vi "TI cDAQ.vi"() -> ()   [LabVIEW 2023]
uses:
  Type Defs and Controls/Graphs Numerics.ctl
  Type Defs and Controls/Graph Channels.ctl
  Type Defs and Controls/Sensor List Cluster.ctl
  Type Defs and Controls/Channel Config Screen.ctl
  Type Defs and Controls/Graphs Numerics (Big).ctl
  Type Defs and Controls/Graph Channels (Big).ctl
  Type Defs and Controls/Sensor Config.ctl
  Type Defs and Controls/DAQ Settings.ctl
  Type Defs and Controls/Trigger Stop Method.ctl
  Type Defs and Controls/Log File Type.ctl
  Type Defs and Controls/Channel Config.ctl
  Type Defs and Controls/Header.ctl
  Type Defs and Controls/Graph Settings Type Def.ctl
  Type Defs and Controls/Test Limits.ctl
  Type Defs and Controls/All Part Info.ctl
  Type Defs and Controls/Part Info.ctl
  Type Defs and Controls/Sensor.ctl
  Type Defs and Controls/System Type.ctl
  Type Defs and Controls/System Config.ctl
  Type Defs and Controls/App Config.ctl
  <vilib>/event_ctls.llb/eventvkey.ctl
  <vilib>/Analysis/baseanly.llb/Mean (DBL).vi
  <vilib>/DAQmx/read.llb/DAQmx Read (Analog 2D DBL NChan NSamp).vi
  <vilib>/Utility/file.llb/Read Delimited Spreadsheet (string).vi
  <vilib>/DAQmx/miscellaneous.llb/DAQmx Fill In Error Info.vi
  <userlib>/_OpenG.lib/array/array.llb/Sort 1D Array (String)__ogtk.vi
  <userlib>/_OpenG.lib/array/array.llb/Sort 1D Array (I32)__ogtk.vi
  <vilib>/Analysis/NI_AALBase.lvlib
  Type Defs and Controls/RT FIFO Mode.ctl
  <resource>/objmgr/daqmx.rc
  <vilib>/Utility/config.llb/NI_LVConfig.lvlib
  <userlib>/_OpenG.lib/array/array.llb/openg_array.lvlib
  <userlib>/_OpenG.lib/variantconfig/variantconfig.llb/openg_variant_configuration_file.lvlib
panel:
  in  "Connecting Tab":enum32{"Page 1"}(tab)
  in  "Save":bool
  in  "Revert":bool
  in  "Open File":bool
  in  "Save Data As":bool
  in  "O-Scope Mode":bool
  in  "Limit:":dbl caption="Mb"
  in  "Auto Save":bool=TRUE
  out "Changes Latch":bool=TRUE
  in  "Title Bar":string
  out "In O-scope Mode":bool
  in  "Load Indicator Tab":enum32{"Page 1"}(tab)
  in  "Decoration Tab":enum32{"Page 1", "Page 2"}(tab)
  in  "Main Tab":enum32{" Main", "Configure"}(tab)
  in  "Show Big Data":bool
  in  "Big Data Tab":enum32{"Page 1", "Page 2"}(tab)
  out "Graph Channels (Big)":T1
  out "Graph Numerics (Big)":T2 {"Y1 RT 9" format="%_4f"; "Y1 RT 8" format="%_4f"; "Y1 RT 7" format="%_4f"; "Y1 RT 6" format="%_4f"; "Y1 RT 5" format="%_4f"; "Y1 RT 4" format="%_4f"; "Y1 RT 3" format="%_4f"; "Y1 RT 2" format="%_4f"}
  out "Graph Colors (Big)":T3={"Numeric Text.Colors:BG Color"=16711680, "Numeric Text.Colors:BG Color 2"=16711680, "Numeric Text.Colors:BG Color 3"=16711680, "Numeric Text.Colors:BG Color 4"=16711680, "Numeric Text.Colors:BG Color 5"=16711680, "Numeric Text.Colors:BG Color 6"=16711680, "Numeric Text.Colors:BG Color 7"=16711680, "Numeric Text.Colors:BG Color 8"=16711680}
  in  "Axis Toggle All":bool
  in  "Axis Toggles":T4
  out "Graph 2":sgl[][](graph)
  in  "Play":bool=TRUE
  in  "Pause":bool
  in  "Main Toggle":bool
  in  "Graph Toggles":T4
  out "Graph Numerics":T5 {"Y6 RT 3" format="%_4f"; "Y5 RT 3" format="%_4f"; "Y4 RT 3" format="%_4f"; "Y3 RT 3" format="%_4f"; "Y6 RT 2" format="%_4f"; "Y5 RT 2" format="%_4f"; "Y4 RT 2" format="%_4f"; "Y3 RT 2" format="%_4f"; "Y2 RT 2" format="%_4f"; "Y1 RT 2" format="%_4f"; "Y6 RT" format="%_4f"; "Y5 RT" format="%_4f"; "Y4 RT" format="%_4f"; "Y3 RT" format="%_4f"; "Y2 RT" format="%_4f"; "Y1 RT" format="%_4f"}
  in  "Graph Channels":T6 {"Y5 3" items=["", "diag raw", "9221_AI-02", "9221_AI-03", "9221_AI-04", "9221_AI-05", "9221_AI-06", "9221_AI-07", "FDM Current (Controller)", "PWM Command", "PWM Diagnostic", "Pump Speed", "9205_AI-04", "9205_AI-05", "9205_AI-06", "9205_AI-07", "9205_AI-22A", "9205_AI-23A", "9208_AI-00", "9208_AI-01", "9208_AI-02", "9208_AI-03", "9208_AI-04", "9208_AI-05", "9208_AI-06", "9208_AI-07", "9211-1_TC-00", "9211-1_TC-01", "9211-1_TC-02", "9211-1_TC-03", "9211-2_TC-00", "9211-2_TC-01", "9211-2_TC-02", "9211-2_TC-03"]; "Y6 3" items=["", "diag raw", "9221_AI-02", "9221_AI-03", "9221_AI-04", "9221_AI-05", "9221_AI-06", "9221_AI-07", "FDM Current (Controller)", "PWM Command", "PWM Diagnostic", "Pump Speed", "9205_AI-04", "9205_AI-05", "9205_AI-06", "9205_AI-07", "9205_AI-22A", "9205_AI-23A", "9208_AI-00", "9208_AI-01", "9208_AI-02", "9208_AI-03", "9208_AI-04", "9208_AI-05", "9208_AI-06", "9208_AI-07", "9211-1_TC-00", "9211-1_TC-01", "9211-1_TC-02", "9211-1_TC-03", "9211-2_TC-00", "9211-2_TC-01", "9211-2_TC-02", "9211-2_TC-03"]; "Y3 3" items=["", "diag raw", "9221_AI-02", "9221_AI-03", "9221_AI-04", "9221_AI-05", "9221_AI-06", "9221_AI-07", "FDM Current (Controller)", "PWM Command", "PWM Diagnostic", "Pump Speed", "9205_AI-04", "9205_AI-05", "9205_AI-06", "9205_AI-07", "9205_AI-22A", "9205_AI-23A", "9208_AI-00", "9208_AI-01", "9208_AI-02", "9208_AI-03", "9208_AI-04", "9208_AI-05", "9208_AI-06", "9208_AI-07", "9211-1_TC-00", "9211-1_TC-01", "9211-1_TC-02", "9211-1_TC-03", "9211-2_TC-00", "9211-2_TC-01", "9211-2_TC-02", "9211-2_TC-03"]; "Y4 3" items=["", "diag raw", "9221_AI-02", "9221_AI-03", "9221_AI-04", "9221_AI-05", "9221_AI-06", "9221_AI-07", "FDM Current (Controller)", "PWM Command", "PWM Diagnostic", "Pump Speed", "9205_AI-04", "9205_AI-05", "9205_AI-06", "9205_AI-07", "9205_AI-22A", "9205_AI-23A", "9208_AI-00", "9208_AI-01", "9208_AI-02", "9208_AI-03", "9208_AI-04", "9208_AI-05", "9208_AI-06", "9208_AI-07", "9211-1_TC-00", "9211-1_TC-01", "9211-1_TC-02", "9211-1_TC-03", "9211-2_TC-00", "9211-2_TC-01", "9211-2_TC-02", "9211-2_TC-03"]; "Y5 2" items=["", "diag raw", "9221_AI-02", "9221_AI-03", "9221_AI-04", "9221_AI-05", "9221_AI-06", "9221_AI-07", "FDM Current (Controller)", "PWM Command", "PWM Diagnostic", "Pump Speed", "9205_AI-04", "9205_AI-05", "9205_AI-06", "9205_AI-07", "9205_AI-22A", "9205_AI-23A", "9208_AI-00", "9208_AI-01", "9208_AI-02", "9208_AI-03", "9208_AI-04", "9208_AI-05", "9208_AI-06", "9208_AI-07", "9211-1_TC-00", "9211-1_TC-01", "9211-1_TC-02", "9211-1_TC-03", "9211-2_TC-00", "9211-2_TC-01", "9211-2_TC-02", "9211-2_TC-03"]; "Y6 2" items=["", "diag raw", "9221_AI-02", "9221_AI-03", "9221_AI-04", "9221_AI-05", "9221_AI-06", "9221_AI-07", "FDM Current (Controller)", "PWM Command", "PWM Diagnostic", "Pump Speed", "9205_AI-04", "9205_AI-05", "9205_AI-06", "9205_AI-07", "9205_AI-22A", "9205_AI-23A", "9208_AI-00", "9208_AI-01", "9208_AI-02", "9208_AI-03", "9208_AI-04", "9208_AI-05", "9208_AI-06", "9208_AI-07", "9211-1_TC-00", "9211-1_TC-01", "9211-1_TC-02", "9211-1_TC-03", "9211-2_TC-00", "9211-2_TC-01", "9211-2_TC-02", "9211-2_TC-03"]; "Y3 2" items=["", "diag raw", "9221_AI-02", "9221_AI-03", "9221_AI-04", "9221_AI-05", "9221_AI-06", "9221_AI-07", "FDM Current (Controller)", "PWM Command", "PWM Diagnostic", "Pump Speed", "9205_AI-04", "9205_AI-05", "9205_AI-06", "9205_AI-07", "9205_AI-22A", "9205_AI-23A", "9208_AI-00", "9208_AI-01", "9208_AI-02", "9208_AI-03", "9208_AI-04", "9208_AI-05", "9208_AI-06", "9208_AI-07", "9211-1_TC-00", "9211-1_TC-01", "9211-1_TC-02", "9211-1_TC-03", "9211-2_TC-00", "9211-2_TC-01", "9211-2_TC-02", "9211-2_TC-03"]; "Y4 2" items=["", "diag raw", "9221_AI-02", "9221_AI-03", "9221_AI-04", "9221_AI-05", "9221_AI-06", "9221_AI-07", "FDM Current (Controller)", "PWM Command", "PWM Diagnostic", "Pump Speed", "9205_AI-04", "9205_AI-05", "9205_AI-06", "9205_AI-07", "9205_AI-22A", "9205_AI-23A", "9208_AI-00", "9208_AI-01", "9208_AI-02", "9208_AI-03", "9208_AI-04", "9208_AI-05", "9208_AI-06", "9208_AI-07", "9211-1_TC-00", "9211-1_TC-01", "9211-1_TC-02", "9211-1_TC-03", "9211-2_TC-00", "9211-2_TC-01", "9211-2_TC-02", "9211-2_TC-03"]; "Y2 2" items=["", "diag raw", "9221_AI-02", "9221_AI-03", "9221_AI-04", "9221_AI-05", "9221_AI-06", "9221_AI-07", "FDM Current (Controller)", "PWM Command", "PWM Diagnostic", "Pump Speed", "9205_AI-04", "9205_AI-05", "9205_AI-06", "9205_AI-07", "9205_AI-22A", "9205_AI-23A", "9208_AI-00", "9208_AI-01", "9208_AI-02", "9208_AI-03", "9208_AI-04", "9208_AI-05", "9208_AI-06", "9208_AI-07", "9211-1_TC-00", "9211-1_TC-01", "9211-1_TC-02", "9211-1_TC-03", "9211-2_TC-00", "9211-2_TC-01", "9211-2_TC-02", "9211-2_TC-03"]; "Y1 2" items=["", "diag raw", "9221_AI-02", "9221_AI-03", "9221_AI-04", "9221_AI-05", "9221_AI-06", "9221_AI-07", "FDM Current (Controller)", "PWM Command", "PWM Diagnostic", "Pump Speed", "9205_AI-04", "9205_AI-05", "9205_AI-06", "9205_AI-07", "9205_AI-22A", "9205_AI-23A", "9208_AI-00", "9208_AI-01", "9208_AI-02", "9208_AI-03", "9208_AI-04", "9208_AI-05", "9208_AI-06", "9208_AI-07", "9211-1_TC-00", "9211-1_TC-01", "9211-1_TC-02", "9211-1_TC-03", "9211-2_TC-00", "9211-2_TC-01", "9211-2_TC-02", "9211-2_TC-03"]}
  in  "Graph Range":T7(ring)=enum."10"
  out "Graph 1":sgl[][](graph)
  in  "Synch Files":bool
  in  "Import from CSV":bool
  in  "Log Min":bool
  in  "Log Sec":bool=TRUE
  in  "Hide Trig Ch":bool
  in  "Hide Trig Val":bool
  in  "Hide Trig Samples":bool
  in  "Hide Trig Stop":bool
  in  "Hide Trig Int":bool
  in  "Hide Pretrig Smpls":bool
  in  "Save Mode":T8(ring)
  in  "Sample Min":bool
  in  "Sample Sec":bool=TRUE
  in  "Delete Sensor":bool
  in  "Add Sensor":bool
  in  "Trigger Stop Method":T9(ring)=enum."Use Threshold to Stop Trigger"
  in  "Hours":bool
  in  "Minutes":bool=TRUE
  in  "Trigger Type":T10(ring)
  in  "Sensors":T11=[{"Channel"="9221_AI-00", "Description"="test", "Acquire"=TRUE, "Sensor"="Pressure Sensor", "Chg Sensor"=FALSE, "Cal Date"="12/31/1903", "Offset"=-0.0, "Span"=10.0, "Cal"=FALSE, "Test Limits"=FALSE, "Type"="0-60 VDC", "Data Index"=0}, {"Channel"="9221_AI-01", "Description"="", "Acquire"=FALSE, "Sensor"="None Selected", "Chg Sensor"=FALSE, "Cal Date"="---------", "Offset"=0.0, "Span"=0.0, "Cal"=FALSE, "Test Limits"=FALSE, "Type"="0-60 VDC", "Data Index"=1}, {"Channel"="9221_AI-02", "Description"="", "Acquire"=FALSE, "Sensor"="None Selected", "Chg Sensor"=FALSE, "Cal Date"="---------", "Offset"=0.0, "Span"=0.0, "Cal"=FALSE, "Test Limits"=FALSE, "Type"="0-60 VDC", "Data Index"=2}, {"Channel"="9221_AI-03", "Description"="", "Acquire"=FALSE, "Sensor"="None Selected", "Chg Sensor"=FALSE, "Cal Date"="---------", "Offset"=0.0, "Span"=0.0, "Cal"=FALSE, "Test Limits"=FALSE, "Type"="0-60 VDC", "Data Index"=3}, {"Channel"="9221_AI-04", "Description"="", "Acquire"=FALSE, "Sensor"="None Selected", "Chg Sensor"=FALSE, "Cal Date"="---------", "Offset"=0.0, "Span"=0.0, "Cal"=FALSE, "Test Limits"=FALSE, "Type"="0-60 VDC", "Data Index"=4}, {"Channel"="9221_AI-05", "Description"="", "Acquire"=FALSE, "Sensor"="None Selected", "Chg Sensor"=FALSE, "Cal Date"="---------", "Offset"=0.0, "Span"=0.0, "Cal"=FALSE, "Test Limits"=FALSE, "Type"="0-60 VDC", "Data Index"=5}, {"Channel"="9221_AI-06", "Description"="", "Acquire"=FALSE, "Sensor"="None Selected", "Chg Sensor"=FALSE, "Cal Date"="---------", "Offset"=0.0, "Span"=0.0, "Cal"=FALSE, "Test Limits"=FALSE, "Type"="0-60 VDC", "Data Index"=6}, {"Channel"="9221_AI-07", "Description"="", "Acquire"=FALSE, "Sensor"="None Selected", "Chg Sensor"=FALSE, "Cal Date"="---------", "Offset"=0.0, "Span"=0.0, "Cal"=FALSE, "Test Limits"=FALSE, "Type"="0-60 VDC", "Data Index"=7}, {"Channel"="9205_AI-00", "Description"="", "Acquire"=FALSE, "Sensor"="None Selected", "Chg Sensor"=FALSE, "Cal Date"="---------", "Offset"=0.0, "Span"=0.0, "Cal"=FALSE, "Test Limits"=FALSE, "Type"="0-10 VDC", "Data Index"=8}, {"Channel"="9205_AI-01", "Description"="", "Acquire"=FALSE, "Sensor"="None Selected", "Chg Sensor"=FALSE, "Cal Date"="---------", "Offset"=0.0, "Span"=0.0, "Cal"=FALSE, "Test Limits"=FALSE, "Type"="0-10 VDC", "Data Index"=9}, {"Channel"="9205_AI-02", "Description"="", "Acquire"=FALSE, "Sensor"="None Selected", "Chg Sensor"=FALSE, "Cal Date"="---------", "Offset"=0.0, "Span"=0.0, "Cal"=FALSE, "Test Limits"=FALSE, "Type"="0-10 VDC", "Data Index"=10}, {"Channel"="9205_AI-03", "Description"="", "Acquire"=FALSE, "Sensor"="None Selected", "Chg Sensor"=FALSE, "Cal Date"="---------", "Offset"=0.0, "Span"=0.0, "Cal"=FALSE, "Test Limits"=FALSE, "Type"="0-10 VDC", "Data Index"=11}, {"Channel"="9205_AI-04", "Description"="", "Acquire"=FALSE, "Sensor"="None Selected", "Chg Sensor"=FALSE, "Cal Date"="---------", "Offset"=0.0, "Span"=0.0, "Cal"=FALSE, "Test Limits"=FALSE, "Type"="0-10 VDC", "Data Index"=12}, {"Channel"="9205_AI-05", "Description"="", "Acquire"=FALSE, "Sensor"="None Selected", "Chg Sensor"=FALSE, "Cal Date"="---------", "Offset"=0.0, "Span"=0.0, "Cal"=FALSE, "Test Limits"=FALSE, "Type"="0-10 VDC", "Data Index"=13}, {"Channel"="9205_AI-06", "Description"="", "Acquire"=FALSE, "Sensor"="None Selected", "Chg Sensor"=FALSE, "Cal Date"="---------", "Offset"=0.0, "Span"=0.0, "Cal"=FALSE, "Test Limits"=FALSE, "Type"="0-10 VDC", "Data Index"=14}, {"Channel"="9205_AI-07", "Description"="", "Acquire"=FALSE, "Sensor"="None Selected", "Chg Sensor"=FALSE, "Cal Date"="---------", "Offset"=0.0, "Span"=0.0, "Cal"=FALSE, "Test Limits"=FALSE, "Type"="0-10 VDC", "Data Index"=15}, {"Channel"="9208_AI-00", "Description"="", "Acquire"=FALSE, "Sensor"="None Selected", "Chg Sensor"=FALSE, "Cal Date"="---------", "Offset"=0.0, "Span"=0.0, "Cal"=FALSE, "Test Limits"=FALSE, "Type"="0-20 mA", "Data Index"=16}, {"Channel"="9208_AI-01", "Description"="", "Acquire"=FALSE, "Sensor"="None Selected", "Chg Sensor"=FALSE, "Cal Date"="---------", "Offset"=0.0, "Span"=0.0, "Cal"=FALSE, "Test Limits"=FALSE, "Type"="0-20 mA", "Data Index"=17}, {"Channel"="9208_AI-02", "Description"="", "Acquire"=FALSE, "Sensor"="None Selected", "Chg Sensor"=FALSE, "Cal Date"="---------", "Offset"=0.0, "Span"=0.0, "Cal"=FALSE, "Test Limits"=FALSE, "Type"="0-20 mA", "Data Index"=18}, {"Channel"="9208_AI-03", "Description"="", "Acquire"=FALSE, "Sensor"="None Selected", "Chg Sensor"=FALSE, "Cal Date"="---------", "Offset"=0.0, "Span"=0.0, "Cal"=FALSE, "Test Limits"=FALSE, "Type"="0-20 mA", "Data Index"=19}, {"Channel"="9208_AI-04", "Description"="", "Acquire"=FALSE, "Sensor"="None Selected", "Chg Sensor"=FALSE, "Cal Date"="---------", "Offset"=0.0, "Span"=0.0, "Cal"=FALSE, "Test Limits"=FALSE, "Type"="0-20 mA", "Data Index"=20}, {"Channel"="9208_AI-05", "Description"="", "Acquire"=FALSE, "Sensor"="None Selected", "Chg Sensor"=FALSE, "Cal Date"="---------", "Offset"=0.0, "Span"=0.0, "Cal"=FALSE, "Test Limits"=FALSE, "Type"="0-20 mA", "Data Index"=21}, {"Channel"="9208_AI-06", "Description"="", "Acquire"=FALSE, "Sensor"="None Selected", "Chg Sensor"=FALSE, "Cal Date"="---------", "Offset"=0.0, "Span"=0.0, "Cal"=FALSE, "Test Limits"=FALSE, "Type"="0-20 mA", "Data Index"=22}, {"Channel"="9208_AI-07", "Description"="", "Acquire"=FALSE, "Sensor"="None Selected", "Chg Sensor"=FALSE, "Cal Date"="---------", "Offset"=0.0, "Span"=0.0, "Cal"=FALSE, "Test Limits"=FALSE, "Type"="0-20 mA", "Data Index"=23}, {"Channel"="9211_TC-00", "Description"="", "Acquire"=FALSE, "Sensor"="None Selected", "Chg Sensor"=FALSE, "Cal Date"="---------", "Offset"=0.0, "Span"=0.0, "Cal"=FALSE, "Test Limits"=FALSE, "Type"="T-Type", "Data Index"=24}, {"Channel"="9211_TC-01", "Description"="", "Acquire"=FALSE, "Sensor"="None Selected", "Chg Sensor"=FALSE, "Cal Date"="---------", "Offset"=0.0, "Span"=0.0, "Cal"=FALSE, "Test Limits"=FALSE, "Type"="T-Type", "Data Index"=25}, {"Channel"="9211_TC-02", "Description"="", "Acquire"=FALSE, "Sensor"="None Selected", "Chg Sensor"=FALSE, "Cal Date"="---------", "Offset"=0.0, "Span"=0.0, "Cal"=FALSE, "Test Limits"=FALSE, "Type"="T-Type", "Data Index"=26}, {"Channel"="9211_TC-03", "Description"="", "Acquire"=FALSE, "Sensor"="None Selected", "Chg Sensor"=FALSE, "Cal Date"="---------", "Offset"=0.0, "Span"=0.0, "Cal"=FALSE, "Test Limits"=FALSE, "Type"="T-Type", "Data Index"=27}]
  in  "DAQ Table":string[][](table)=[[""], ["test"], ["50.000"], ["5"], ["0"], ["1.000"], [""], ["10"], ["1"]]
  out "Config Name:":string="test.cfg"
  in  "Open":bool
  in  "Save As":bool
  in  "Title Tab":enum32{"Page 1", "Page 2"}(tab)
  out "Title":string="TI cDAQ, Debug"
  out "Date":string="4/23/2020"
  out "Time":string="11:18:09 AM"
  in  "Mode Exit":bool
  out "Status":string="IN DATA VIEW MODE..."
  in  "Acquiring Tab":enum32{"Page 1"}(tab)
  in  "Control Tab":enum32{"Page 1", "Page 2"}(tab)
  in  "Disarm DAQ":bool
  in  "Arm DAQ":bool
  out "DAQ Armed":bool
  in  "Start Log":bool
  out "Acquiring Data 2":bool
  in  "Stop DAQ":bool
  in  "Header Table:":string[][](table)=[[""], [""], [""], [""]] caption="Header Table"
  in  "Data Base Path:":path=path "C:/Data"
  out "Elapsed Time:":dbl format="%<%H:%M:%S>t"
  out "Start of Test:":timestamp format="%<%x %X>T"
  out "Samples Recorded:":u32 format="%#.0f"
  in  "Add Data Point":bool
  # "Connecting\nto cDAQ"
  # "samples /"
  # "*This includes the Sensor/Cal file,\nand Config files."
  # "samples /"
  # "Channel"
  # "Type"
  # "Acquire"
  # "Name"
  # "Sensor"
  # "Cal Date"
  # "Zero"
  # "Span"
  # "Logging\nData"
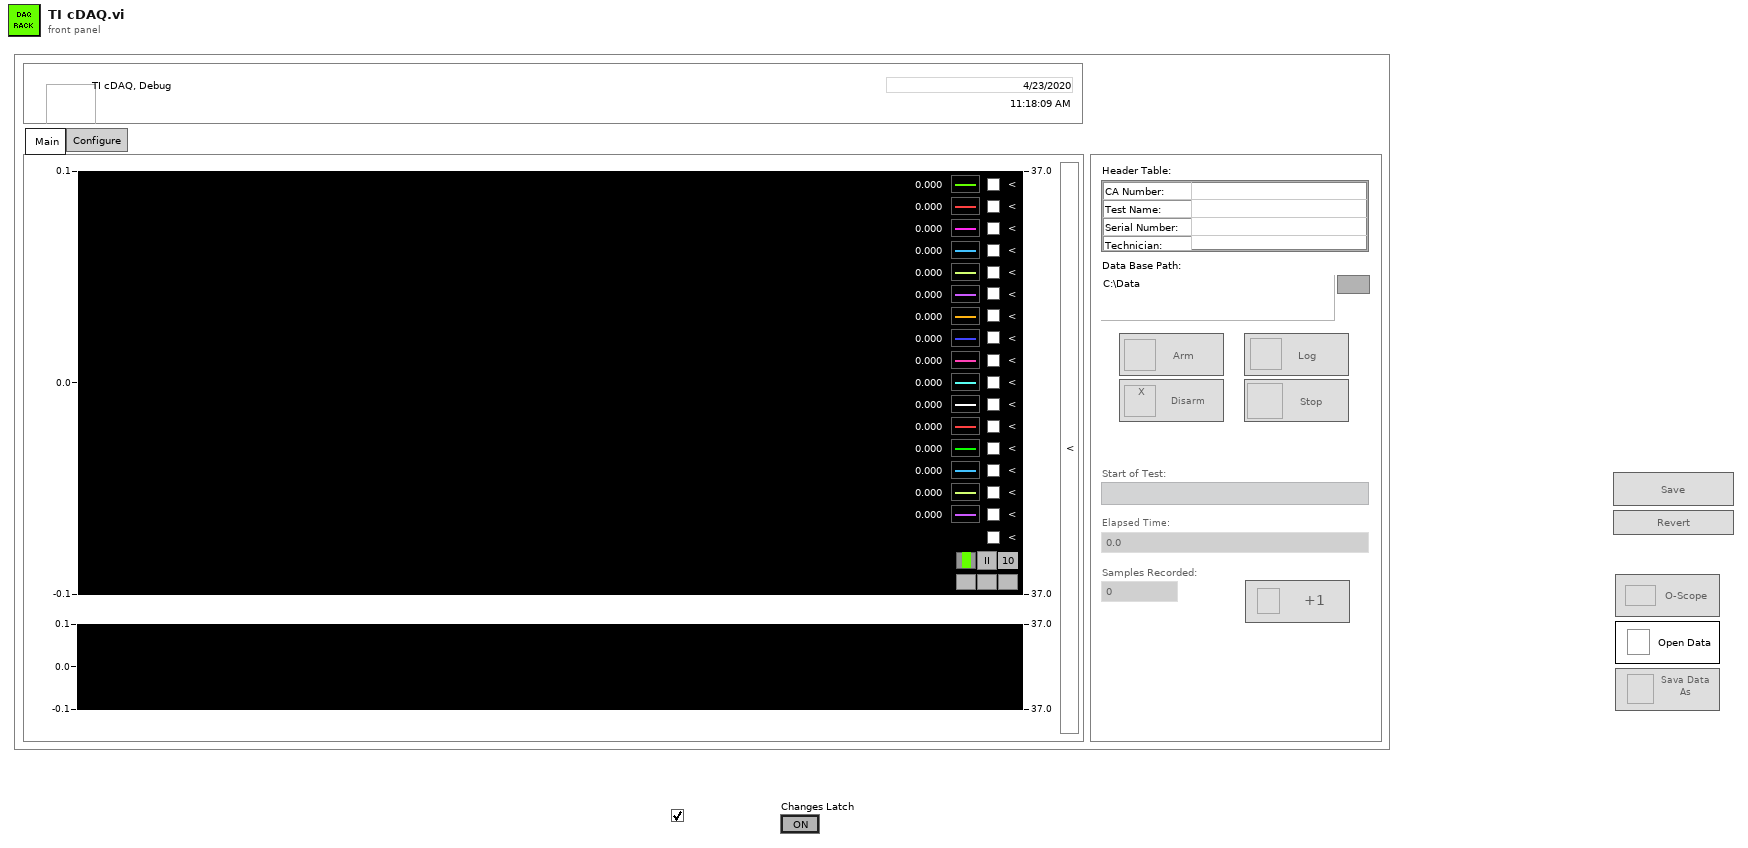
[diagram p1: front panel]
types:
  T1 = typedef "Graph Channels (Big).ctl" = cluster{"String":string, "String 2":string, "String 3":string, "String 4":string, "String 5":string, "String 6":string, "String 7":string, "String 8":string}
  T2 = typedef "Graphs Numerics (Big).ctl" = cluster{"Y1 RT 2":dbl, "Y1 RT 3":dbl, "Y1 RT 4":dbl, "Y1 RT 5":dbl, "Y1 RT 6":dbl, "Y1 RT 7":dbl, "Y1 RT 8":dbl, "Y1 RT 9":dbl}
  T3 = cluster{"Numeric Text.Colors:BG Color":u32, "Numeric Text.Colors:BG Color 2":u32, "Numeric Text.Colors:BG Color 3":u32, "Numeric Text.Colors:BG Color 4":u32, "Numeric Text.Colors:BG Color 5":u32, "Numeric Text.Colors:BG Color 6":u32, "Numeric Text.Colors:BG Color 7":u32, "Numeric Text.Colors:BG Color 8":u32}
  T4 = cluster{"Boolean":bool, "Boolean 2":bool, "Boolean 3":bool, "Boolean 4":bool, "Boolean 5":bool, "Boolean 6":bool, "Boolean 7":bool, "Boolean 8":bool, "Boolean 9":bool, "Boolean 10":bool, "Boolean 11":bool, "Boolean 12":bool, "Boolean 13":bool, "Boolean 14":bool, "Boolean 15":bool, "Boolean 16":bool}
  T5 = typedef "Graphs Numerics.ctl" = cluster{"Y1 RT":dbl, "Y2 RT":dbl, "Y3 RT":dbl, "Y4 RT":dbl, "Y5 RT":dbl, "Y6 RT":dbl, "Y1 RT 2":dbl, "Y2 RT 2":dbl, "Y3 RT 2":dbl, "Y4 RT 2":dbl, "Y5 RT 2":dbl, "Y6 RT 2":dbl, "Y3 RT 3":dbl, "Y4 RT 3":dbl, "Y5 RT 3":dbl, "Y6 RT 3":dbl}
  T6 = typedef "Graph Channels.ctl" = cluster{"Y1":u16, "Y2":u16, "Y3":u16, "Y4":u16, "Y5":u16, "Y6":u16, "Y1 2":u16, "Y2 2":u16, "Y3 2":u16, "Y4 2":u16, "Y5 2":u16, "Y6 2":u16, "Y3 3":u16, "Y4 3":u16, "Y5 3":u16, "Y6 3":u16}
  T7 = enum16{"1", "2", "3", "4", "5", "10", "15", "30", "60"}
  T8 = enum16{"Single File", "Segmented Files", "New File at Midnight"}
  T9 = enum16{"Use Samples Value to Stop Trigger", "Use Threshold to Stop Trigger"}
  T10 = enum16{"Manual", "Timed", "Analog Rising", "Analog Falling"}
  T11 = typedef "Sensor List Cluster.ctl" = T12[]
  T12 = typedef "Channel Config Screen.ctl" = cluster{"Channel":string, "Description":string, "Acquire":bool, "Sensor":string, "Chg Sensor":bool, "Cal Date":string, "Offset":dbl, "Span":dbl, "Cal":bool, "Test Limits":bool, "Type":string, "Data Index":u32}
  T13 = typedef "App Config.ctl" = cluster{"Support Dir (Local)":path, "Support Dir (Remote)":path, "Config Sub Dir":string, "Last Config (Std)":string, "Last Config (Def)":string, "Last Config (8TC)":string}
  T14 = typedef "System Config.ctl" = cluster{"System":string, "Description":string}
  T15 = typedef "System Type.ctl" = enum16{"Standard", "Deformation", "Standard 8TC"}
  T16 = typedef "Sensor Config.ctl" = cluster{"DAQ Settings":T17, "Channels":T20[], "Header":T21, "Graph Settings":T22, "Test Limits":T23[], "All Type Info":T24, "Save Mode":enum16{"Single File", "Segmented Files", "New File at Midnight"}, "Data Base Path":path}
  T17 = typedef "DAQ Settings.ctl" = cluster{"Trigger Type":enum16{"Manual", "Timed", "Analog Rising", "Analog Falling"}, "Trigger Samples":i32, "Pretrigger Samples":i32, "Trigger Interval":dbl, "Time Units":bool, "Auto Save":bool, "Sample Rate":dbl, "Select Analog":bool, "Trigger Value":dbl, "Trigger Stop Method":T18, "Rate Sec/Min":bool, "Save Mode":enum16{"Single File", "Segmented Files", "New File at Midnight"}, "File Size Limit":dbl, "Log File Type":T19, "Trigger Data Index":u32, "Log Rate":dbl, "Rate Sec/Min (Log)":bool, "Sample Rate (S/s)":dbl, "Log Rate (S/s)":dbl}
  T18 = typedef "Trigger Stop Method.ctl" = enum16{"Use Samples Value to Stop Trigger", "Use Threshold to Stop Trigger"}
  T19 = typedef "Log File Type.ctl" = enum16{"Basic", "RTS"}
  T20 = typedef "Channel Config.ctl" = cluster{"Channel":string, "Type":string, "Acquire":bool, "Name":string, "Sensor":string, "Data Index":u32}
  T21 = typedef "Header.ctl" = cluster{"CA Number":string, "Test Name":string, "Serial Number":string, "Technician":string}
  T22 = typedef "Graph Settings Type Def.ctl" = cluster{"Graph Labels":string[], u8[], i16[], u32[], u8[], u8[], u8[], u32[], u8[], u8[], u8[], dbl[], dbl[], "Graph Toggles":bool[], "Axis Toggles":bool[], "Graph Range":enum16{"1", "2", "3", "4", "5", "10", "15", "30", "60"}}
  T23 = typedef "Test Limits.ctl" = cluster{"Channel Acquired?":bool, "RMS?":bool, "Pk-Pk":bool, "Frequency":bool, "EU High Limit 1":dbl, "EU Low Limit 1":dbl, "EU High Limit 2":dbl, "EU Low Limit 2":dbl, "RMS High Limit":dbl, "RMS Low Limit":dbl, "Pk-Pk High Limit ":dbl, "Pk-Pk Low Limit":dbl, "Frequency High Limit":dbl, "Frequency Low Limit":dbl}
  T24 = typedef "All Part Info.ctl" = cluster{"Type Name":string, "Type Signal Names":string[], "# Signals":i32, "# Parts":i32, "Part Info":T25[]}[]
  T25 = typedef "Part Info.ctl" = cluster{"Part Number":string, "Channel Indexes":u16[], "Enabled?":bool}
  T26 = typedef "Sensor.ctl" = cluster{"Sensor Name":string, "Sensor Info":cluster{"Manufacturer":string, "Model":string, "Serial Number":string}, "Last Cal Info":cluster{"Last Calibration Date":dbl, "Calibrator":string, "Cal Duration":i32}, "Voltage Range":cluster{"High Limit":dbl, "Low Limit":dbl}, "EGU Range":cluster{"High Limit":dbl, "Low Limit":dbl}, "Units":string, "Calibration Type":enum16{"Calibrate Analog", "Compare Analog Calibration"}, "EGU List":dbl[], "Voltage List":dbl[], "Coefficients":dbl[], "Order":i32, "Algorithm":enum32{"SVD", "Givens", "Givens2", "Householder", "LU Decomposition", "Cholesky"}, "Max Error % of Full Scale":dbl, "Max Mean Squared Error":dbl, "Use Error %":bool, "Use MSE":bool, "Allow Manual Entry":bool, "Max Stability Error":dbl, "Max Error % of Reading":dbl, "Use Error % of Reading":bool}
  T27 = cluster{"Sensor Name":string, "Sensor Info":cluster{"Manufacturer":string, "Model":string, "Serial Number":string}, "Last Cal Info":cluster{"Last Calibration Date":dbl, "Calibrator":string, "Cal Duration":i32}, "Voltage Range":cluster{"High Limit":dbl, "Low Limit":dbl}, "EGU Range":cluster{"High Limit":dbl, "Low Limit":dbl}, "Units":string, "Calibration Type":enum16{"Calibrate Analog", "Compare Analog Calibration"}, "EGU List":dbl[], "Voltage List":dbl[], "Coefficients":dbl[], "Order":i32, "Algorithm":enum32{"SVD", "Givens", "Givens2", "Householder", "LU Decomposition", "Cholesky"}, "Max Error % of Full Scale":dbl, "Max Mean Squared Error":dbl, "Use Error %":bool, "Use MSE":bool, "Allow Manual Entry":bool, "Max Stability Error":dbl, "Max Error % of Reading":dbl, "Use Error % of Reading":bool}[]
  T28 = cluster{"Virtual Trigger":bool, "Interval":dbl, "Trigger Armed":bool, "Acquiring Data":bool, "Channel Filter":bool[], "Error":errorcluster, "Data":sgl[][], "Trigger Index":i32, "App Path":path, "Config Dir":path, "Config":T16, "Channel Addresses":string[], "Scaling":cluster{"Sensor Name":string, "Sensor Info":cluster{"Manufacturer":string, "Model":string, "Serial Number":string}, "Last Cal Info":cluster{"Last Calibration Date":dbl, "Calibrator":string, "Cal Duration":i32}, "Voltage Range":cluster{"High Limit":dbl, "Low Limit":dbl}, "EGU Range":cluster{"High Limit":dbl, "Low Limit":dbl}, "Units":string, "Calibration Type":enum16{"Calibrate Analog", "Compare Analog Calibration"}, "EGU List":dbl[], "Voltage List":dbl[], "Coefficients":dbl[], "Order":i32, "Algorithm":enum32{"SVD", "Givens", "Givens2", "Householder", "LU Decomposition", "Cholesky"}, "Max Error % of Full Scale":dbl, "Max Mean Squared Error":dbl, "Use Error %":bool, "Use MSE":bool, "Allow Manual Entry":bool, "Max Stability Error":dbl, "Max Error % of Reading":dbl, "Use Error % of Reading":bool}[], "File Created?":bool, "Saving Path":path, "Previous Time":dbl, "New Time":dbl, "Calibration Path":path, "AI Task":refnum<k21>, "Graph Ch Refs":refnum<vi>[], "Pause Graph":bool, "Force Update":bool, "Data File Path":path, "Buffer Size":u32, "UnPause Once":bool, "O-Scope Mode":bool, "Data View Mode":bool, "Midnight Check":timestamp, "Start Timestamp":timestamp, "Time Offset":dbl, "Pretrigger Size":i32, "Midnight Rollover":bool, "Segment File":bool, "Total Channel Count":i16, "DO Task":refnum<k21>, "DI Task":refnum<k21>, "timer":u32, "App Config Path":path, "Title Bar":refnum<vi>, "Connected Timer":u32, "Last SN":string, "Acquire Data":bool, "Channel Select":i32, "Channel Display":T11, "Sensors":T26[], "Config Saved":T16, "Changes?":bool, "Revert":bool, "DAQ Running":bool, "Load Prompt":bool, "Samples Recorded":u32, "System Type":T15, "Samples Acquired":u32, "Data Log Indicies":i32[], "System Ref":tag, "Selected System":T14, "Config Extension":string, "App Config":T13, "Config Name":string, "Sensor File Name":string, "Sys Cfg File Name":string, "Add Data Point":bool, "Manual Data Mode":bool, "Log Path Ref":refnum<file>}
  T29 = typedef "eventvkey.ctl" = enum16{"ASCII", "Enter", "Return", "Shift", "Ctrl", "Alt", "Cmd", "Opt", "Caps", "NumLock", "Clear", "Break", "Up", "Down", "Left", "Right", "Insert", "Delete", "Home", "End", "PageUp", "PageDown", "Escape", "Help", "Pause", "ScrollLock", "F1", "F2", "F3", "F4", "F5", "F6", "F7", "F8", "F9", "F10", "F11", "F12", "F13", "F14", "F15", "F16", "F17", "F18", "F19", "F20", "F21", "F22", "F23", "F24", "Play", "VolumeUp", "VolumeDown", "Mute", "Two Byte Char"}
  T30 = enum8{"Enabled", "Disabled", "Disabled and Grayed Out"}
  T31 = enum32{"Page Enabled", "Page Disabled", "Page Disabled & Grayed"}
  T32 = typedef "RT FIFO Mode.ctl" = enum16{"Create", "Write", "Read", "Delete"}
  T33 = cluster{"[0]":bool, "[1]":bool, "[2]":bool, "[3]":bool, "[4]":bool, "[5]":bool, "[6]":bool, "[7]":bool, "[8]":bool, "[9]":bool, "[10]":bool, "[11]":bool, "[12]":bool, "[13]":bool, "[14]":bool, "[15]":bool}
  T34 = typedef "LVRowAndColumnTypeDef.ctl" = cluster{"Row":i32, "Column":i32}
  T35 = cluster{"Header Table:[0]":string, "Header Table:[1]":string, "Header Table:[2]":string, "Header Table:[3]":string}
  T36 = typedef "LVPoint32TypeDef.ctl" = cluster{"Horizontal":i32, "Vertical":i32}
  T37 = cluster{"[0]":string, "[1]":string, "[2]":string, "[3]":string, "[4]":string, "[5]":string, "[6]":string, "[7]":string}
  T38 = enum32{"invalid app kind", "Development System", "Run Time System", "Student Edition", "Embedded LabVIEW", "Evaluation", "Custom"}
  T39 = typedef "NI_LVConfig.lvlib/Config Data RefNum.ctl" = refnum<k1>
  T40 = cluster{"[0]":dbl, "[1]":dbl, "[2]":dbl, "[3]":dbl, "[4]":dbl, "[5]":dbl, "[6]":dbl, "[7]":dbl, "[8]":dbl, "[9]":dbl, "[10]":dbl, "[11]":dbl, "[12]":dbl, "[13]":dbl, "[14]":dbl, "[15]":dbl}
  T41 = cluster{"[0]":dbl, "[1]":dbl, "[2]":dbl, "[3]":dbl, "[4]":dbl, "[5]":dbl, "[6]":dbl, "[7]":dbl}
  T42 = cluster{"Graph Toggles[0]":bool, "Graph Toggles[1]":bool, "Graph Toggles[2]":bool, "Graph Toggles[3]":bool, "Graph Toggles[4]":bool, "Graph Toggles[5]":bool, "Graph Toggles[6]":bool, "Graph Toggles[7]":bool, "Graph Toggles[8]":bool, "Graph Toggles[9]":bool, "Graph Toggles[10]":bool, "Graph Toggles[11]":bool, "Graph Toggles[12]":bool, "Graph Toggles[13]":bool, "Graph Toggles[14]":bool, "Graph Toggles[15]":bool}
  T43 = cluster{"Axis Toggles[0]":bool, "Axis Toggles[1]":bool, "Axis Toggles[2]":bool, "Axis Toggles[3]":bool, "Axis Toggles[4]":bool, "Axis Toggles[5]":bool, "Axis Toggles[6]":bool, "Axis Toggles[7]":bool, "Axis Toggles[8]":bool, "Axis Toggles[9]":bool, "Axis Toggles[10]":bool, "Axis Toggles[11]":bool, "Axis Toggles[12]":bool, "Axis Toggles[13]":bool, "Axis Toggles[14]":bool, "Axis Toggles[15]":bool}
  T44 = typedef "LVDateTimeRec.ctl" = cluster{"fractional second":dbl, "second":i32, "minute":i32, "hour":i32, "day of month":i32, "month":i32, "year":i32, "day of week":i32, "day of year":i32, "DST":i32}
  T45 = cluster{"Sensor Name":string, "Sensor Info":cluster{"Manufacturer":string, "Model":string, "Serial Number":string}, "Last Cal Info":cluster{"Last Calibration Date":dbl, "Calibrator":string, "Cal Duration":i32}, "Voltage Range":cluster{"High Limit":dbl, "Low Limit":dbl}, "EGU Range":cluster{"High Limit":dbl, "Low Limit":dbl}, "Units":string, "Calibration Type":enum16{"Calibrate Analog", "Compare Analog Calibration"}, "EGU List":dbl[], "Voltage List":dbl[], "Coefficients":dbl[], "Order":i32, "Algorithm":enum32{"SVD", "Givens", "Givens2", "Householder", "LU Decomposition", "Cholesky"}, "Max Error % of Full Scale":dbl, "Max Mean Squared Error":dbl, "Use Error %":bool, "Use MSE":bool, "Allow Manual Entry":bool, "Max Stability Error":dbl, "Max Error % of Reading":dbl, "Use Error % of Reading":bool}
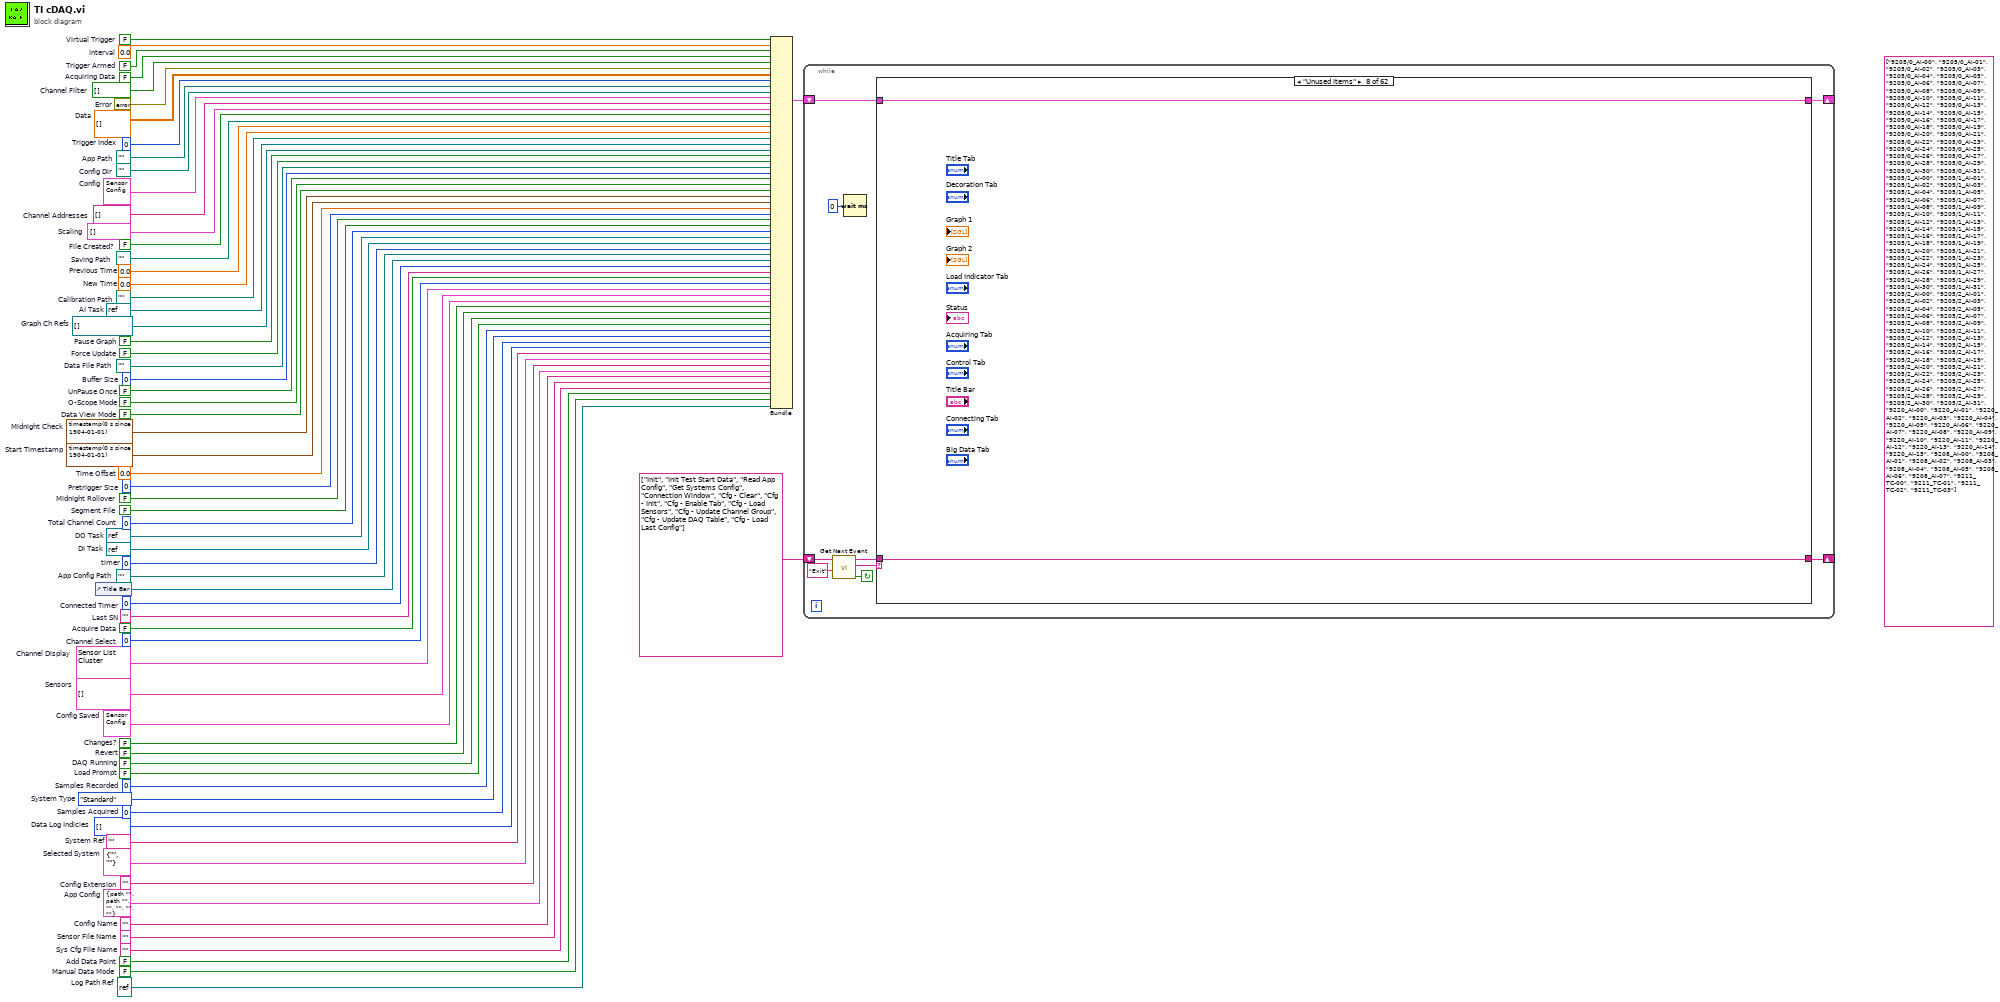
[diagram p0: block diagram]
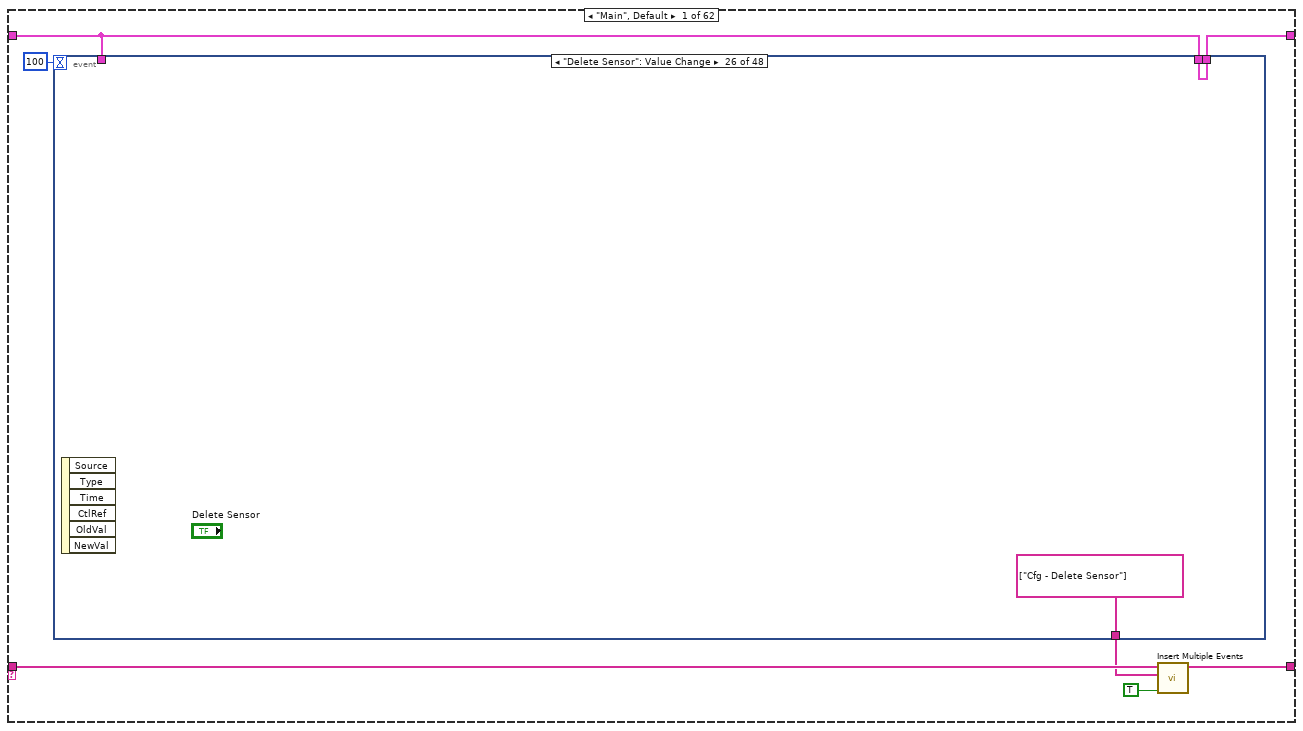
[diagram p2: hidden frame]
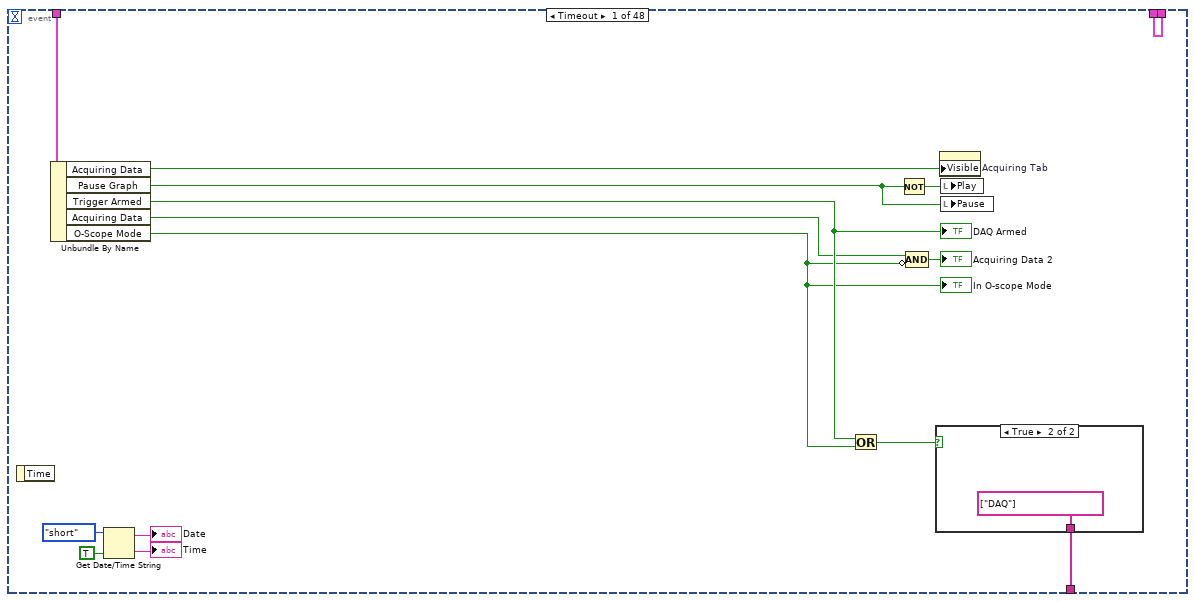
[diagram p3: hidden frame]
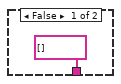
[diagram p4: hidden frame]
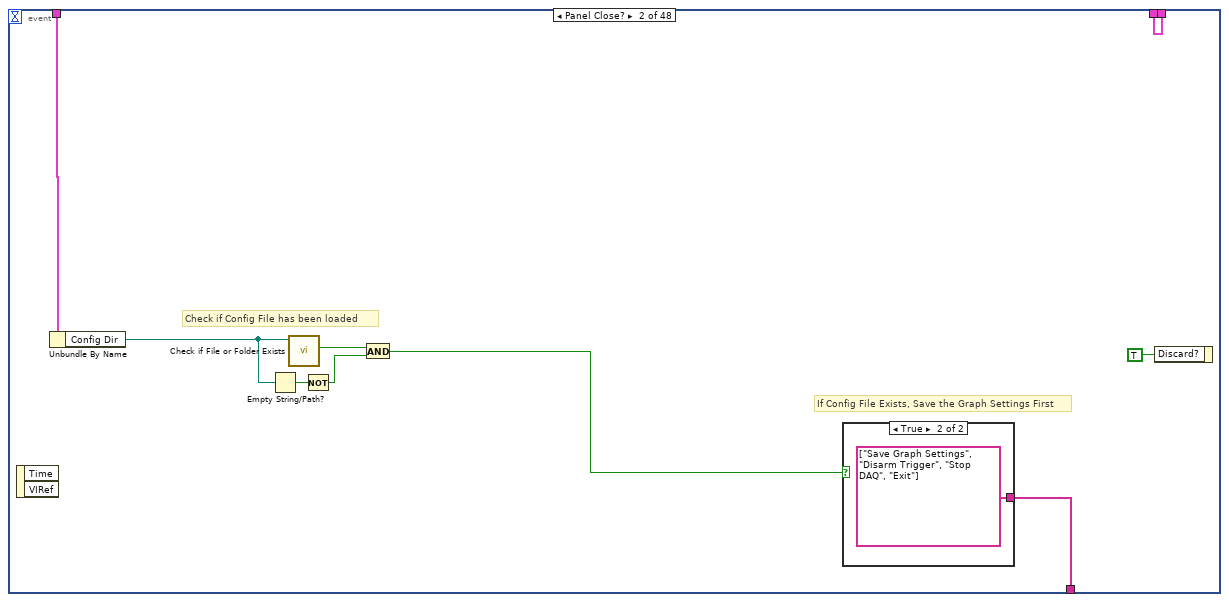
[diagram p5: hidden frame]
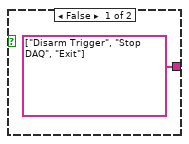
[diagram p6: hidden frame]
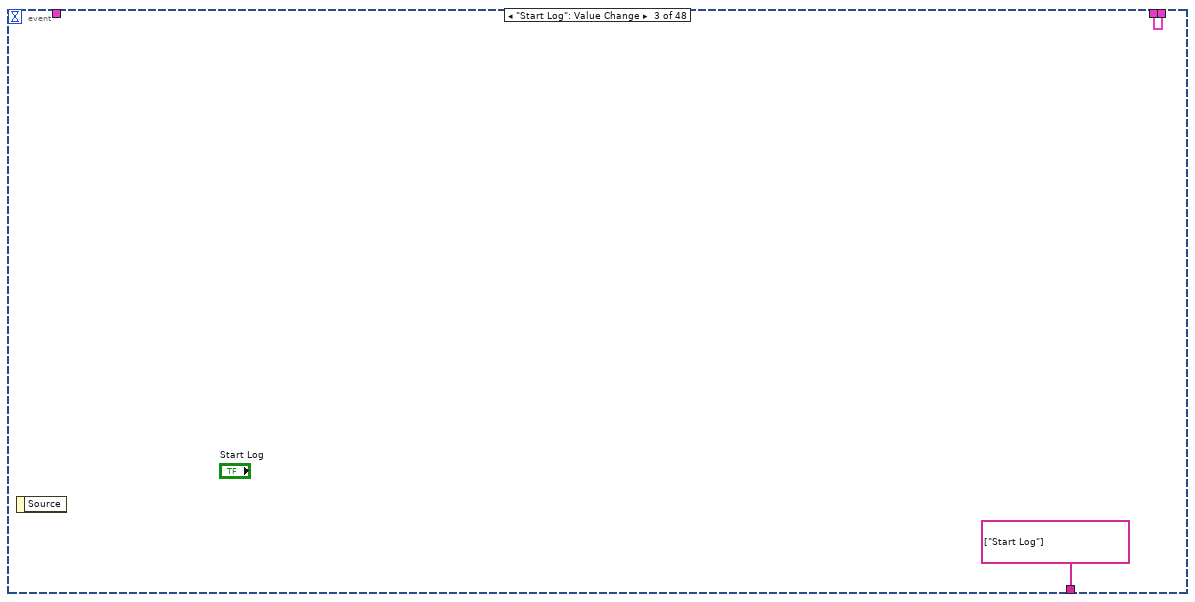
[diagram p7: hidden frame]
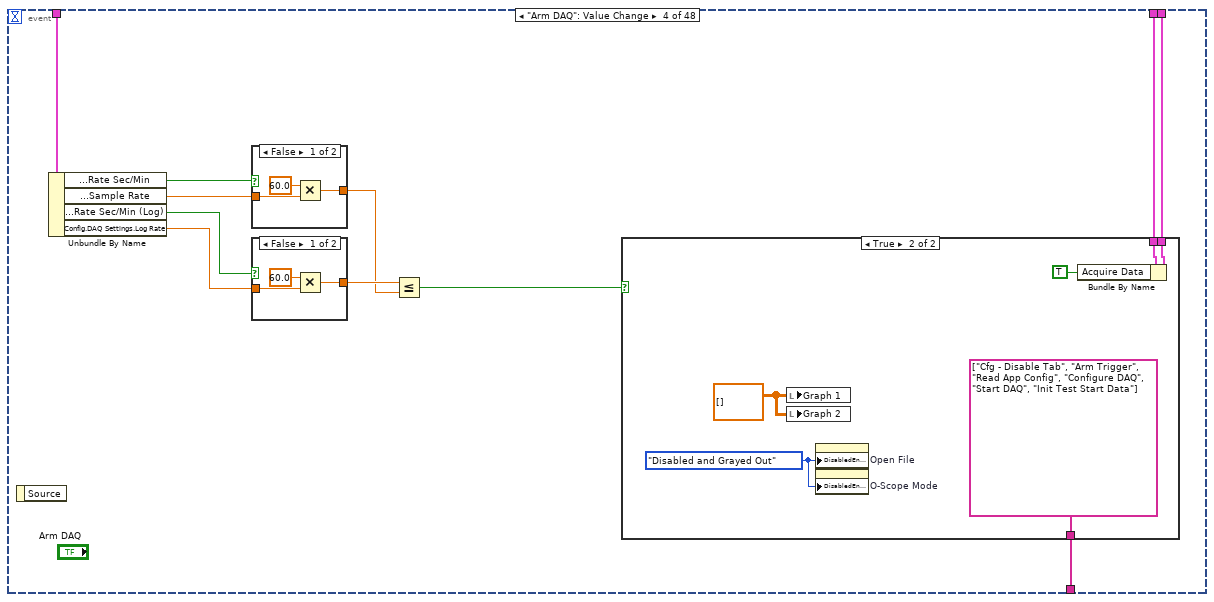
[diagram p8: hidden frame]
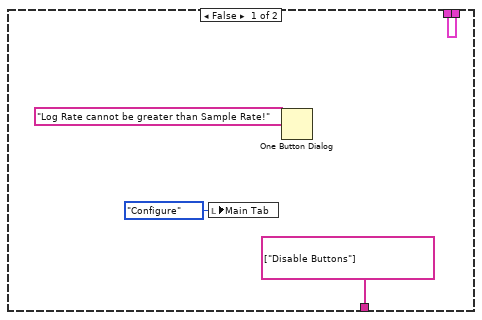
[diagram p11: hidden frame]
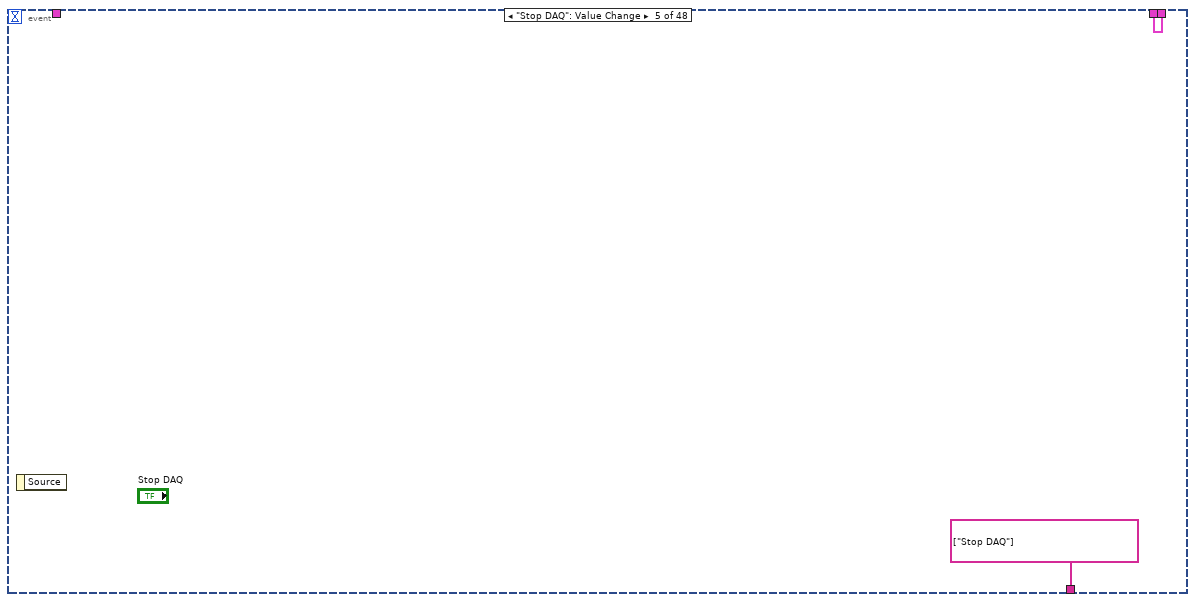
[diagram p12: hidden frame]
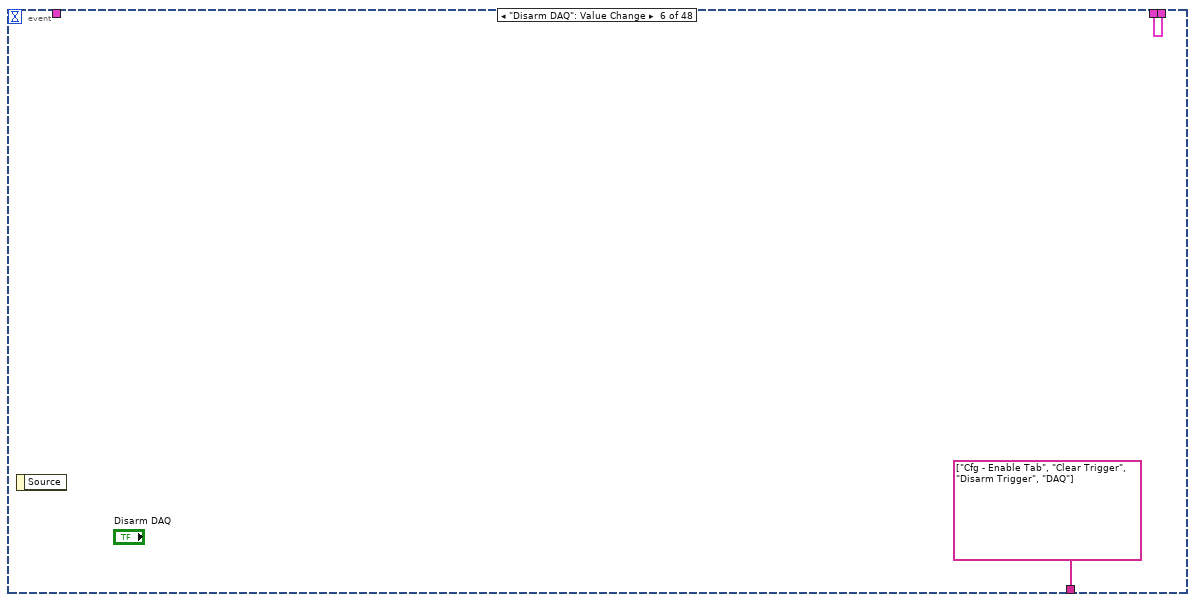
[diagram p13: hidden frame]
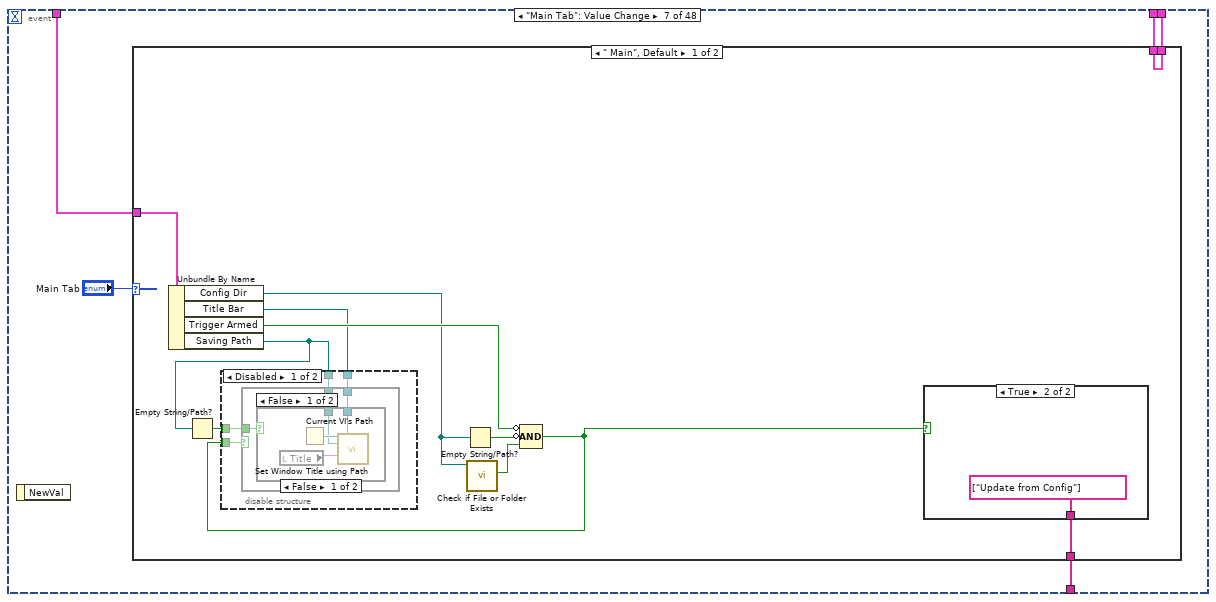
[diagram p14: hidden frame]
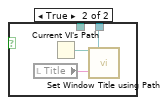
[diagram p15: hidden frame]
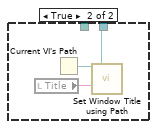
[diagram p16: hidden frame]
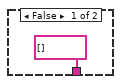
[diagram p18: hidden frame]
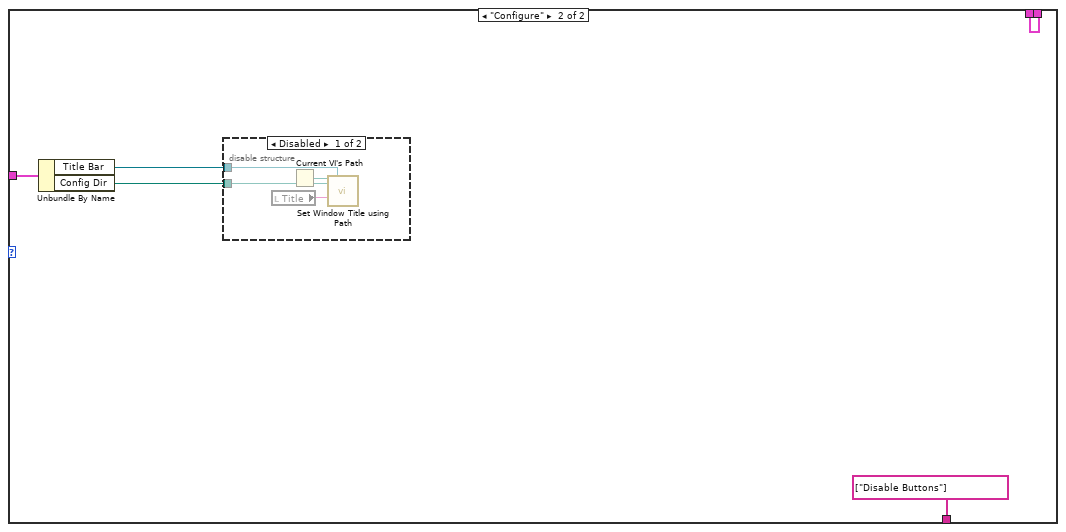
[diagram p19: hidden frame]
diagram:
  w1 = refnum<file> refnum  # Log Path Ref
  (unwired) string[] ["9205/0_AI-00", "9205/0_AI-01", "9205/0_AI-02", "9205/0_AI-03", "9205/0_AI-04", "9205/0_AI-05", "9205/0_AI-06", "9205/0_AI-07", "9205/0_AI-08", "9205/0_AI-09", "9205/0_AI-10", "9205/0_AI-11", "9205/0_AI-12", "9205/0_AI-13", "9205/0_AI-14", "9205/0_AI-15", "9205/0_AI-16", "9205/0_AI-17", "9205/0_AI-18", "9205/0_AI-19", "9205/0_AI-20", "9205/0_AI-21", "9205/0_AI-22", "9205/0_AI-23", "9205/0_AI-24", "9205/0_AI-25", "9205/0_AI-26", "9205/0_AI-27", "9205/0_AI-28", "9205/0_AI-29", "9205/0_AI-30", "9205/0_AI-31", "9205/1_AI-00", "9205/1_AI-01", "9205/1_AI-02", "9205/1_AI-03", "9205/1_AI-04", "9205/1_AI-05", "9205/1_AI-06", "9205/1_AI-07", "9205/1_AI-08", "9205/1_AI-09", "9205/1_AI-10", "9205/1_AI-11", "9205/1_AI-12", "9205/1_AI-13", "9205/1_AI-14", "9205/1_AI-15", "9205/1_AI-16", "9205/1_AI-17", "9205/1_AI-18", "9205/1_AI-19", "9205/1_AI-20", "9205/1_AI-21", "9205/1_AI-22", "9205/1_AI-23", "9205/1_AI-24", "9205/1_AI-25", "9205/1_AI-26", "9205/1_AI-27", "9205/1_AI-28", "9205/1_AI-29", "9205/1_AI-30", "9205/1_AI-31", "9205/2_AI-00", "9205/2_AI-01", "9205/2_AI-02", "9205/2_AI-03", "9205/2_AI-04", "9205/2_AI-05", "9205/2_AI-06", "9205/2_AI-07", "9205/2_AI-08", "9205/2_AI-09", "9205/2_AI-10", "9205/2_AI-11", "9205/2_AI-12", "9205/2_AI-13", "9205/2_AI-14", "9205/2_AI-15", "9205/2_AI-16", "9205/2_AI-17", "9205/2_AI-18", "9205/2_AI-19", "9205/2_AI-20", "9205/2_AI-21", "9205/2_AI-22", "9205/2_AI-23", "9205/2_AI-24", "9205/2_AI-25", "9205/2_AI-26", "9205/2_AI-27", "9205/2_AI-28", "9205/2_AI-29", "9205/2_AI-30", "9205/2_AI-31", "9220_AI-00", "9220_AI-01", "9220_AI-02", "9220_AI-03", "9220_AI-04", "9220_AI-05", "9220_AI-06", "9220_AI-07", "9220_AI-08", "9220_AI-09", "9220_AI-10", "9220_AI-11", "9220_AI-12", "9220_AI-13", "9220_AI-14", "9220_AI-15", "9208_AI-00", "9208_AI-01", "9208_AI-02", "9208_AI-03", "9208_AI-04", "9208_AI-05", "9208_AI-06", "9208_AI-07", "9211_TC-00", "9211_TC-01", "9211_TC-02", "9211_TC-03"] ("appended array")
  w2 = FALSE  # Manual Data Mode
  w3 = FALSE  # Add Data Point
  w4 = ""  # Sys Cfg File Name
  w5 = ""  # Sensor File Name
  w6 = ""  # Config Name
  w7 = T13 {"Support Dir (Local)"=path "", "Support Dir (Remote)"=path "", "Config Sub Dir"="", "Last Config (Std)"="", "Last Config (Def)"="", "Last Config (8TC)"=""}  # App Config
  w8 = ""  # Config Extension
  w9 = T14 {"System"="", "Description"=""}  # Selected System
  w10 = tag ""  # System Ref
  w11 = i32[] []  # Data Log Indicies
  w12 = u32 0  # Samples Acquired
  w13 = System_Type."Standard"  # System Type
  w14 = u32 0  # Samples Recorded
  w15 = FALSE  # Load Prompt
  w19 = T16 {"DAQ Settings"={"Trigger Type"=enum."Manual", "Trigger Samples"=0, "Pretrigger Samples"=0, "Trigger Interval"=0.0, "Time Units"=FALSE, "Auto Save"=FALSE, "Sample Rate"=0.0, "Select Analog"=FALSE, "Trigger Value"=0.0, "Trigger Stop Method"=enum."Use Samples Value to Stop Trigger", "Rate Sec/Min"=FALSE, "Save Mode"=enum."Single File", "File Size Limit"=0.0, "Log File Type"=enum."Basic", "Trigger Data Index"=0, "Log Rate"=7.0, "Rate Sec/Min (Log)"=FALSE, "Sample Rate (S/s)"=0.0, "Log Rate (S/s)"=0.0}, "Channels"=[], "Header"={"CA Number"="", "Test Name"="", "Serial Number"="", "Technician"=""}, "Graph Settings"={"Graph Labels"=[], [], [], [], [], [], [], [], [], [], [], [], [], "Graph Toggles"=[], "Axis Toggles"=[], "Graph Range"=enum."1"}, "Test Limits"=[], "All Type Info"=[], "Save Mode"=enum."Single File", "Data Base Path"=path ""}  # Config Saved
  w16 = FALSE  # DAQ Running
  w17 = FALSE  # Revert
  w18 = FALSE  # Changes?
  w20 = T26[] []  # Sensors
  w22 = 0  # Channel Select
  w21 = T11 [{"Channel"="", "Description"="", "Acquire"=FALSE, "Sensor"="", "Chg Sensor"=FALSE, "Cal Date"="", "Offset"=0.0, "Span"=0.0, "Cal"=FALSE, "Test Limits"=FALSE, "Type"="", "Data Index"=0}, {"Channel"="", "Description"="", "Acquire"=FALSE, "Sensor"="", "Chg Sensor"=FALSE, "Cal Date"="", "Offset"=0.0, "Span"=0.0, "Cal"=FALSE, "Test Limits"=FALSE, "Type"="", "Data Index"=0}, {"Channel"="", "Description"="", "Acquire"=FALSE, "Sensor"="", "Chg Sensor"=FALSE, "Cal Date"="", "Offset"=0.0, "Span"=0.0, "Cal"=FALSE, "Test Limits"=FALSE, "Type"="", "Data Index"=0}, {"Channel"="", "Description"="", "Acquire"=FALSE, "Sensor"="", "Chg Sensor"=FALSE, "Cal Date"="", "Offset"=0.0, "Span"=0.0, "Cal"=FALSE, "Test Limits"=FALSE, "Type"="", "Data Index"=0}, {"Channel"="", "Description"="", "Acquire"=FALSE, "Sensor"="", "Chg Sensor"=FALSE, "Cal Date"="", "Offset"=0.0, "Span"=0.0, "Cal"=FALSE, "Test Limits"=FALSE, "Type"="", "Data Index"=0}, {"Channel"="", "Description"="", "Acquire"=FALSE, "Sensor"="", "Chg Sensor"=FALSE, "Cal Date"="", "Offset"=0.0, "Span"=0.0, "Cal"=FALSE, "Test Limits"=FALSE, "Type"="", "Data Index"=0}, {"Channel"="", "Description"="", "Acquire"=FALSE, "Sensor"="", "Chg Sensor"=FALSE, "Cal Date"="", "Offset"=0.0, "Span"=0.0, "Cal"=FALSE, "Test Limits"=FALSE, "Type"="", "Data Index"=0}, {"Channel"="", "Description"="", "Acquire"=FALSE, "Sensor"="", "Chg Sensor"=FALSE, "Cal Date"="", "Offset"=0.0, "Span"=0.0, "Cal"=FALSE, "Test Limits"=FALSE, "Type"="", "Data Index"=0}, {"Channel"="", "Description"="", "Acquire"=FALSE, "Sensor"="", "Chg Sensor"=FALSE, "Cal Date"="", "Offset"=0.0, "Span"=0.0, "Cal"=FALSE, "Test Limits"=FALSE, "Type"="", "Data Index"=0}, {"Channel"="", "Description"="", "Acquire"=FALSE, "Sensor"="", "Chg Sensor"=FALSE, "Cal Date"="", "Offset"=0.0, "Span"=0.0, "Cal"=FALSE, "Test Limits"=FALSE, "Type"="", "Data Index"=0}, {"Channel"="", "Description"="", "Acquire"=FALSE, "Sensor"="", "Chg Sensor"=FALSE, "Cal Date"="", "Offset"=0.0, "Span"=0.0, "Cal"=FALSE, "Test Limits"=FALSE, "Type"="", "Data Index"=0}, {"Channel"="", "Description"="", "Acquire"=FALSE, "Sensor"="", "Chg Sensor"=FALSE, "Cal Date"="", "Offset"=0.0, "Span"=0.0, "Cal"=FALSE, "Test Limits"=FALSE, "Type"="", "Data Index"=0}, {"Channel"="", "Description"="", "Acquire"=FALSE, "Sensor"="", "Chg Sensor"=FALSE, "Cal Date"="", "Offset"=0.0, "Span"=0.0, "Cal"=FALSE, "Test Limits"=FALSE, "Type"="", "Data Index"=0}, {"Channel"="", "Description"="", "Acquire"=FALSE, "Sensor"="", "Chg Sensor"=FALSE, "Cal Date"="", "Offset"=0.0, "Span"=0.0, "Cal"=FALSE, "Test Limits"=FALSE, "Type"="", "Data Index"=0}, {"Channel"="", "Description"="", "Acquire"=FALSE, "Sensor"="", "Chg Sensor"=FALSE, "Cal Date"="", "Offset"=0.0, "Span"=0.0, "Cal"=FALSE, "Test Limits"=FALSE, "Type"="", "Data Index"=0}, {"Channel"="", "Description"="", "Acquire"=FALSE, "Sensor"="", "Chg Sensor"=FALSE, "Cal Date"="", "Offset"=0.0, "Span"=0.0, "Cal"=FALSE, "Test Limits"=FALSE, "Type"="", "Data Index"=0}, {"Channel"="", "Description"="", "Acquire"=FALSE, "Sensor"="", "Chg Sensor"=FALSE, "Cal Date"="", "Offset"=0.0, "Span"=0.0, "Cal"=FALSE, "Test Limits"=FALSE, "Type"="", "Data Index"=0}, {"Channel"="", "Description"="", "Acquire"=FALSE, "Sensor"="", "Chg Sensor"=FALSE, "Cal Date"="", "Offset"=0.0, "Span"=0.0, "Cal"=FALSE, "Test Limits"=FALSE, "Type"="", "Data Index"=0}, {"Channel"="", "Description"="", "Acquire"=FALSE, "Sensor"="", "Chg Sensor"=FALSE, "Cal Date"="", "Offset"=0.0, "Span"=0.0, "Cal"=FALSE, "Test Limits"=FALSE, "Type"="", "Data Index"=0}, {"Channel"="", "Description"="", "Acquire"=FALSE, "Sensor"="", "Chg Sensor"=FALSE, "Cal Date"="", "Offset"=0.0, "Span"=0.0, "Cal"=FALSE, "Test Limits"=FALSE, "Type"="", "Data Index"=0}, {"Channel"="", "Description"="", "Acquire"=FALSE, "Sensor"="", "Chg Sensor"=FALSE, "Cal Date"="", "Offset"=0.0, "Span"=0.0, "Cal"=FALSE, "Test Limits"=FALSE, "Type"="", "Data Index"=0}, {"Channel"="", "Description"="", "Acquire"=FALSE, "Sensor"="", "Chg Sensor"=FALSE, "Cal Date"="", "Offset"=0.0, "Span"=0.0, "Cal"=FALSE, "Test Limits"=FALSE, "Type"="", "Data Index"=0}, {"Channel"="", "Description"="", "Acquire"=FALSE, "Sensor"="", "Chg Sensor"=FALSE, "Cal Date"="", "Offset"=0.0, "Span"=0.0, "Cal"=FALSE, "Test Limits"=FALSE, "Type"="", "Data Index"=0}, {"Channel"="", "Description"="", "Acquire"=FALSE, "Sensor"="", "Chg Sensor"=FALSE, "Cal Date"="", "Offset"=0.0, "Span"=0.0, "Cal"=FALSE, "Test Limits"=FALSE, "Type"="", "Data Index"=0}, {"Channel"="", "Description"="", "Acquire"=FALSE, "Sensor"="", "Chg Sensor"=FALSE, "Cal Date"="", "Offset"=0.0, "Span"=0.0, "Cal"=FALSE, "Test Limits"=FALSE, "Type"="", "Data Index"=0}, {"Channel"="", "Description"="", "Acquire"=FALSE, "Sensor"="", "Chg Sensor"=FALSE, "Cal Date"="", "Offset"=0.0, "Span"=0.0, "Cal"=FALSE, "Test Limits"=FALSE, "Type"="", "Data Index"=0}, {"Channel"="", "Description"="", "Acquire"=FALSE, "Sensor"="", "Chg Sensor"=FALSE, "Cal Date"="", "Offset"=0.0, "Span"=0.0, "Cal"=FALSE, "Test Limits"=FALSE, "Type"="", "Data Index"=0}, {"Channel"="", "Description"="", "Acquire"=FALSE, "Sensor"="", "Chg Sensor"=FALSE, "Cal Date"="", "Offset"=0.0, "Span"=0.0, "Cal"=FALSE, "Test Limits"=FALSE, "Type"="", "Data Index"=0}, {"Channel"="", "Description"="", "Acquire"=FALSE, "Sensor"="", "Chg Sensor"=FALSE, "Cal Date"="", "Offset"=0.0, "Span"=0.0, "Cal"=FALSE, "Test Limits"=FALSE, "Type"="", "Data Index"=0}, {"Channel"="", "Description"="", "Acquire"=FALSE, "Sensor"="", "Chg Sensor"=FALSE, "Cal Date"="", "Offset"=0.0, "Span"=0.0, "Cal"=FALSE, "Test Limits"=FALSE, "Type"="", "Data Index"=0}, {"Channel"="", "Description"="", "Acquire"=FALSE, "Sensor"="", "Chg Sensor"=FALSE, "Cal Date"="", "Offset"=0.0, "Span"=0.0, "Cal"=FALSE, "Test Limits"=FALSE, "Type"="", "Data Index"=0}, {"Channel"="", "Description"="", "Acquire"=FALSE, "Sensor"="", "Chg Sensor"=FALSE, "Cal Date"="", "Offset"=0.0, "Span"=0.0, "Cal"=FALSE, "Test Limits"=FALSE, "Type"="", "Data Index"=0}, {"Channel"="", "Description"="", "Acquire"=FALSE, "Sensor"="", "Chg Sensor"=FALSE, "Cal Date"="", "Offset"=0.0, "Span"=0.0, "Cal"=FALSE, "Test Limits"=FALSE, "Type"="", "Data Index"=0}, {"Channel"="", "Description"="", "Acquire"=FALSE, "Sensor"="", "Chg Sensor"=FALSE, "Cal Date"="", "Offset"=0.0, "Span"=0.0, "Cal"=FALSE, "Test Limits"=FALSE, "Type"="", "Data Index"=0}, {"Channel"="", "Description"="", "Acquire"=FALSE, "Sensor"="", "Chg Sensor"=FALSE, "Cal Date"="", "Offset"=0.0, "Span"=0.0, "Cal"=FALSE, "Test Limits"=FALSE, "Type"="", "Data Index"=0}, {"Channel"="", "Description"="", "Acquire"=FALSE, "Sensor"="", "Chg Sensor"=FALSE, "Cal Date"="", "Offset"=0.0, "Span"=0.0, "Cal"=FALSE, "Test Limits"=FALSE, "Type"="", "Data Index"=0}, {"Channel"="", "Description"="", "Acquire"=FALSE, "Sensor"="", "Chg Sensor"=FALSE, "Cal Date"="", "Offset"=0.0, "Span"=0.0, "Cal"=FALSE, "Test Limits"=FALSE, "Type"="", "Data Index"=0}, {"Channel"="", "Description"="", "Acquire"=FALSE, "Sensor"="", "Chg Sensor"=FALSE, "Cal Date"="", "Offset"=0.0, "Span"=0.0, "Cal"=FALSE, "Test Limits"=FALSE, "Type"="", "Data Index"=0}, {"Channel"="", "Description"="", "Acquire"=FALSE, "Sensor"="", "Chg Sensor"=FALSE, "Cal Date"="", "Offset"=0.0, "Span"=0.0, "Cal"=FALSE, "Test Limits"=FALSE, "Type"="", "Data Index"=0}, {"Channel"="", "Description"="", "Acquire"=FALSE, "Sensor"="", "Chg Sensor"=FALSE, "Cal Date"="", "Offset"=0.0, "Span"=0.0, "Cal"=FALSE, "Test Limits"=FALSE, "Type"="", "Data Index"=0}, {"Channel"="", "Description"="", "Acquire"=FALSE, "Sensor"="", "Chg Sensor"=FALSE, "Cal Date"="", "Offset"=0.0, "Span"=0.0, "Cal"=FALSE, "Test Limits"=FALSE, "Type"="", "Data Index"=0}, {"Channel"="", "Description"="", "Acquire"=FALSE, "Sensor"="", "Chg Sensor"=FALSE, "Cal Date"="", "Offset"=0.0, "Span"=0.0, "Cal"=FALSE, "Test Limits"=FALSE, "Type"="", "Data Index"=0}, {"Channel"="", "Description"="", "Acquire"=FALSE, "Sensor"="", "Chg Sensor"=FALSE, "Cal Date"="", "Offset"=0.0, "Span"=0.0, "Cal"=FALSE, "Test Limits"=FALSE, "Type"="", "Data Index"=0}, {"Channel"="", "Description"="", "Acquire"=FALSE, "Sensor"="", "Chg Sensor"=FALSE, "Cal Date"="", "Offset"=0.0, "Span"=0.0, "Cal"=FALSE, "Test Limits"=FALSE, "Type"="", "Data Index"=0}, {"Channel"="", "Description"="", "Acquire"=FALSE, "Sensor"="", "Chg Sensor"=FALSE, "Cal Date"="", "Offset"=0.0, "Span"=0.0, "Cal"=FALSE, "Test Limits"=FALSE, "Type"="", "Data Index"=0}, {"Channel"="", "Description"="", "Acquire"=FALSE, "Sensor"="", "Chg Sensor"=FALSE, "Cal Date"="", "Offset"=0.0, "Span"=0.0, "Cal"=FALSE, "Test Limits"=FALSE, "Type"="", "Data Index"=0}, {"Channel"="", "Description"="", "Acquire"=FALSE, "Sensor"="", "Chg Sensor"=FALSE, "Cal Date"="", "Offset"=0.0, "Span"=0.0, "Cal"=FALSE, "Test Limits"=FALSE, "Type"="", "Data Index"=0}, {"Channel"="", "Description"="", "Acquire"=FALSE, "Sensor"="", "Chg Sensor"=FALSE, "Cal Date"="", "Offset"=0.0, "Span"=0.0, "Cal"=FALSE, "Test Limits"=FALSE, "Type"="", "Data Index"=0}, {"Channel"="", "Description"="", "Acquire"=FALSE, "Sensor"="", "Chg Sensor"=FALSE, "Cal Date"="", "Offset"=0.0, "Span"=0.0, "Cal"=FALSE, "Test Limits"=FALSE, "Type"="", "Data Index"=0}, {"Channel"="", "Description"="", "Acquire"=FALSE, "Sensor"="", "Chg Sensor"=FALSE, "Cal Date"="", "Offset"=0.0, "Span"=0.0, "Cal"=FALSE, "Test Limits"=FALSE, "Type"="", "Data Index"=0}, {"Channel"="", "Description"="", "Acquire"=FALSE, "Sensor"="", "Chg Sensor"=FALSE, "Cal Date"="", "Offset"=0.0, "Span"=0.0, "Cal"=FALSE, "Test Limits"=FALSE, "Type"="", "Data Index"=0}, {"Channel"="", "Description"="", "Acquire"=FALSE, "Sensor"="", "Chg Sensor"=FALSE, "Cal Date"="", "Offset"=0.0, "Span"=0.0, "Cal"=FALSE, "Test Limits"=FALSE, "Type"="", "Data Index"=0}, {"Channel"="", "Description"="", "Acquire"=FALSE, "Sensor"="", "Chg Sensor"=FALSE, "Cal Date"="", "Offset"=0.0, "Span"=0.0, "Cal"=FALSE, "Test Limits"=FALSE, "Type"="", "Data Index"=0}, {"Channel"="", "Description"="", "Acquire"=FALSE, "Sensor"="", "Chg Sensor"=FALSE, "Cal Date"="", "Offset"=0.0, "Span"=0.0, "Cal"=FALSE, "Test Limits"=FALSE, "Type"="", "Data Index"=0}, {"Channel"="", "Description"="", "Acquire"=FALSE, "Sensor"="", "Chg Sensor"=FALSE, "Cal Date"="", "Offset"=0.0, "Span"=0.0, "Cal"=FALSE, "Test Limits"=FALSE, "Type"="", "Data Index"=0}, {"Channel"="", "Description"="", "Acquire"=FALSE, "Sensor"="", "Chg Sensor"=FALSE, "Cal Date"="", "Offset"=0.0, "Span"=0.0, "Cal"=FALSE, "Test Limits"=FALSE, "Type"="", "Data Index"=0}, {"Channel"="", "Description"="", "Acquire"=FALSE, "Sensor"="", "Chg Sensor"=FALSE, "Cal Date"="", "Offset"=0.0, "Span"=0.0, "Cal"=FALSE, "Test Limits"=FALSE, "Type"="", "Data Index"=0}, {"Channel"="", "Description"="", "Acquire"=FALSE, "Sensor"="", "Chg Sensor"=FALSE, "Cal Date"="", "Offset"=0.0, "Span"=0.0, "Cal"=FALSE, "Test Limits"=FALSE, "Type"="", "Data Index"=0}, {"Channel"="", "Description"="", "Acquire"=FALSE, "Sensor"="", "Chg Sensor"=FALSE, "Cal Date"="", "Offset"=0.0, "Span"=0.0, "Cal"=FALSE, "Test Limits"=FALSE, "Type"="", "Data Index"=0}, {"Channel"="", "Description"="", "Acquire"=FALSE, "Sensor"="", "Chg Sensor"=FALSE, "Cal Date"="", "Offset"=0.0, "Span"=0.0, "Cal"=FALSE, "Test Limits"=FALSE, "Type"="", "Data Index"=0}, {"Channel"="", "Description"="", "Acquire"=FALSE, "Sensor"="", "Chg Sensor"=FALSE, "Cal Date"="", "Offset"=0.0, "Span"=0.0, "Cal"=FALSE, "Test Limits"=FALSE, "Type"="", "Data Index"=0}, {"Channel"="", "Description"="", "Acquire"=FALSE, "Sensor"="", "Chg Sensor"=FALSE, "Cal Date"="", "Offset"=0.0, "Span"=0.0, "Cal"=FALSE, "Test Limits"=FALSE, "Type"="", "Data Index"=0}, {"Channel"="", "Description"="", "Acquire"=FALSE, "Sensor"="", "Chg Sensor"=FALSE, "Cal Date"="", "Offset"=0.0, "Span"=0.0, "Cal"=FALSE, "Test Limits"=FALSE, "Type"="", "Data Index"=0}, {"Channel"="", "Description"="", "Acquire"=FALSE, "Sensor"="", "Chg Sensor"=FALSE, "Cal Date"="", "Offset"=0.0, "Span"=0.0, "Cal"=FALSE, "Test Limits"=FALSE, "Type"="", "Data Index"=0}, {"Channel"="", "Description"="", "Acquire"=FALSE, "Sensor"="", "Chg Sensor"=FALSE, "Cal Date"="", "Offset"=0.0, "Span"=0.0, "Cal"=FALSE, "Test Limits"=FALSE, "Type"="", "Data Index"=0}]  # Channel Display
  w23 = FALSE  # Acquire Data
  w24 = ""  # Last SN
  w25 = u32 0  # Connected Timer
  w27 = path ""  # App Config Path
  w28 = u32 0  # timer
  w30 = refnum<k21> refnum  # DI Task
  w31 = refnum<k21> refnum  # DO Task
  w32 = i16 0  # Total Channel Count
  w33 = FALSE  # Segment File
  w34 = FALSE  # Midnight Rollover
  w35 = 0  # Pretrigger Size
  w36 = 0.0  # Time Offset
  w37 = timestamp(0 s since 1904-01-01)  # Start Timestamp
  w38 = timestamp(0 s since 1904-01-01)  # Midnight Check
  w39 = FALSE  # Data View Mode
  w40 = FALSE  # O-Scope Mode
  w41 = FALSE  # UnPause Once
  w42 = u32 0  # Buffer Size
  w43 = path ""  # Data File Path
  w44 = FALSE  # Force Update
  w45 = FALSE  # Pause Graph
  w46 = refnum<vi>[] []  # Graph Ch Refs
  w47 = refnum<k21> refnum  # AI Task
  w48 = path ""  # Calibration Path
  w49 = sgl[][] []  # Data
  w50 = 0.0  # New Time
  w51 = 0.0  # Previous Time
  w52 = path ""  # Saving Path
  w53 = FALSE  # File Created?
  w54 = T27 []  # Scaling
  w55 = FALSE  # Virtual Trigger
  w56 = 0.0  # Interval
  w57 = FALSE  # Trigger Armed
  w58 = FALSE  # Acquiring Data
  w59 = 0  # Trigger Index
  w60 = bool[] []  # Channel Filter
  w61 = string[] []  # Channel Addresses
  w62 = errorcluster {"status"=FALSE, "code"=0, "source"=""}  # Error
  w63 = T16 {"DAQ Settings"={"Trigger Type"=enum."Manual", "Trigger Samples"=0, "Pretrigger Samples"=0, "Trigger Interval"=0.0, "Time Units"=FALSE, "Auto Save"=FALSE, "Sample Rate"=0.0, "Select Analog"=FALSE, "Trigger Value"=0.0, "Trigger Stop Method"=enum."Use Samples Value to Stop Trigger", "Rate Sec/Min"=FALSE, "Save Mode"=enum."Single File", "File Size Limit"=0.0, "Log File Type"=enum."Basic", "Trigger Data Index"=0, "Log Rate"=7.0, "Rate Sec/Min (Log)"=FALSE, "Sample Rate (S/s)"=0.0, "Log Rate (S/s)"=0.0}, "Channels"=[], "Header"={"CA Number"="", "Test Name"="", "Serial Number"="", "Technician"=""}, "Graph Settings"={"Graph Labels"=[], [], [], [], [], [], [], [], [], [], [], [], [], "Graph Toggles"=[], "Axis Toggles"=[], "Graph Range"=enum."1"}, "Test Limits"=[], "All Type Info"=[], "Save Mode"=enum."Single File", "Data Base Path"=path ""}  # Config
  w64 = path ""  # App Path
  w65 = path ""  # Config Dir
  n1 = control-ref of="Title Bar"() -> (w26:refnum<vi>)
  n2 = Bundle("Virtual Trigger"=w55, "Interval"=w56, "Trigger Armed"=w57, "Acquiring Data"=w58, "Channel Filter"=w60, "Error"=w62, "Data"=w49, "Trigger Index"=w59, "App Path"=w64, "Config Dir"=w65, "Config"=w63, "Channel Addresses"=w61, "Scaling"=w54, "File Created?"=w53, "Saving Path"=w52, "Previous Time"=w51, "New Time"=w50, "Calibration Path"=w48, "AI Task"=w47, "Graph Ch Refs"=w46, "Pause Graph"=w45, "Force Update"=w44, "Data File Path"=w43, "Buffer Size"=w42, "UnPause Once"=w41, "O-Scope Mode"=w40, "Data View Mode"=w39, "Midnight Check"=w38, "Start Timestamp"=w37, "Time Offset"=w36, "Pretrigger Size"=w35, "Midnight Rollover"=w34, "Segment File"=w33, "Total Channel Count"=w32, "DO Task"=w31, "DI Task"=w30, "timer"=w28, "App Config Path"=w27, "Title Bar"=w26, "Connected Timer"=w25, "Last SN"=w24, "Acquire Data"=w23, "Channel Select"=w22, "Channel Display"=w21, "Sensors"=w20, "Config Saved"=w19, "Changes?"=w18, "Revert"=w17, "DAQ Running"=w16, "Load Prompt"=w15, "Samples Recorded"=w14, "System Type"=w13, "Samples Acquired"=w12, "Data Log Indicies"=w11, "System Ref"=w10, "Selected System"=w9, "Config Extension"=w8, "App Config"=w7, "Config Name"=w6, "Sensor File Name"=w5, "Sys Cfg File Name"=w4, "Add Data Point"=w3, "Manual Data Mode"=w2, "Log Path Ref"=w1) -> (w66:T28)  [unwired: 1 in]
  n3 = while {
    shift-left: string[] ["Init", "Init Test Start Data", "Read App Config", "Get Systems Config", "Connection Window", "Cfg - Clear", "Cfg - Init", "Cfg - Enable Tab", "Cfg - Load Sensors", "Cfg - Update Channel Group", "Cfg - Update DAQ Table", "Cfg - Load Last Config"] ("event queue out") -> [w73]
    shift-right: [w67] -> _
    shift-left: w66 -> [w72]
    shift-right: [w71] -> _
    stop <- w75 continue-if-true
    n4 = call "Get Next Event.vi"("Exit Event"="Exit", "event queue in"=w73) -> ("Condition (Exit:F)"=w75:bool, "next event"=w74:string, "event queue out"=w70:string[])  [unwired: 3 in]
    n5 = Wait (ms)(milliseconds to wait=u32 0) -> ()  [unwired: 1 out]
    n6 = case shown="\"Unused Items\"" w74 {
      tunnel: w72 -> [w77 w676 w695 w714 w739 w760 w767 w773 w776 w784 w811 w867 w894 w909 w947 w963 w995 w1062 w1106 w1115 w1150 w1180 w1188 w1221 w1253 w1274 w1360 w1531 w1573 w1583 w1589 w1608 w1631 w1636 w1639 w1644 w1645 w1667 w1742 w1760 w1784 w1802 w1808 w1820 w1845 w1869 w1889 w1909 w1916 w1921 w1929 w1937 w1955 w1966 w1987 w2013 w2032 w2044 w2079 w2103 w2119 w2125]
      tunnel: [w76 w688 w694 w713 w739 w760 w767 w773 w776 w783 w813 w866 w894 w914 w946 w962 w991 w1063 w1105 w1115 w1149 w1180 w1188 w1221 w1252 w1273 w1359 w1530 w1578 w1587 w1589 w1607 w1630 w1637 w1639 w1644 w1645 w1666 w1741 w1759 w1783 w1801 w1807 w1819 w1844 w1868 w1888 w1908 w1915 w1920 w1928 w1937 w1955 w1965 w1986 w2012 w2031 w2044 w2079 w2102 w2119 w2125] -> w71
      tunnel: w70 -> [w81 w678 w698 w706 w740 w761 w768 w772 w775 w795 w802 w871 w893 w912 w943 w964 w988 w1058 w1104 w1119 w1123 w1179 w1187 w1203 w1250 w1271 w1337 w1526 w1579 w1588 w1594 w1604 w1632 w1635 _ w1642 w1647 w1661 w1738 w1758 w1782 w1800 w1806 w1817 w1842 w1867 w1886 w1905 w1912 w1919 w1927 w1935 w1953 w1963 w1984 w2010 w2029 w2042 w2078 w2100 w2118 w2124]
      tunnel: [w82 w678 w698 w707 w741 w762 w764 w772 w775 w795 w806 w870 w893 w911 w944 w964 w989 w1057 w1103 w1118 w1123 w1179 w1187 w1222 w1250 w1271 w1328 w1527 w1579 w1588 w1594 w1605 w1632 w1635 string[] [] ("event queue out") w1640 w1647 w1661 w1737 w1758 w1781 w1800 w1806 w1818 w1843 w1867 w1887 w1906 w1913 w1919 w1927 w1936 w1954 w1964 w1985 w2011 w2030 w2043 w2078 w2101 w2118 w2124] -> w67
      frame "Main", Default {
        n7 = event shown="[25] \"Delete Sensor\": Value Change" {
          selector: _ -> [_ _ _ _ _ _ _ _ _ _ _ _ _ _ _ _ _ _ _ _ _ _ _ _ _ _ _ _ _ _ _ _ _ _ _ _ _ _ _ _ _ _ _ _ _ _ _ _]
          dyn-events: _ -> [_ _ _ _ _ _ _ _ _ _ _ _ _ _ _ _ _ _ _ _ _ _ _ _ _ _ _ _ _ _ _ _ _ _ _ _ _ _ _ _ _ _ _ _ _ _ _ _]
          timeout: 100 -> [_ _ _ _ _ _ _ _ _ _ _ _ _ _ _ _ _ _ _ _ _ _ _ _ _ _ _ _ _ _ _ _ _ _ _ _ _ _ _ _ _ _ _ _ _ _ _ _]
          tunnel: [w86 w100 string[] ["Start Log"] w123 string[] ["Stop DAQ"] string[] ["Cfg - Enable Tab", "Clear Trigger", "Disarm Trigger", "DAQ"] w146 w190 w198 w211 w218 string[] ["Update Graph"] ("f") string[] [] ("f") string[] [] ("f") w294 string[] ["Exit Mode"] ("f") w300 string[] [] ("f") w348 w370 w383 string[] ["Cfg - Load"] string[] ["Cfg - Store Channel Group", "Cfg - Save"] w404 string[] ["Cfg - Add Sensor"] string[] ["Cfg - Delete Sensor"] string[] ["Cfg - Save", "Cfg - Store Channel Group", "Cfg - Check for Sensor Select", "Cfg - Check for Calibrate"] string[] [] string[] ["Cfg - Save"] string[] [] string[] ["Cfg - Update DAQ Table", "Cfg - Save"] string[] ["Cfg - Update DAQ Table"] w543 string[] ["Cfg - Save", "Cfg - Update Fields"] string[] ["Cfg - Save", "Cfg - Update Fields"] string[] ["Cfg - Save"] string[] ["Cfg - Save"] string[] ["Cfg - Save"] string[] ["Cfg - Save"] string[] ["Cfg - Save"] string[] ["Cfg - Save"] string[] ["Cfg - Save"] string[] [] string[] ["Cfg - Save", "Cfg - Load Last Config"] w634 string[] ["Synch Files with Server"] string[] [] w661] -> w80
          tunnel: w77 -> [w97 w106 _ w120 _ _ w149 w194 w201 w213 w221 w254 _ _ w293 _ w307 w343 w349 w371 w382 _ _ w399 _ _ _ _ _ _ _ _ w547 _ _ _ _ _ _ _ _ _ _ _ _ _ w644 w657]
          tunnel: w77 -> [w84 w107 w111 w122 w143 w145 w148 w195 w207 w215 w230 w258 w272 w277 w287 w298 w309 w344 w353 w373 w378 w393 w394 w402 w411 w413 w417 w420 w472 w487 w506 w540 w545 w564 w569 w574 w579 w585 w591 w597 w603 w610 w615 w624 w633 w637 w646 w660]
          tunnel: [w84 w107 w111 w121 w143 w145 w147 w195 w207 w215 w230 w257 w271 w276 w286 w298 w308 w344 w353 w373 w377 w392 w394 w401 w411 w413 w416 w420 w471 w487 w505 w539 w546 w563 w568 w573 w578 w584 w590 w596 w602 w609 w614 w622 w633 w637 w646 w659] -> w76
          event Timeout {
            n8 = event-data() -> ()  [unwired: 1 in, 1 out]
            n9 = Unbundle By Name(w97) -> ("Acquiring Data"=w85:bool, "Pause Graph"=w91:bool, "Trigger Armed"=w90:bool, "Acquiring Data"=w88:bool, "O-Scope Mode"=w87:bool)
            "DAQ Armed" <- w90
            "In O-scope Mode" <- w87
            n10 = Get Date/Time String(date format (0)=enum16{"short", "long", "abbreviated"}."short", want seconds? (F)=TRUE) -> (date string=→"Date":string, time string=→"Time":string)  [unwired: 1 in]
            n11 = Or(x=w90, y=w87) -> (x .or. y?=w83:bool)
            n12 = Not(x=w91) -> (.not. x?=w92:bool)
            n13 = Compound Arithmetic op=AND(w88, invert w87) -> (→"Acquiring Data 2":bool)
            n14 = case shown="True" w83 {
              tunnel: [string[] [] string[] ["DAQ"]] -> w86
              frame False {
              }
              frame True {
              }
            }
            n15 = property on="Acquiring Tab" class="TabCtl (strict)"("Visible"=w85) -> ()  [unwired: 2 in, 2 out]
            n16 = local write "Play"(w92) -> ()
            n17 = local write "Pause"(w91) -> ()
          }
          event Panel Close? {
            # "If Config File Exists, Save the Graph Settings First"
            # "Check if Config File has been loaded"
            n18 = event-data() -> ()  [unwired: 1 in, 2 out]
            n19 = Unbundle By Name(w106) -> ("Config Dir"=w105:path)
            n20 = Empty String/Path?(string/path=w105) -> (empty?=w104:bool)
            n21 = call <vilib>:"Check if File or Folder Exists.vi"("path"=w105) -> ("file or folder exists?"=w103:bool)  [unwired: 8 in, 2 out]
            n22 = Not(x=w104) -> (.not. x?=w102:bool)
            n23 = And(x=w103, y=w102) -> (x .and. y?=w101:bool)
            n24 = case shown="True" w101 {
              tunnel: [string[] ["Disarm Trigger", "Stop DAQ", "Exit"] ("f") string[] ["Save Graph Settings", "Disarm Trigger", "Stop DAQ", "Exit"] ("f")] -> w100
              frame False {
              }
              frame True {
              }
            }
            n25 = event-data("Discard?"=TRUE) -> ()  [unwired: 1 in, 1 out]
          }
          event "Start Log": Value Change {
            n26 = event-data() -> ()  [unwired: 1 in, 1 out]
          }
          event "Arm DAQ": Value Change {
            n27 = event-data() -> ()  [unwired: 1 in, 1 out]
            n28 = Unbundle By Name(w120) -> ("Config.DAQ Settings.Rate Sec/Min"=w119:bool, "Config.DAQ Settings.Sample Rate"=w118:dbl, "Config.DAQ Settings.Rate Sec/Min (Log)"=w117:bool, "Config.DAQ Settings.Log Rate"=w116:dbl)
            n29 = case shown="False" w119 {
              tunnel: w118 -> [w130 w131]
              tunnel: [w128 w131] -> w114
              frame False {
                n30 = Multiply(x=60.0, y=w130) -> (x*y=w128:dbl)
              }
              frame True {
              }
            }
            n31 = case shown="False" w117 {
              tunnel: w116 -> [w126 w127]
              tunnel: [w124 w127] -> w115
              frame False {
                n32 = Multiply(x=60.0, y=w126) -> (x*y=w124:dbl)
              }
              frame True {
              }
            }
            n33 = Less Or Equal?(x=w115, y=w114) -> (x <= y?=w113:bool)
            n34 = case shown="True" w113 {
              tunnel: [string[] ["Disable Buttons"] string[] ["Cfg - Disable Tab", "Arm Trigger", "Read App Config", "Configure DAQ", "Start DAQ", "Init Test Start Data"]] -> w123
              tunnel: w122 -> [w135 w139]
              tunnel: [w135 w138] -> w121
              frame False {
                n35 = local write "Main Tab"(enum32{" Main", "Configure"}."Configure" ("Main Tab")) -> ()
                n36 = One Button Dialog(message="Log Rate cannot be greater than Sample Rate!") -> ()  [unwired: 1 in, 1 out]
              }
              frame True {
                w141 = T30."Disabled and Grayed Out" ("Disabled")
                w137 = sgl[][] [] ("Graph")
                n37 = local write "Graph 1"(w137) -> ()
                n38 = local write "Graph 2"(w137) -> ()
                n39 = property on="Open File" class="Bool"("DisabledEnum"=w141) -> ()  [unwired: 2 in, 2 out]
                n40 = property on="O-Scope Mode" class="Bool"("DisabledEnum"=w141) -> ()  [unwired: 2 in, 2 out]
                n41 = Bundle By Name(cluster=w139, "Acquire Data"=TRUE) -> (w138:T28)
              }
            }
          }
          event "Stop DAQ": Value Change {
            n42 = event-data() -> ()  [unwired: 1 in, 1 out]
          }
          event "Disarm DAQ": Value Change {
            n43 = event-data() -> ()  [unwired: 1 in, 1 out]
          }
          event "Main Tab": Value Change {
            n44 = event-data() -> ()  [unwired: 1 in, 1 out]
            n45 = case shown="\" Main\", Default" "Main Tab" {
              tunnel: w149 -> [w158 w183]
              tunnel: w148 -> [w152 w185]
              tunnel: [w152 w185] -> w147
              tunnel: [w161 string[] ["Disable Buttons"] ("f")] -> w146
              frame " Main", Default {
                n46 = Unbundle By Name(w158) -> ("Config Dir"=w151:path, "Title Bar"=w153:refnum<vi>, "Trigger Armed"=w156:bool, "Saving Path"=w155:path)
                n47 = Empty String/Path?(string/path=w155) -> (empty?=w154:bool)
                n48 = Empty String/Path?(string/path=w151) -> (empty?=w160:bool)
                n49 = call <vilib>:"Check if File or Folder Exists.vi"("path"=w151) -> ("file or folder exists?"=w159:bool)  [unwired: 8 in, 2 out]
                n50 = Compound Arithmetic op=AND(invert w156, invert w160, w159) -> (w157:bool)
                n51 = disable-structure shown="Disabled" {
                  disable-tunnel: w157 -> [w165 _]
                  disable-tunnel: w155 -> [w164 _]
                  disable-tunnel: w154 -> [w163 _]
                  disable-tunnel: w153 -> [w162 _]
                  frame Disabled {
                    n52 = case shown="False" w165 {
                      tunnel: w164 -> [w168 _]
                      tunnel: w163 -> [w167 _]
                      tunnel: w162 -> [w166 w176]
                      frame False {
                        n53 = case shown="False" w167 {
                          tunnel: w168 -> [w171 _]
                          tunnel: w166 -> [w169 w173]
                          frame False {
                            n54 = local read "Title"() -> (w170:string)
                            n55 = Current VI's Path() -> (path=w172:path)
                            n56 = call "Set Window Title using Path.vi"("VI path"=w172, "Title Bar"=w169, "File Path"=w171, "Title"=w170) -> ()  [unwired: 11 in, 1 out]
                          }
                          frame True {
                            n57 = local read "Title"() -> (w174:string)
                            n58 = Current VI's Path() -> (path=w175:path)
                            n59 = call "Set Window Title using Path.vi"("VI path"=w175, "Title Bar"=w173, "Title"=w174) -> ()  [unwired: 12 in, 1 out]
                          }
                        }
                      }
                      frame True {
                        n60 = local read "Title"() -> (w177:string)
                        n61 = Current VI's Path() -> (path=w178:path)
                        n62 = call "Set Window Title using Path.vi"("VI path"=w178, "Title Bar"=w176, "Title"=w177) -> ()  [unwired: 12 in, 1 out]
                      }
                    }
                  }
                  frame Enabled {
                  }
                }
                n63 = case shown="True" w157 {
                  tunnel: [string[] [] ("f") string[] ["Update from Config"] ("f")] -> w161
                  frame False {
                  }
                  frame True {
                  }
                }
              }
              frame "Configure" {
                n64 = Unbundle By Name(w183) -> ("Title Bar"=w181:refnum<vi>, "Config Dir"=w182:path)
                n65 = disable-structure shown="Disabled" {
                  disable-tunnel: w182 -> [w188 _]
                  disable-tunnel: w181 -> [w186 _]
                  frame Disabled {
                    n66 = local read "Title"() -> (w187:string)
                    n67 = Current VI's Path() -> (path=w189:path)
                    n68 = call "Set Window Title using Path.vi"("VI path"=w189, "Title Bar"=w186, "File Path"=w188, "Title"=w187) -> ()  [unwired: 11 in, 1 out]
                  }
                  frame Enabled {
                  }
                }
              }
            }
          }
          event "Graph Toggles": Value Change {
            n69 = event-data() -> ()  [unwired: 1 in, 1 out]
            n70 = Unbundle By Name(w194) -> ("Data View Mode"=w193:bool)
            n71 = case shown="False" w193 {
              tunnel: [string[] ["Save Graph Settings"] ("f") string[] [] ("f")] -> w191
              frame False {
              }
              frame True {
              }
            }
            n72 = Build Array (concatenate)(string[] ["Update Graph Toggles"] ("f"), w191) -> (w190:string[])
          }
          event "Main Toggle": Value Change {
            n73 = event-data() -> ()  [unwired: 1 in, 1 out]
            n74 = Unbundle By Name(w201) -> ("Data View Mode"=w202:bool)
            n75 = case shown="False" w202 {
              tunnel: [string[] ["Save Graph Settings"] ("f") string[] [] ("f")] -> w199
              frame False {
              }
              frame True {
              }
            }
            n76 = Initialize Array("Main Toggle", 16 ("dimension size")) -> (w203:bool[])
            n77 = Array To Cluster(array=w203) -> (cluster=w206:T33)
            n78 = local write "Graph Toggles"(w206) -> ()
            n79 = Build Array (concatenate)(string[] ["Update Graph Toggles"] ("f"), w199) -> (w198:string[])
          }
          event "Axis Toggles": Value Change {
            n80 = event-data() -> ()  [unwired: 1 in, 1 out]
            n81 = Unbundle By Name(w213) -> ("Data View Mode"=w214:bool)
            n82 = case shown="False" w214 {
              tunnel: [string[] ["Save Graph Settings"] ("f") string[] [] ("f")] -> w210
              frame False {
              }
              frame True {
              }
            }
            n83 = Build Array (concatenate)(string[] ["Update Axis Toggles"] ("f"), w210) -> (w211:string[])
          }
          event "Axis Toggle All": Value Change {
            n84 = event-data() -> ()  [unwired: 1 in, 1 out]
            n85 = Unbundle By Name(w221) -> ("Data View Mode"=w222:bool)
            n86 = case shown="False" w222 {
              tunnel: [string[] ["Save Graph Settings"] ("f") string[] [] ("f")] -> w219
              frame False {
              }
              frame True {
              }
            }
            n87 = Initialize Array("Axis Toggle All", 16 ("dimension size")) -> (w223:bool[])
            n88 = Select(t=u32 16711680, s="Axis Toggle All", f=u32 16777226) -> (s? t:f=w228:u32)
            n89 = Array To Cluster(array=w223) -> (cluster=w229:T33)
            n90 = property on="Axis Toggle All" class="Bool (strict)"("BoolText.TextColor"=w228) -> ()  [unwired: 2 in, 2 out]
            n91 = local write "Axis Toggles"(w229) -> ()
            n92 = Build Array (concatenate)(string[] ["Update Axis Toggles"] ("f"), w219) -> (w218:string[])
          }
          event "Graph 2": Scale Range Change {
            w255 = TRUE ("Pause Graph")
            n93 = event-data() -> ("NewRange.Maximum"=w256:dbl, "NewRange.Minimum"=w252:dbl)  [unwired: 1 in]
            n94 = Unbundle By Name(w254) -> ("Buffer Size"=w253:u32, "Graph Ch Refs"=w251:refnum<vi>[])
            n95 = Round Toward +Infinity(x=w256) -> (ceil(x): smallest int >= x=w234:dbl)
            n96 = property on="Graph 2" class="WFGraph (strict)"() -> ("XScale.Offset"=w249:dbl, "XScale.Multiplier"=w244:dbl)  [unwired: 2 in, 2 out]
            n97 = Round Toward +Infinity(x=w252) -> (ceil(x): smallest int >= x=w233:dbl)
            n98 = Subtract(x=w234, y=w233) -> (x-y=w248:dbl)
            n99 = Subtract(x=w233, y=w249) -> (x-y=w247:dbl)
            n100 = flat-sequence {
              tunnel: w234 -> [w263]
              tunnel: w233 -> [w262]
              tunnel: [w261] -> _
              tunnel: w235 -> [_]
              frame #0 {
                n101 = property on="Graph 1" class="WFGraph (strict)"("XScale.Offset"=w262, "XScale.Maximum"=w263, "XScale.Minimum"=w262) -> (error out=w261:errorcluster)  [unwired: 2 in, 1 out]
              }
            }
            n102 = Divide(x=w248, y=w244) -> (x/y=w246:dbl)
            n103 = Divide(x=w247, y=w244) -> (x/y=w245:dbl)
            n104 = call "Trim Data (by ref).vi"("length"=w253) -> ("Data Out"=w250:sgl[][])  [unwired: 12 in, 2 out]
            n105 = flat-sequence {
              tunnel: w236 -> [w260]
              tunnel: [w260] -> w235
              frame #0 {
                n106 = local write "Graph 1"(w260) -> ()
              }
            }
            n107 = Delete From Array(array=w250, length=w246, index (row)=w245) -> (deleted portion=w237:sgl[][])  [unwired: 1 in, 1 out]
            n108 = Array Size(array=w237) -> (size(s)=w241:i32[])
            n109 = Index Array(array=w241) -> (element=w239:i32)  [unwired: 1 in]
            n110 = Initialize Array(0.0 ("element"), w239) -> (w243:dbl[])
            n111 = Insert Into Array(array=w237, index (col)=0 ("index (row)"), new element=w243) -> (w238:sgl[][])  [unwired: 1 in]
            n112 = for {
              tunnel: w251 -> [w269] mode=indexing
              tunnel: w238 -> [w268]
              tunnel: [w265] -> w236 mode=indexing
              n113 = property class="Ring"(reference=w269) -> ("Value"=w266:variant)  [unwired: 1 in, 2 out]
              n114 = Variant To Data(type=u16 0, Variant=w266) -> (data=w264:u16)  [unwired: 1 in, 1 out]
              n115 = Index Array(array=w268, index (col)=w264) -> (element=w265:sgl[])  [unwired: 1 in]
            }
            n116 = Bundle By Name(cluster=w258, "Pause Graph"=w255, "Force Update"=w255) -> (w257:T28)
          }
          event "Pause": Value Change {
            n117 = event-data() -> ()  [unwired: 1 in, 1 out]
            n118 = Bundle By Name(cluster=w272, "Pause Graph"="Pause") -> (w271:T28)
          }
          event "Play": Value Change {
            n119 = event-data() -> ()  [unwired: 1 in, 1 out]
            n120 = Not(x="Play") -> (.not. x?=w274:bool)
            n121 = Bundle By Name(cluster=w277, "Pause Graph"=w274) -> (w276:T28)
          }
          event "Open File": Value Change {
            n122 = event-data() -> ()  [unwired: 1 in, 1 out]
            n123 = Unbundle By Name(w293) -> ("Config.Data Base Path"=w284:path, "Data File Path"=w282:path)
            n124 = Empty String/Path?(string/path=w282) -> (empty?=w281:bool)
            n125 = Not A Number/Path/Refnum?(number/path/refnum=w282) -> (NaN/Path/Refnum?=w280:bool)
            n126 = Or(x=w281, y=w280) -> (x .or. y?=w279:bool)
            n127 = Select(t=w284, s=w279, f=w282) -> (s? t:f=w283:path)
            n128 = call "File Dialog"("start path"=w283) -> ("selected path"=w285:path, "exists"=w292:bool, "cancelled"=w291:bool, "error out"=w290:errorcluster)  [unwired: 11 in]
            n129 = Unbundle By Name(w290) -> ("status"=w289:bool)
            n130 = Compound Arithmetic op=AND(w292, invert w291, invert w289) -> (w288:bool)
            n131 = case shown="True" w288 {
              tunnel: [string[] [] ("f") string[] ["Data View Mode", "Open Data File"] ("f")] -> w294
              frame False {
              }
              frame True {
              }
            }
            n132 = Bundle By Name(cluster=w287, "Data File Path"=w285) -> (w286:T28)
          }
          event "Mode Exit": Value Change {
            n133 = event-data() -> ()  [unwired: 1 in, 1 out]
          }
          event "O-Scope Mode": Value Change {
            n134 = event-data() -> ()  [unwired: 1 in, 1 out]
            n135 = Unbundle By Name(w307) -> ("Config.DAQ Settings.Trigger Type"=w306:T10, "Config.DAQ Settings.Sample Rate (S/s)"=w304:dbl, "Title Bar"=w299:refnum<vi>)
            n136 = Equal?(x=T10."Manual", y=w306) -> (x = y?=w303:bool)
            n137 = Not Equal To 0?(x=w304) -> (x != 0?=w302:bool)
            n138 = And(x=w303, y=w302) -> (x .and. y?=w301:bool)
            n139 = case shown="True" w301 {
              tunnel: w309 -> [w312 w331]
              tunnel: [w312 w330] -> w308
              tunnel: [string[] [] string[] ["Arm Trigger", "Read App Config", "Read Reg DAQ Racks", "Configure DAQ", "Start DAQ"]] -> w300
              tunnel: w299 -> [_ w313]
              frame False {
                n140 = One Button Dialog(message="You must have Manual trigger selected and a non-zero sample rate in order to enter this mode.") -> ()  [unwired: 1 in, 1 out]
              }
              frame True {
                w319 = T30."Enabled" ("Disabled")
                w315 = T30."Disabled and Grayed Out" ("Disabled")
                w327 = TRUE ("Visible")
                w328 = sgl[][] [] ("Graph")
                n141 = property on="Mode Exit" class="Bool"("Visible"=w327) -> ()  [unwired: 2 in, 2 out]
                n142 = property on="Status" class="Str"("Visible"=w327) -> ()  [unwired: 2 in, 2 out]
                n143 = property on="Status" class="Str"("Text.BGColor"=u32 3381759) -> ()  [unwired: 2 in, 2 out]
                n144 = local write "Graph 1"(w328) -> ()
                n145 = local write "Graph 2"(w328) -> ()
                n146 = property on="Play" class="Bool (strict)"("DisabledEnum"=w319) -> ()  [unwired: 2 in, 2 out]
                n147 = property on="Pause" class="Bool (strict)"("DisabledEnum"=w319) -> ()  [unwired: 2 in, 2 out]
                n148 = property on="Graph Channels" class="Clust (strict)"("DisabledEnum"=w319) -> ()  [unwired: 2 in, 2 out]
                n149 = local read "Title"() -> (w314:string)
                n150 = Current VI's Path() -> (path=w324:path)
                n151 = call "Set Window Title using Path.vi"("VI path"=w324, "Title Bar"=w313, "Title"=w314) -> ()  [unwired: 12 in, 1 out]
                n152 = local write "Pause"(FALSE ("Play")) -> ()
                n153 = local write "Play"(TRUE ("Play")) -> ()
                n154 = local write "Status"("IN O-SCOPE MODE..." ("Status")) -> ()
                n155 = property on="Arm DAQ" class="Bool"("DisabledEnum"=w315) -> ()  [unwired: 2 in, 2 out]
                n156 = property on="Open File" class="Bool"("DisabledEnum"=w315) -> ()  [unwired: 2 in, 2 out]
                n157 = property on="Save Data As" class="Bool"("DisabledEnum"=w315) -> ()  [unwired: 2 in, 2 out]
                n158 = property on="O-Scope Mode" class="Bool"("DisabledEnum"=w315) -> ()  [unwired: 2 in, 2 out]
                n159 = Get Date/Time In Seconds() -> (seconds since 1Jan1904=w318:timestamp)
                n160 = Bundle By Name(cluster=w331, "O-Scope Mode"=TRUE, "Start Timestamp"=w318, "Buffer Size"=u32 100000, "Pause Graph"=FALSE, "Saving Path"=path "") -> (w330:T28)
              }
            }
          }
          event "Save Data As": Value Change {
            n161 = event-data() -> ()  [unwired: 1 in, 1 out]
            n162 = Unbundle By Name(w343) -> ("Data File Path"=w341:path, "Saving Path"=w340:path, "Data View Mode"=w339:bool)
            n163 = Select(t=w341, s=w339, f=w340) -> (s? t:f=w333:path)
            n164 = Strip Path(path=w333) -> (name=w338:string)  [unwired: 1 out]
            n165 = call "File Dialog2"("default name"=w338) -> ("selected path"=w332:path, "cancelled"=w336:bool, "error out"=w335:errorcluster)  [unwired: 11 in, 1 out]
            n166 = Unbundle By Name(w335) -> ("status"=w337:bool)
            n167 = Compound Arithmetic op=AND(invert w336, invert w337) -> (w334:bool)
            n168 = case shown="True" w334 {
              tunnel: w333 -> [_ w346]
              tunnel: w332 -> [_ w345]
              frame False {
              }
              frame True {
                n169 = Copy(9:TRUE ("overwrite (F)"), 10:w345, 11:w346) -> ()  [unwired: 2 in, 3 out]
              }
            }
          }
          event "Graph 1": Plot Attribute Change; "Graph 1": Scale Range Change; "Graph 1": Shortcut Menu Selection (App) {
            n170 = event-data() -> ()  [unwired: 1 in, 1 out]
            n171 = Unbundle By Name(w349) -> ("Data View Mode"=w350:bool)
            n172 = for {
              N: 16 -> [_]
              i -> [w369]
              n173 = property on="Graph 1" class="WFGraph (strict)"("Active Plot"=w369) -> ("Plot.Bar Plot Style"=w368:u8, "Plot.Fill To"=w367:i16, "Plot.Fill/Pt. Color"=w366:u32, "Plot.Label Style"=w365:u8, "Plot.Line Style"=w364:u8, "Plot.Line Width"=w363:u8, "Plot.Plot Color"=w362:u32, "Plot.Plot Interpolation"=w361:u8, "Plot.Point Style"=w360:u8)  [unwired: 2 in, 2 out]
              n174 = property on="Graph 2" class="WFGraph (strict)"("Active Plot"=w369, "Plot.Bar Plot Style"=w368, "Plot.Fill To"=w367, "Plot.Fill/Pt. Color"=w366, "Plot.Label Style"=w365, "Plot.Line Style"=w364, "Plot.Line Width"=w363, "Plot.Plot Color"=w362, "Plot.Plot Interpolation"=w361, "Plot.Point Style"=w360) -> ()  [unwired: 2 in, 2 out]
            }
            n175 = case shown="False" w350 {
              tunnel: [string[] ["Save Graph Settings"] ("f") string[] [] ("f")] -> w348
              frame False {
              }
              frame True {
              }
            }
            n176 = for {
              N: 2 -> [_]
              i -> [w357]
              n177 = property on="Graph 1" class="WFGraph (strict)"("ActYScl"=w357) -> ("YScale.ScaleFit"=w356:u8, "YScale.Maximum"=w359:dbl, "YScale.Minimum"=w358:dbl)  [unwired: 2 in, 2 out]
              n178 = property on="Graph 2" class="WFGraph (strict)"("ActYScl"=w357, "YScale.ScaleFit"=w356, "YScale.Maximum"=w359, "YScale.Minimum"=w358) -> ()  [unwired: 2 in, 2 out]
            }
          }
          event "Graph Range": Value Change {
            n179 = event-data() -> ()  [unwired: 1 in, 6 out]
            n180 = Unbundle By Name(w371) -> ("Data View Mode"=w372:bool)
            n181 = case shown="False" w372 {
              tunnel: [string[] ["Save Graph Settings"] ("f") string[] [] ("f")] -> w370
              frame False {
              }
              frame True {
              }
            }
          }
          event "Open": Value Change {
            n182 = event-data() -> ()  [unwired: 1 in, 6 out]
            n183 = Unbundle By Name(w382) -> ("Config Dir"=w381:path, "Config Extension"=w380:string)
            n184 = call "Config Select.vi"("Config Dir"=w381, "Config Extension"=w380) -> ("Load Config"=w379:bool, "Config Name"=w376:string)  [unwired: 15 in, 1 out]
            n185 = case shown="True" w379 {
              tunnel: [string[] [] string[] ["Cfg - Load"]] -> w383
              tunnel: w378 -> [w385 w388]
              tunnel: [w385 w387] -> w377
              tunnel: w376 -> [_ w386]
              frame False {
              }
              frame True {
                n186 = Bundle By Name(cluster=w388, "Config Name"=w386) -> (w387:T28)
              }
            }
          }
          event "Revert": Value Change {
            n187 = event-data() -> ()  [unwired: 1 in, 6 out]
            n188 = Bundle By Name(cluster=w393, "Revert"="Revert") -> (w392:T28)
          }
          event "Save": Value Change {
            n189 = event-data() -> ()  [unwired: 1 in, 6 out]
          }
          event "Save As": Value Change {
            n190 = event-data() -> ()  [unwired: 1 in, 6 out]
            n191 = Unbundle By Name(w399) -> ("Config Dir"=w398:path, "Config Extension"=w397:string, "Config Name"=w396:string)
            n192 = call "Config Save As.vi"("Config Dir"=w398, "Config Extension"=w397, "Config Name"=w396) -> ("Save As"=w403:bool, "Config Name OUT"=w400:string)  [unwired: 14 in, 1 out]
            n193 = case shown="True" w403 {
              tunnel: [string[] [] string[] ["Cfg - Store Channel Group", "Cfg - Save"]] -> w404
              tunnel: w402 -> [w406 w409]
              tunnel: [w406 w408] -> w401
              tunnel: w400 -> [_ w407]
              frame False {
              }
              frame True {
                n194 = Bundle By Name(cluster=w409, "Config Name"=w407) -> (w408:T28)
              }
            }
          }
          event "Add Sensor": Value Change {
            n195 = event-data() -> ()  [unwired: 1 in, 6 out]
          }
          event "Delete Sensor": Value Change {
            n196 = event-data() -> ()  [unwired: 1 in, 6 out]
          }
          event Value Change {
            n197 = event-data() -> ()  [unwired: 1 in, 6 out]
            n198 = Bundle By Name(cluster=w417, "Channel Display"="Sensors", "Changes?"=TRUE) -> (w416:T28)
          }
          event "DAQ Table": Key Down? {
            n199 = event-data() -> ("CtlRef"=w425:refnum<vi>, "VKey"=w424:T29, "Char"=w423:i16)  [unwired: 1 in]
            n200 = case shown="\"Enter\", \"Return\", \"Down\"" w424 {
              tunnel: [1 ("Column") 1 ("Column") -1 ("Column")] -> w429
              tunnel: [FALSE TRUE TRUE] -> w428
              frame Default {
              }
              frame "Enter", "Return", "Down" {
              }
              frame "Up" {
              }
            }
            n201 = Equal?(x=w423, y=i16 9) -> (x = y?=w426:bool)
            n202 = Or(x=w428, y=w426) -> (x .or. y?=w422:bool)
            n203 = case shown="True" w422 {
              tunnel: w425 -> [_ w440]
              tunnel: w429 -> [_ w435]
              frame False {
              }
              frame True {
                n204 = property class="Tbl (strict)"(reference=w440) -> (reference out=w437:refnum<vi>, "EditPos"=w439:T34)  [unwired: 1 in, 1 out]
                n205 = Unbundle(w439) -> ("Row"=w434:i32)  [unwired: 1 out]
                n206 = case shown="2" w434 {
                  selector: w434 -> [_ w448 _ w457]
                  tunnel: w434 -> [w443 w446 _ _]
                  tunnel: w435 -> [w442 w445 w456 w462]
                  tunnel: [w441 w447 w451 w458] -> w433
                  frame Default {
                    n207 = Add(x=w442, y=w443) -> (x+y=w441:i32)
                  }
                  frame 2 {
                    n208 = Equal?(x=w445, y=-1) -> (x = y?=w449:bool)
                    n209 = Add(x=w446, y=w445) -> (x+y=w444:i32)
                    n210 = Select(t=w448, s=w449, f=w444) -> (s? t:f=w447:i32)
                  }
                  frame 5 {
                    n211 = Equal?(x=w456, y=-1) -> (x = y?=w455:bool)
                    n212 = Select(t=4, s=w455, f=7) -> (s? t:f=w451:i32)
                  }
                  frame 7 {
                    n213 = Equal?(x=w462, y=-1) -> (x = y?=w461:bool)
                    n214 = Select(t=5, s=w461, f=w457) -> (s? t:f=w458:i32)
                  }
                }
                n215 = In Range and Coerce(upper limit=7 ("y"), x=w433, lower limit=2) -> (coerced(x)=w432:i32)  [unwired: 1 out]
                n216 = Bundle("y"=w432, "Column"=0) -> (w438:cluster{"y":i32, "Column":i32})  [unwired: 1 in]
                n217 = property class="Tbl (strict)"(reference=w437, "EditPos"=w438) -> ()  [unwired: 1 in, 2 out]
              }
            }
            n218 = event-data("Discard?"=w422) -> ()  [unwired: 1 in, 1 out]
          }
          event "Header Table:": Value Change {
            n219 = event-data() -> ()  [unwired: 1 in, 6 out]
            n220 = Index Array(array="Header Table:", index (col)=0 ("disabled index (col)")) -> (element=w474:string[])  [unwired: 1 in]
            n221 = Array To Cluster(array=w474) -> (cluster=w476:T35)
            n222 = Bundle By Name(cluster=w472, "Config.Header"=w476, "Changes?"=TRUE) -> (w471:T28)
          }
          event "Header Table:": Key Down {
            w483 = i16 9  # Tab
            n223 = event-data() -> ("CtlRef"=w485:refnum<vi>, "Char"=w484:i16, "VKey"=w478:T29)  [unwired: 1 in, 7 out]
            n224 = Equal?(x=w484, y=w483) -> (x = y?=w482:bool)
            n225 = Equal?(x=w478, y=eventvkey."Enter" ("VKey")) -> (x = y?=w481:bool)
            n226 = Equal?(x=w478, y=eventvkey."Return" ("VKey")) -> (x = y?=w477:bool)
            n227 = Compound Arithmetic op=OR(w482, w481, w477) -> (w480:bool)
            n228 = case shown="True" w480 {
              tunnel: w485 -> [_ w493]
              frame False {
              }
              frame True {
                n229 = property class="Tbl (strict)"(reference=w493, "Key Focus"=TRUE) -> (reference out=w492:refnum<vi>, "Selection Start"=w491:T34)  [unwired: 1 in, 1 out]
                n230 = Unbundle(w491) -> ("Row"=w489:i32)  [unwired: 1 out]
                n231 = case shown="0..2" w489 {
                  tunnel: w489 -> [_ w500]
                  tunnel: w492 -> [w495 w498]
                  frame Default {
                    n232 = property class="Tbl (strict)"(reference=w495, "Key Focus"=FALSE) -> ()  [unwired: 1 in, 2 out]
                  }
                  frame 0..2 {
                    n233 = Increment(x=w500) -> (x+1=w499:i32)
                    n234 = Bundle(w499, "Column"=0) -> (w496:cluster{i32, "Column":i32})  [unwired: 1 in]
                    n235 = property class="Tbl (strict)"(reference=w498, "EditPos"=w496, "Selection Start"=w496) -> ()  [unwired: 1 in, 2 out]
                  }
                }
              }
            }
          }
          event "DAQ Table": Value Change {
            n236 = event-data() -> ()  [unwired: 1 in, 6 out]
            n237 = Index Array(array="DAQ Table", index (col)=0 ("disabled index (col)")) -> (element=w507:string[])  [unwired: 1 in]
            n238 = for {
              tunnel: w507 -> [w525] mode=indexing
              tunnel: [w523] -> w509 mode=indexing
              n239 = Match Pattern(string=w525, regular expression="[.]") -> (before substring=w531:string, after substring=w524:string, offset past match=w529:i32)  [unwired: 1 in, 1 out]
              n240 = Decimal Digit?(1:w531) -> (0:w530:bool)
              n241 = Equal?(x=w529, y=-1) -> (x = y?=w527:bool)
              n242 = Or(x=w530, y=w527) -> (x .or. y?=w526:bool)
              n243 = case shown="True" w526 {
                tunnel: [w533 w536] -> w523
                tunnel: w525 -> [_ w536]
                tunnel: w524 -> [w535 _]
                frame False {
                  n244 = Concatenate Strings("0." ("string"), w535) -> (w533:string)
                }
                frame True {
                }
              }
            }
            n245 = Index Array(array=w509, index #1=2 ("index"), index #5=7 ("index")) -> (element #1=w512:string, element #2=w514:string, element #3=w516:string, element #4=w518:string, element #5=w520:string, element #6=w502:string)  [unwired: 4 in]
            n246 = Fract/Exp String To Number(string=w512) -> (number=w513:dbl)  [unwired: 3 in, 1 out]
            n247 = Decimal String To Number(string=w514) -> (number=w515:i32)  [unwired: 2 in, 1 out]
            n248 = Decimal String To Number(string=w516) -> (number=w517:i32)  [unwired: 2 in, 1 out]
            n249 = Fract/Exp String To Number(string=w518) -> (number=w519:dbl)  [unwired: 3 in, 1 out]
            n250 = Fract/Exp String To Number(string=w520) -> (number=w521:dbl)  [unwired: 3 in, 1 out]
            n251 = Fract/Exp String To Number(string=w502) -> (number=w501:dbl)  [unwired: 3 in, 1 out]
            n252 = Bundle By Name(cluster=w506, "Config.DAQ Settings.Trigger Value"=w513, "Config.DAQ Settings.Trigger Samples"=w515, "Config.DAQ Settings.Pretrigger Samples"=w517, "Config.DAQ Settings.Trigger Interval"=w519, "Config.DAQ Settings.Sample Rate"=w521, "Config.DAQ Settings.Log Rate"=w501, "Changes?"=TRUE) -> (w505:T28)
          }
          event "Limit:": Value Change {
            n253 = event-data() -> ()  [unwired: 1 in, 6 out]
            n254 = Bundle By Name(cluster=w540, "Config.DAQ Settings.File Size Limit"="Limit:", "Changes?"=TRUE) -> (w539:T28)
          }
          event "DAQ Table": Mouse Down? {
            n255 = event-data() -> ("Coords"=w542:T36)  [unwired: 1 in]
            n256 = invoke on="DAQ Table" class="Tbl (strict)" method="Point To Row Column"("Point"=w542) -> ("CellPosition"=w548:T34)  [unwired: 5 in, 5 out]
            n257 = Unbundle By Name(w548) -> ("Row"=w549:i32)
            n258 = case shown="1" w549 {
              tunnel: w545 -> [w552 w558]
              tunnel: [w552 w557] -> w546
              tunnel: [string[] [] string[] ["Cfg - Update DAQ Table"]] -> w543
              tunnel: [FALSE ("Discard?") TRUE ("Discard?")] -> w544
              tunnel: w547 -> [_ w553]
              frame 0, Default {
              }
              frame 1 {
                n259 = Unbundle By Name(w553) -> ("Config"=w559:T16)
                n260 = call "Select Analog Trigger Channel.vi"("Config"=w559) -> ("Config out"=w560:T16)  [unwired: 14 in]
                n261 = Bundle By Name(cluster=w558, "Config"=w560, "Changes?"=TRUE) -> (w557:T28)
              }
            }
            n262 = event-data("Discard?"=w544) -> ()  [unwired: 1 in, 1 out]
          }
          event "Trigger Type": Value Change {
            n263 = event-data() -> ()  [unwired: 1 in, 6 out]
            n264 = Bundle By Name(cluster=w564, "Config.DAQ Settings.Trigger Type"="Trigger Type", "Changes?"=TRUE) -> (w563:T28)
          }
          event "Save Mode": Value Change {
            n265 = event-data() -> ()  [unwired: 1 in, 6 out]
            n266 = Bundle By Name(cluster=w569, "Config.DAQ Settings.Save Mode"="Save Mode", "Changes?"=TRUE) -> (w568:T28)
          }
          event "Trigger Stop Method": Value Change {
            n267 = event-data() -> ()  [unwired: 1 in, 6 out]
            n268 = Bundle By Name(cluster=w574, "Config.DAQ Settings.Trigger Stop Method"="Trigger Stop Method", "Changes?"=TRUE) -> (w573:T28)
          }
          event "Minutes": Value Change {
            n269 = event-data() -> ()  [unwired: 1 in, 6 out]
            n270 = Not(x="Minutes") -> (.not. x?=w580:bool)
            n271 = Bundle By Name(cluster=w579, "Changes?"=TRUE, "Config.DAQ Settings.Time Units"=w580) -> (w578:T28)
            n272 = local write "Hours"(w580) -> ()
          }
          event "Hours": Value Change {
            n273 = event-data() -> ()  [unwired: 1 in, 6 out]
            n274 = Not(x="Hours") -> (.not. x?=w586:bool)
            n275 = local write "Minutes"(w586) -> ()
            n276 = Bundle By Name(cluster=w585, "Changes?"=TRUE, "Config.DAQ Settings.Time Units"="Hours") -> (w584:T28)
          }
          event "Sample Sec": Value Change {
            # "False = Sec\nTrue = Min"
            n277 = event-data() -> ()  [unwired: 1 in, 6 out]
            n278 = Not(x="Sample Sec") -> (.not. x?=w593:bool)
            n279 = local write "Sample Min"(w593) -> ()
            n280 = Bundle By Name(cluster=w591, "Changes?"=TRUE, "Config.DAQ Settings.Rate Sec/Min"=w593) -> (w590:T28)
          }
          event "Sample Min": Value Change {
            # "False = Sec\nTrue = Min"
            n281 = event-data() -> ()  [unwired: 1 in, 6 out]
            n282 = Not(x="Sample Min") -> (.not. x?=w598:bool)
            n283 = local write "Sample Sec"(w598) -> ()
            n284 = Bundle By Name(cluster=w597, "Changes?"=TRUE, "Config.DAQ Settings.Rate Sec/Min"="Sample Min") -> (w596:T28)
          }
          event "Log Sec": Value Change {
            # "False = Sec\nTrue = Min"
            n285 = event-data() -> ()  [unwired: 1 in, 6 out]
            n286 = Not(x="Log Sec") -> (.not. x?=w605:bool)
            n287 = local write "Log Min"(w605) -> ()
            n288 = Bundle By Name(cluster=w603, "Changes?"=TRUE, "Config.DAQ Settings.Rate Sec/Min (Log)"=w605) -> (w602:T28)
          }
          event "Log Min": Value Change {
            # "False = Sec\nTrue = Min"
            n289 = event-data() -> ()  [unwired: 1 in, 6 out]
            n290 = Not(x="Log Min") -> (.not. x?=w606:bool)
            n291 = local write "Log Sec"(w606) -> ()
            n292 = Bundle By Name(cluster=w610, "Changes?"=TRUE, "Config.DAQ Settings.Rate Sec/Min (Log)"="Log Min") -> (w609:T28)
          }
          event "Auto Save": Value Change {
            n293 = event-data() -> ()  [unwired: 1 in, 6 out]
            n294 = Bundle By Name(cluster=w615, "Config.DAQ Settings.Auto Save"="Auto Save", "Changes?"=TRUE) -> (w614:T28)
          }
          event "Data Base Path:": Value Change {
            n295 = event-data() -> ("OldVal"=w617:path)  [unwired: 1 in, 5 out]
            n296 = call <vilib>:"Check if File or Folder Exists.vi"("path"="Data Base Path:") -> ("file or folder exists?"=w620:bool, "dup path"=w619:path)  [unwired: 8 in, 1 out]
            n297 = case shown="False" w620 {
              tunnel: [w626 w628] -> w618
              tunnel: w619 -> [_ w628]
              tunnel: w617 -> [w626 _]
              frame False {
                n298 = One Button Dialog(message="Desired folder does not exist!") -> ()  [unwired: 1 in, 1 out]
              }
              frame True {
              }
            }
            n299 = Bundle By Name(cluster=w624, "Config.Data Base Path"=w618, "Load Prompt"=FALSE) -> (w622:T28)
          }
          event "Import from CSV": Value Change {
            n300 = event-data() -> ()  [unwired: 1 in, 6 out]
            n301 = Two Button Dialog(message="Are you sure you want to do this?\n\nThis will overwrite the data of any sensor with the same gauge number.", 1:"Abort" ("T button name (\"OK\")"), 2:"Proceed" ("T button name (\"OK\")")) -> (T button?=w629:bool)
            n302 = case shown="True" w629 {
              tunnel: [string[] [] string[] ["Cfg - Import from CSV"]] -> w634
              frame False {
              }
              frame True {
              }
            }
          }
          event "Synch Files": Value Change {
            n303 = event-data() -> ()  [unwired: 1 in, 6 out]
            n304 = call <vilib>:"Set Busy.vi"() -> ()  [unwired: 10 in, 2 out]
          }
          event "Show Big Data": Value Change {
            n305 = event-data() -> ()  [unwired: 1 in, 6 out]
            n306 = Unbundle By Name(w644) -> ("Graph Ch Refs"=w643:refnum<vi>[])
            n307 = property on="Graph Colors (Big)" class="Clust (strict)"() -> ("Controls[]"=w639:refnum<vi>[])  [unwired: 2 in, 2 out]
            n308 = for {
              N: 8 -> [_]
              tunnel: w643 -> [w652] mode=indexing
              tunnel: [w651] -> w641 mode=indexing
              tunnel: w639 -> [w648] mode=indexing
              i -> [w650]
              n309 = property class="Ring"(reference=w652) -> ("RingText.Text"=w651:string)  [unwired: 1 in, 2 out]
              n310 = property on="Graph 1" class="WFGraph (strict)"("Active Plot"=w650) -> ("Plot.Plot Color"=w649:u32)  [unwired: 2 in, 2 out]
              n311 = property class="Ctl"(reference=w648, "Value"=w649) -> ()  [unwired: 1 in, 2 out]
            }
            n312 = property on="Big Data Tab" class="TabCtl (strict)"("Visible"="Show Big Data") -> ()  [unwired: 2 in, 2 out]
            n313 = Array To Cluster(array=w641) -> (cluster=→"Graph Channels (Big)":T37)
          }
          event "Add Data Point": Value Change {
            n314 = event-data() -> ()  [unwired: 1 in, 6 out]
            n315 = Unbundle By Name(w657) -> ("Virtual Trigger"=w655:bool, "Manual Data Mode"=w654:bool)
            n316 = Not(x=w655) -> (.not. x?=w656:bool)
            n317 = Compound Arithmetic op=AND(invert w655, invert w654) -> (w653:bool)
            n318 = case shown="True" w653 {
              tunnel: [string[] [] string[] ["Start Log"]] -> w661
              frame False {
              }
              frame True {
              }
            }
            n319 = Bundle By Name(cluster=w660, "Add Data Point"="Add Data Point", "Manual Data Mode"=w656) -> (w659:T28)
          }
        }
        n320 = call "Insert Multiple Events.vi"("Insert all? (T)"=TRUE, "Events to Insert"=w80, "Event queue in"=w81) -> ("Event queue out"=w82:string[])  [unwired: 4 in]
      }
      frame "Init" {
        w670 = T30."Enabled" ("Disabled")
        w664 = u8 2 ("Disabled")
        w686 = string[] [""] ("Strings []")
        n321 = property class="App"() -> ("App.Kind"=w681:T38)  [unwired: 2 in, 2 out]
        n322 = local write "Graph Numerics"(T5 {"Y1 RT"=0.0, "Y2 RT"=0.0, "Y3 RT"=0.0, "Y4 RT"=0.0, "Y5 RT"=0.0, "Y6 RT"=0.0, "Y1 RT 2"=0.0, "Y2 RT 2"=0.0, "Y3 RT 2"=0.0, "Y4 RT 2"=0.0, "Y5 RT 2"=0.0, "Y6 RT 2"=0.0, "Y3 RT 3"=0.0, "Y4 RT 3"=0.0, "Y5 RT 3"=0.0, "Y6 RT 3"=0.0} ("Graph Numerics")) -> ()
        n323 = local write "Graph Numerics (Big)"(T2 {"Y1 RT 2"=0.0, "Y1 RT 3"=0.0, "Y1 RT 4"=0.0, "Y1 RT 5"=0.0, "Y1 RT 6"=0.0, "Y1 RT 7"=0.0, "Y1 RT 8"=0.0, "Y1 RT 9"=0.0} ("Graph Numerics (Big)")) -> ()
        n324 = case shown="\"Run Time System\"" w681 {
          tunnel: ["TI cDAQ, Debug" ("Name and Version") w691] -> w680
          frame Default {
          }
          frame "Run Time System" {
            n325 = call "Get Version from EXE.vi"("EXE Name"="TI cDAQ.exe") -> ("Name and Version"=w691:string)  [unwired: 12 in, 2 out]
          }
        }
        "Title" <- w680
        n326 = property on="Y1" class="Ring (strict)"("Strings []"=w686) -> ()  [unwired: 2 in, 2 out]
        n327 = property on="Y2" class="Ring (strict)"("Strings []"=w686) -> ()  [unwired: 2 in, 2 out]
        n328 = property on="Y4" class="Ring (strict)"("Strings []"=w686) -> ()  [unwired: 2 in, 2 out]
        n329 = property on="Y3" class="Ring (strict)"("Strings []"=w686) -> ()  [unwired: 2 in, 2 out]
        n330 = property on="Y6" class="Ring (strict)"("Strings []"=w686) -> ()  [unwired: 2 in, 2 out]
        n331 = property on="Y5" class="Ring (strict)"("Strings []"=w686) -> ()  [unwired: 2 in, 2 out]
        n332 = property class="VI"("Front Panel.Title"=w680) -> ()  [unwired: 2 in, 2 out]
        n333 = property on="Add Data Point" class="Bool"("Disabled"=w664) -> ()  [unwired: 2 in, 2 out]
        n334 = property on="Arm DAQ" class="Bool"("Disabled"=w664) -> ()  [unwired: 2 in, 2 out]
        n335 = property on="Start Log" class="Bool"("Disabled"=w664) -> ()  [unwired: 2 in, 2 out]
        n336 = property on="Stop DAQ" class="Bool"("Disabled"=w664) -> ()  [unwired: 2 in, 2 out]
        n337 = property on="Disarm DAQ" class="Bool"("Disabled"=w664) -> ()  [unwired: 2 in, 2 out]
        n338 = property on="O-Scope Mode" class="Bool"("DisabledEnum"=w664) -> ()  [unwired: 2 in, 2 out]
        n339 = property on="Save Data As" class="Bool"("DisabledEnum"=w664) -> ()  [unwired: 2 in, 2 out]
        n340 = local write "Acquiring Data 2"(FALSE ("Acquiring Data")) -> ()
        n341 = local write "Main Tab"(enum32{" Main", "Configure"}."Configure" ("Main Tab")) -> ()
        n342 = local write "Show Big Data"(FALSE ("Show Big Data")) -> ()
        n343 = property on="Acquiring Tab" class="TabCtl (strict)"("Visible"=FALSE) -> ()  [unwired: 2 in, 2 out]
        n344 = property on="Connecting Tab" class="TabCtl (strict)"("Visible"=FALSE) -> ()  [unwired: 2 in, 2 out]
        n345 = property on="Big Data Tab" class="TabCtl (strict)"("Visible"=FALSE) -> ()  [unwired: 2 in, 2 out]
        n346 = property on="Open File" class="Bool"("DisabledEnum"=T30."Enabled" ("Disabled")) -> ()  [unwired: 2 in, 2 out]
        n347 = property on="Decoration Tab" class="TabCtl (strict)"("DisabledEnum"=T30."Disabled and Grayed Out" ("Disabled")) -> ()  [unwired: 2 in, 2 out]
        n348 = Current VI's Path() -> (path=w675:path)
        n349 = call "Get Paths.vi"("Path IN"=w675) -> ("App Path"=w671:path)  [unwired: 10 in]
        n350 = property on="Header Table:" class="Tbl (strict)"("DisabledEnum"=w670) -> ()  [unwired: 2 in, 2 out]
        n351 = property on="Data Base Path:" class="Path"("DisabledEnum"=w670) -> ()  [unwired: 2 in, 2 out]
        n352 = Build Path(base path=w671, name or relative path="App Config.ini") -> (appended path=w677:path)
        n353 = Bundle By Name(cluster=w676, "App Path"=w671, "App Config Path"=w677, "Virtual Trigger"=FALSE, "Sensor File Name"="Sensors.scl" ("name or relative path"), "Sys Cfg File Name"="Systems Config.ini" ("name or relative path")) -> (w688:T28)
      }
      frame "Init Test Start Data" {
        w692 = u32 0 ("Samples Recorded")
        w696 = T30."Disabled and Grayed Out" ("Disabled")
        w697 = 0.0 ("Elapsed Time:")
        n354 = property on="Start of Test:" class="AbsTime (strict)"("DisabledEnum"=w696) -> ()  [unwired: 2 in, 2 out]
        n355 = property on="Elapsed Time:" class="DigNum (strict)"("DisabledEnum"=w696) -> ()  [unwired: 2 in, 2 out]
        n356 = property on="Samples Recorded:" class="DigNum (strict)"("DisabledEnum"=w696) -> ()  [unwired: 2 in, 2 out]
        n357 = local write "Elapsed Time:"(w697) -> ()
        n358 = To Time Stamp(1:w697) -> (0:w693:timestamp)
        n359 = local write "Start of Test:"(w693) -> ()
        n360 = Bundle By Name(cluster=w695, "Start Timestamp"=w693, "Samples Recorded"=w692) -> (w694:T28)
        n361 = local write "Samples Recorded:"(w692) -> ()
      }
      frame "Read App Config" {
        n362 = Unbundle By Name(w714) -> ("Sensor File Name"=w699:string, "App Path"=w708:path, "App Config Path"=w712:path, "App Config"=w709:T13)
        n363 = call <vilib>:"Open Config Data.vi"("configuration file path"=w712) -> ("file created?"=w711:bool, "refnum"=w710:T39)  [unwired: 8 in, 1 out]
        n364 = case shown="True" w711 {
          tunnel: w710 -> [w720 _]
          tunnel: w709 -> [w717 w728]
          tunnel: [w716 w729] -> w704
          tunnel: w708 -> [_ w727]
          tunnel: [string[] [] ("Events to Insert") string[] ["Save App Config"] ("Events to Insert")] -> w705
          frame False {
            n365 = call <userlib>:"Read INI Cluster__ogtk.vi"("INI Fomatted Cluster Type"=w717, "refnum"=w720) -> ("INI Fomatted Cluster"=w718:variant, "dup refnum"=w719:T39)  [unwired: 5 in, 3 out]
            n366 = call <vilib>:"Close Config Data.vi"("refnum"=w719) -> ()  [unwired: 9 in, 2 out]
            n367 = Variant To Data(type=w717, Variant=w718) -> (data=w716:T13)  [unwired: 1 in, 1 out]
          }
          frame True {
            w721 = "" ("Last Config (Std)")
            n368 = Build Path(base path=w727, name or relative path="Support") -> (appended path=w725:path)
            n369 = Bundle By Name(cluster=w728, "Support Dir (Local)"=w725, "Support Dir (Remote)"=path "S:/GLOBALTEST/Software/TI cDAQ/Support", "Config Sub Dir"="Configurations", "Last Config (Std)"=w721, "Last Config (Def)"=w721, "Last Config (8TC)"=w721) -> (w729:T13)
          }
        }
        n370 = Unbundle By Name(w704) -> ("Support Dir (Local)"=w703:path, "Config Sub Dir"=w702:string)
        n371 = Build Path(base path=w703, name or relative path=w699) -> (appended path=w701:path)
        n372 = Build Path(base path=w703, name or relative path=w702) -> (appended path=w700:path)
        n373 = call "Insert Multiple Events.vi"("Events to Insert"=w705, "Event queue in"=w706) -> ("Event queue out"=w707:string[])  [unwired: 5 in]
        n374 = Bundle By Name(cluster=w714, "App Config"=w704, "Calibration Path"=w701, "Config Dir"=w700) -> (w713:T28)
      }
      frame "Save App Config" {
        n375 = Unbundle By Name(w739) -> ("App Config Path"=w742:path, "System Type"=w733:T15, "App Config"=w732:T13, "Config Name"=w730:string)
        n376 = case shown="\"Standard 8TC\"" w733 {
          tunnel: w732 -> [w745 w748 w751]
          tunnel: [w744 w747 w750] -> w731
          tunnel: w730 -> [w743 w746 w749]
          frame "Standard", Default {
            n377 = Bundle By Name(cluster=w745, "Last Config (Std)"=w743) -> (w744:T13)
          }
          frame "Deformation" {
            n378 = Bundle By Name(cluster=w748, "Last Config (Def)"=w746) -> (w747:T13)
          }
          frame "Standard 8TC" {
            n379 = Bundle By Name(cluster=w751, "Last Config (8TC)"=w749) -> (w750:T13)
          }
        }
        n380 = call <vilib>:"Open Config Data.vi"("configuration file path"=w742) -> ("error out"=w735:errorcluster, "refnum"=w737:T39)  [unwired: 8 in, 1 out]
        n381 = call <userlib>:"Write INI Cluster__ogtk.vi"("error in (no error)"=w735, "INI Fomatted Cluster"=w731, "refnum"=w737) -> ("error out"=w734:errorcluster, "dup refnum"=w736:T39)  [unwired: 7 in]
        n382 = call <vilib>:"Close Config Data.vi"("error in (no error)"=w734, "refnum"=w736) -> ()  [unwired: 8 in, 2 out]
        n383 = call "Insert Multiple Events.vi"("Events to Insert"=string[] [], "Event queue in"=w740) -> ("Event queue out"=w741:string[])  [unwired: 5 in]
      }
      frame "Get Systems Config" {
        n384 = Unbundle By Name(w760) -> ("Sys Cfg File Name"=w752:string, "App Config.Support Dir (Remote)"=w758:path, "App Config.Support Dir (Local)"=w757:path)
        n385 = Build Path(base path=w758, name or relative path=w752) -> (appended path=w756:path)
        n386 = Build Path(base path=w757, name or relative path=w752) -> (appended path=w755:path)
        n387 = Copy(9:TRUE ("overwrite (F)"), 10:w755, 11:w756) -> (0:w753:errorcluster)  [unwired: 2 in, 2 out]
        n388 = call <vilib>:"Clear Errors.vi"("error in (no error)"=w753) -> ()  [unwired: 5 in, 2 out]
        n389 = call "Insert Multiple Events.vi"("Events to Insert"=string[] [], "Event queue in"=w761) -> ("Event queue out"=w762:string[])  [unwired: 5 in]
      }
      frame "Synch Files with Server" {
        n390 = Unbundle By Name(w767) -> ("App Config"=w766:T13, "Sensor File Name"=w765:string)
        n391 = call "Synch with Server.vi"("Sensor File Name"=w765, "App Config"=w766) -> ("Error OUT"=w763:errorcluster)  [unwired: 9 in]
        n392 = flat-sequence {
          tunnel: w763 -> [_]
          frame #0 {
            n393 = call <vilib>:"Unset Busy.vi"() -> ()  [unwired: 11 in, 1 out]
          }
        }
        n394 = case shown="No Error" w763 {
          tunnel: [string[] ["Cfg - Load Sensors", "Cfg - Update Channel Group", "Cfg - Load"] ("Events to Insert") string[] [] ("Events to Insert")] -> w769
          frame No Error {
          }
          frame Error {
          }
        }
        n395 = call "Insert Multiple Events.vi"("Events to Insert"=w769, "Event queue in"=w768) -> ("Event queue out"=w764:string[])  [unwired: 5 in]
      }
      frame "Unused Items" {
      }
      frame "Disable Buttons" {
        w774 = u8 2 ("Disabled")
        n396 = property on="Arm DAQ" class="Bool"("Disabled"=w774) -> ()  [unwired: 2 in, 2 out]
        n397 = property on="Start Log" class="Bool"("Disabled"=w774) -> ()  [unwired: 2 in, 2 out]
        n398 = property on="Stop DAQ" class="Bool"("Disabled"=w774) -> ()  [unwired: 2 in, 2 out]
        n399 = property on="Disarm DAQ" class="Bool"("Disabled"=w774) -> ()  [unwired: 2 in, 2 out]
        n400 = property on="Add Data Point" class="Bool"("Disabled"=w774) -> ()  [unwired: 2 in, 2 out]
      }
      frame "Data View Mode" {
        w780 = T30."Disabled" ("Disabled")
        w779 = T30."Disabled and Grayed Out" ("Disabled")
        w791 = TRUE ("Visible")
        w792 = T30."Disabled" ("Disabled")
        w794 = sgl[][] [] ("Graph")
        n401 = control-ref of="Main Tab"() -> (w790:refnum<vi>)
        n402 = local write "Graph Numerics"(T5 {"Y1 RT"=0.0, "Y2 RT"=0.0, "Y3 RT"=0.0, "Y4 RT"=0.0, "Y5 RT"=0.0, "Y6 RT"=0.0, "Y1 RT 2"=0.0, "Y2 RT 2"=0.0, "Y3 RT 2"=0.0, "Y4 RT 2"=0.0, "Y5 RT 2"=0.0, "Y6 RT 2"=0.0, "Y3 RT 3"=0.0, "Y4 RT 3"=0.0, "Y5 RT 3"=0.0, "Y6 RT 3"=0.0} ("Graph Numerics")) -> ()
        n403 = local write "Graph Numerics (Big)"(T2 {"Y1 RT 2"=0.0, "Y1 RT 3"=0.0, "Y1 RT 4"=0.0, "Y1 RT 5"=0.0, "Y1 RT 6"=0.0, "Y1 RT 7"=0.0, "Y1 RT 8"=0.0, "Y1 RT 9"=0.0} ("Graph Numerics (Big)")) -> ()
        n404 = property on="Load Indicator Tab" class="TabCtl (strict)"("Visible"=w791) -> ()  [unwired: 2 in, 2 out]
        n405 = property on="Mode Exit" class="Bool"("Visible"=w791) -> ()  [unwired: 2 in, 2 out]
        n406 = property on="Status" class="Str"("Visible"=w791) -> ()  [unwired: 2 in, 2 out]
        n407 = property on="Status" class="Str"("Text.BGColor"=u32 16768256) -> ()  [unwired: 2 in, 2 out]
        n408 = local write "Graph 1"(w794) -> ()
        n409 = local write "Graph 2"(w794) -> ()
        n410 = property on="Play" class="Bool (strict)"("DisabledEnum"=w792) -> ()  [unwired: 2 in, 2 out]
        n411 = property on="Pause" class="Bool (strict)"("DisabledEnum"=w792) -> ()  [unwired: 2 in, 2 out]
        n412 = property class="TabCtl (strict)"(reference=w790) -> ("Pages"=w789:refnum<vi>[])  [unwired: 1 in, 2 out]
        n413 = Index Array(array=w789, index=1) -> (element=w787:refnum<vi>)
        n414 = property class="Page"(reference=w787, "PageEnb"=T31."Page Disabled & Grayed" ("Page Enabled State")) -> ()  [unwired: 1 in, 2 out]
        n415 = property on="Decoration Tab" class="TabCtl (strict)"("DisabledEnum"=w780) -> ()  [unwired: 2 in, 2 out]
        n416 = property on="Graph Channels" class="Clust (strict)"("DisabledEnum"=w780) -> ()  [unwired: 2 in, 2 out]
        n417 = property on="Arm DAQ" class="Bool"("DisabledEnum"=w779) -> ()  [unwired: 2 in, 2 out]
        n418 = property on="O-Scope Mode" class="Bool"("DisabledEnum"=w779) -> ()  [unwired: 2 in, 2 out]
        n419 = local write "Status"("IN DATA VIEW MODE..." ("Status")) -> ()
        n420 = Bundle By Name(cluster=w784, "Data View Mode"=TRUE, "Saving Path"=path "") -> (w783:T28)
      }
      frame "Exit Mode" {
        w812 = FALSE
        w814 = sgl[][] [] ("Graph")
        w821 = FALSE ("Visible")
        n421 = Unbundle By Name(w811) -> ("O-Scope Mode"=w805:bool, "Config Dir"=w810:path, "Title Bar"=w796:refnum<vi>)
        n422 = property on="Mode Exit" class="Bool"("Visible"=w821) -> ()  [unwired: 2 in, 2 out]
        n423 = property on="Status" class="Str"("Visible"=w821) -> ()  [unwired: 2 in, 2 out]
        n424 = control-ref of="Main Tab"() -> (w820:refnum<vi>)
        n425 = Empty String/Path?(string/path=w810) -> (empty?=w801:bool)
        n426 = property class="TabCtl (strict)"(reference=w820) -> ("Pages"=w819:refnum<vi>[])  [unwired: 1 in, 2 out]
        n427 = case shown="False" w801 {
          frame False {
            w830 = T30."Enabled" ("Disabled")
            n428 = property on="Arm DAQ" class="Bool"("DisabledEnum"=w830) -> ()  [unwired: 2 in, 2 out]
            n429 = property on="Open File" class="Bool"("DisabledEnum"=w830) -> ()  [unwired: 2 in, 2 out]
            n430 = property on="O-Scope Mode" class="Bool"("DisabledEnum"=w830) -> ()  [unwired: 2 in, 2 out]
          }
          frame True {
          }
        }
        n431 = local read "Title"() -> (w797:string)
        n432 = case shown="True" w805 {
          frame False {
          }
          frame True {
            n433 = call "Configure DAQ (by ref).vi"("Mode"=enum16{"Init", "Acquire", "Clear"}."Clear") -> ()  [unwired: 19 in, 8 out]
          }
        }
        n434 = Current VI's Path() -> (path=w815:path)
        n435 = call "Set Window Title using Path.vi"("VI path"=w815, "Title Bar"=w796, "Title"=w797) -> ()  [unwired: 12 in, 1 out]
        n436 = Index Array(array=w819, index=1) -> (element=w817:refnum<vi>)
        n437 = property class="Page"(reference=w817, "PageEnb"=T31."Page Enabled" ("Page Enabled State")) -> ()  [unwired: 1 in, 2 out]
        n438 = property on="Graph Channels" class="Clust (strict)"() -> ("Controls[]"=w808:refnum<vi>[])  [unwired: 2 in, 2 out]
        n439 = local write "Graph 1"(w814) -> ()
        n440 = local write "Graph 2"(w814) -> ()
        n441 = property on="Save Data As" class="Bool"("DisabledEnum"=T30."Disabled and Grayed Out" ("Disabled")) -> ()  [unwired: 2 in, 2 out]
        n442 = for {
          tunnel: w808 -> [w829] mode=indexing
          tunnel: [FALSE] -> w809 mode=indexing
          n443 = To More Specific Class(target class=refnum<vi> refnum ("Ring"), reference=w829) -> (specific class reference=w827:refnum<vi>)  [unwired: 1 in, 1 out]
          n444 = property class="Ring"(reference=w827, "Strings []"=string[] [""]) -> (reference out=w828:refnum<vi>)  [unwired: 1 in, 1 out]
          n445 = property class="Ring"(reference=w828, "Value"=0 ("index")) -> ()  [unwired: 1 in, 2 out]
        }
        n446 = Array To Cluster(array=w809) -> (cluster=w798:T33)
        n447 = local write "Graph Toggles"(w798) -> ()
        n448 = local write "Axis Toggles"(w798) -> ()
        n449 = Not(x=w801) -> (.not. x?=w800:bool)
        n450 = call "Insert Multiple Events.vi"("Insert all? (T)"=w800, "Events to Insert"=string[] ["Open Config File"], "Event queue in"=w802) -> ("Event queue out"=w803:string[])  [unwired: 4 in]
        n451 = Bundle By Name(cluster=w811, "O-Scope Mode"=w812, "Data View Mode"=w812) -> (w813:T28)
        n452 = call "Insert Multiple Events.vi"("Events to Insert"=string[] ["Update Graph Toggles", "Update Axis Toggles"], "Event queue in"=w803) -> ("Event queue out"=w806:string[])  [unwired: 5 in]
      }
      frame "Open Data File" {
        w847 = TRUE ("Pause Graph")
        n453 = Unbundle By Name(w867) -> ("Data File Path"=w845:path, "Title Bar"=w832:refnum<vi>)
        n454 = local read "Title"() -> (w833:string)
        n455 = Current VI's Path() -> (path=w846:path)
        n456 = property on="Save Data As" class="Bool"("DisabledEnum"=T30."Enabled" ("Disabled")) -> ()  [unwired: 2 in, 2 out]
        n457 = call "Set Window Title using Path.vi"("VI path"=w846, "Title Bar"=w832, "File Path"=w845, "Title"=w833) -> ()  [unwired: 11 in, 1 out]
        n458 = call-poly <vilib>:"Read Delimited Spreadsheet.vi"("file path (dialog if empty)"=w845, "delimiter (\\t)"="," ("delimiter (\\t)")) -> ("all rows"=w831:string[][])  [unwired: 8 in, 5 out]
        n459 = Delete From Array(array=w831, length=5 ("index (row)"), index (row)=0) -> (deleted portion=w863:string[][], array with subset deleted=w840:string[][])  [unwired: 1 in]
        n460 = Index Array(array=w831, index (row)=0, index (col)=0 ("disabled index (col)")) -> (element=w836:string)
        n461 = Index Array(array=w863, index (row)=3) -> (element=w861:string[])  [unwired: 1 in]
        n462 = call "Fill in Off Time.vi"("Start Time"=w836, "Data IN"=w840) -> ("Sample Rate"=w835:dbl, "Data OUT"=w839:sgl[][])  [unwired: 8 in]
        n463 = call "TimeDate String to Timestamp.vi"("Time/Date String"=w836) -> ("Timestamp"=w834:timestamp)  [unwired: 10 in]
        n464 = property on="Graph Channels" class="Clust (strict)"() -> ("Controls[]"=w857:refnum<vi>[])  [unwired: 2 in, 2 out]
        n465 = Delete From Array(array=w861, length=1, index=0) -> (array with subset deleted=w842:string[])  [unwired: 1 out]
        n466 = Array Size(array=w842) -> (size(s)=w841:i32)
        n467 = Array Size(array=w839) -> (size(s)=w854:i32[])
        n468 = for {
          tunnel: w857 -> [w890] mode=indexing
          tunnel: w842 -> [w887]
          tunnel: [w879] -> w858 mode=indexing
          tunnel: [w884] -> w843 mode=indexing
          tunnel: w841 -> [w877]
          i -> [w878]
          n469 = Greater Or Equal?(x=w878, y=w877) -> (x >= y?=w880:bool)
          n470 = Build Array (concatenate)("" ("element"), w887) -> (w886:string[])
          n471 = Increment(x=w878) -> (x+1=w883:i32)
          n472 = To More Specific Class(target class=refnum<vi> refnum ("Ring"), reference=w890) -> (specific class reference=w884:refnum<vi>)  [unwired: 1 in, 1 out]
          n473 = property class="Ring"(reference=w884, "Strings []"=w886) -> (reference out=w889:refnum<vi>)  [unwired: 1 in, 1 out]
          n474 = Select(t=0, s=w880, f=w883) -> (s? t:f=w882:i32)
          n475 = property class="Ring"(reference=w889, "Value"=w882) -> ()  [unwired: 1 in, 2 out]
          n476 = Not(x=w880) -> (.not. x?=w879:bool)
        }
        n477 = Index Array(array=w854) -> (element=w851:i32)  [unwired: 1 in]
        n478 = property on="Graph 1" class="WFGraph (strict)"("X Scale.Offset and Multiplier:Multiplier"=w835) -> ()  [unwired: 2 in, 2 out]
        n479 = property on="Graph 2" class="WFGraph (strict)"("X Scale.Offset and Multiplier:Multiplier"=w835) -> ()  [unwired: 2 in, 2 out]
        n480 = Reciprocal(x=w835) -> (1/x=w850:dbl)
        n481 = flat-sequence {
          tunnel: w851 -> [w873]
          tunnel: w839 -> [w874]
          tunnel: [w874] -> w853
          tunnel: [w873] -> w852
          tunnel: w853 -> [w875]
          tunnel: w852 -> [w876]
          frame #0 {
            n482 = call "Trim Data (by ref).vi"("Boolean"=TRUE) -> ()  [unwired: 12 in, 3 out]
          }
          frame #1 {
            n483 = call "Trim Data (by ref).vi"("length"=w876, "Array"=w875) -> ()  [unwired: 11 in, 3 out]
          }
        }
        n484 = Array To Cluster(array=w858) -> (cluster=w856:T33)
        n485 = local write "Graph Toggles"(w856) -> ()
        n486 = local write "Play"(FALSE ("Play")) -> ()
        n487 = local write "Pause"(TRUE ("Play")) -> ()
        n488 = call "Insert Multiple Events.vi"("Events to Insert"=string[] ["Update Graph Toggles", "Update Graph", "Update Graph", "Load Indicator Off"], "Event queue in"=w871) -> ("Event queue out"=w870:string[])  [unwired: 5 in]
        n489 = Bundle By Name(cluster=w867, "UnPause Once"=w847, "Pause Graph"=w847, "Buffer Size"=w851, "Force Update"=TRUE, "Start Timestamp"=w834, "Config.DAQ Settings.Sample Rate"=w850, "Graph Ch Refs"=w843) -> (w866:T28)
      }
      frame "Load Indicator Off" {
        n490 = property on="Decoration Tab" class="TabCtl (strict)"("DisabledEnum"=T30."Enabled" ("Disabled")) -> ()  [unwired: 2 in, 2 out]
        n491 = property on="Load Indicator Tab" class="TabCtl (strict)"("Visible"=FALSE) -> ()  [unwired: 2 in, 2 out]
      }
      frame "Connection Window" {
        n492 = Unbundle By Name(w909) -> ("App Config.Last Config (Std)"=w900:string, "App Config.Last Config (Def)"=w902:string, "App Config.Last Config (8TC)"=w895:string, "App Config.Support Dir (Local)"=w898:path, "Sys Cfg File Name"=w896:string)
        n493 = Build Path(base path=w898, name or relative path=w896) -> (appended path=w897:path)
        n494 = call "Initial Connection.vi"("Systems Config Path"=w897) -> ("Close Program"=w910:bool, "System Ref"=w906:tag, "Selected System"=w905:T14, "Error OUT"=w907:errorcluster)  [unwired: 14 in, 1 out]
        n495 = property on="Decoration Tab" class="TabCtl (strict)"(error in=w907, "DisabledEnum"=T30."Enabled" ("Disabled")) -> ()  [unwired: 1 in, 2 out]
        n496 = Unbundle By Name(w905) -> ("Description"=w904:string)
        n497 = case shown="\"Standard 8TC\"" w904 {
          tunnel: [System_Type."Standard" ("System Type") System_Type."Deformation" ("System Type") System_Type."Standard 8TC" ("System Type")] -> w903
          tunnel: [w916 w919 w921] -> w901
          tunnel: w902 -> [_ w919 _]
          tunnel: w900 -> [w916 _ _]
          tunnel: ["*.std" ("[pattern]") "*.def" ("[pattern]") "*.8TC" ("[pattern]")] -> w899
          tunnel: w895 -> [_ _ w921]
          frame "Standard", "Standard XT", Default {
          }
          frame "Deformation" {
          }
          frame "Standard 8TC" {
          }
        }
        n498 = case shown="True" w910 {
          tunnel: [string[] [] ("Events to Insert") string[] ["Exit"] ("Events to Insert")] -> w913
          frame False {
          }
          frame True {
          }
        }
        n499 = call "Insert Multiple Events.vi"("Events to Insert"=w913, "Event queue in"=w912) -> ("Event queue out"=w911:string[])  [unwired: 5 in]
        n500 = Bundle By Name(cluster=w909, "System Ref"=w906, "Selected System"=w905, "System Type"=w903, "Config Name"=w901, "Config Extension"=w899) -> (w914:T28)
      }
      frame "Update from Config" {
        w937 = T30."Disabled and Grayed Out" ("Disabled")
        w936 = T30."Enabled" ("Disabled")
        w938 = FALSE ("Trigger Armed")
        n501 = property on="Start Log" class="Bool"("Disabled"=w937) -> ()  [unwired: 2 in, 2 out]
        n502 = property on="Stop DAQ" class="Bool"("Disabled"=w937) -> ()  [unwired: 2 in, 2 out]
        n503 = property on="Arm DAQ" class="Bool"("Disabled"=w936) -> ()  [unwired: 2 in, 2 out]
        n504 = property on="Graph Channels" class="Clust (strict)"("DisabledEnum"=w936) -> ()  [unwired: 2 in, 2 out]
        n505 = property on="O-Scope Mode" class="Bool"("DisabledEnum"=w936) -> ()  [unwired: 2 in, 2 out]
        n506 = Unbundle By Name(w947) -> ("Calibration Path"=w940:path, "Config"=w927:T16)
        n507 = call "Read Sensor Scaling.vi"("Cal Base Path"=w940) -> ("Sensors scaling"=w941:T27)  [unwired: 14 in]
        n508 = Unbundle By Name(w927) -> ("DAQ Settings.Log Rate"=w929:dbl, "DAQ Settings.Rate Sec/Min (Log)"=w928:bool)
        n509 = call "Extract Channel Names and Addresses from Config.vi"("Config"=w927) -> ("Channel Names"=w934:string[], "Channel Addresses"=w945:string[])  [unwired: 13 in]
        n510 = Unbundle By Name(w927) -> ("DAQ Settings.Sample Rate"=w931:dbl, "DAQ Settings.Rate Sec/Min"=w932:bool)
        n511 = case shown="True" w932 {
          tunnel: w931 -> [w952 w955]
          tunnel: [w952 w953] -> w930
          frame False {
          }
          frame True {
            n512 = Divide(x=w955, y=60.0) -> (x/y=w953:dbl)
          }
        }
        n513 = case shown="True" w928 {
          tunnel: w929 -> [w948 w951]
          tunnel: [w948 w949] -> w926
          frame False {
          }
          frame True {
            n514 = Divide(x=w951, y=60.0) -> (x/y=w949:dbl)
          }
        }
        n515 = property on="Graph Channels" class="Clust (strict)"() -> ("Controls[]"=w933:refnum<vi>[])  [unwired: 2 in, 2 out]
        n516 = for {
          tunnel: w933 -> [w959] mode=indexing
          tunnel: w934 -> [w958]
          tunnel: [w957] -> w939 mode=indexing
          n517 = To More Specific Class(target class=refnum<vi> refnum ("Ring"), reference=w959) -> (specific class reference=w957:refnum<vi>)  [unwired: 1 in, 1 out]
          n518 = property class="Ring"(reference=w957, "Strings []"=w958) -> ()  [unwired: 1 in, 2 out]
        }
        n519 = Bundle By Name(cluster=w947, "Virtual Trigger"=w938, "Acquiring Data"=w938, "Trigger Armed"=w938, "Scaling"=w941, "Channel Addresses"=w945, "Trigger Index"=0, "Graph Ch Refs"=w939, "Config.DAQ Settings.Sample Rate (S/s)"=w930, "Config.DAQ Settings.Log Rate (S/s)"=w926) -> (w946:T28)
        n520 = call "Insert Multiple Events.vi"("Events to Insert"=string[] ["Build Channel Filter", "Disarm Trigger", "Clear Data", "Update Graph Settings"], "Event queue in"=w943) -> ("Event queue out"=w944:string[])  [unwired: 5 in]
      }
      frame "Build Channel Filter" {
        n521 = Unbundle By Name(w963) -> ("Config.Channels"=w961:T20[])  [unwired: 1 out]
        n522 = for {
          tunnel: w961 -> [w966] mode=indexing
          tunnel: [w965] -> w960 mode=indexing
          n523 = Unbundle By Name(w966) -> ("Acquire"=w965:bool)
        }
        n524 = Bundle By Name(cluster=w963, "Channel Filter"=w960) -> (w962:T28)
      }
      frame "Configure DAQ" {
        n525 = Unbundle By Name(w995) -> ("System Ref"=w967:tag, "Calibration Path"=w986:path, "Channel Filter"=w984:bool[], "Config"=w985:T16, "Scaling"=w993:T27, "System Type"=w969:T15, "O-Scope Mode"=w990:bool, "Config.DAQ Settings.Trigger Type"=w987:T10, "Total Channel Count"=w982:i16)
        n526 = call "Sort scaling sensors.vi"("Channels in"=w985, "Sensors (scale)"=w993) -> ("Sensor (scaling) out"=w983:T27)  [unwired: 17 in]
        n527 = flat-sequence {
          tunnel: w983 -> [w999]
          tunnel: w984 -> [w1000]
          tunnel: w985 -> [w1001]
          tunnel: w986 -> [w1002]
          tunnel: [w1002] -> w973
          tunnel: [w1001] -> w972
          tunnel: [w1000] -> w971
          tunnel: [w999] -> w970
          tunnel: [w996] -> w968
          tunnel: w967 -> [w996]
          tunnel: w982 -> [w1009]
          tunnel: [w1005] -> w978
          tunnel: [w1008] -> w976
          tunnel: [w1007] -> w975
          tunnel: [w1006] -> w974
          tunnel: w973 -> [w1013]
          tunnel: w972 -> [w1012]
          tunnel: w971 -> [w1011]
          tunnel: w970 -> [w1010]
          tunnel: w969 -> [w1004]
          tunnel: w968 -> [w1003]
          tunnel: [w1017] -> w979
          tunnel: [w1018] -> w980
          tunnel: [w1019] -> w981
          tunnel: w976 -> [w1019]
          tunnel: w975 -> [w1018]
          tunnel: w974 -> [w1017]
          frame #0 {
            w997 = 2
            n528 = property on="Decoration Tab" class="TabCtl (strict)"("DisabledEnum"=w997) -> ()  [unwired: 2 in, 2 out]
            n529 = property on="Graph 2" class="WFGraph (strict)"("DisabledEnum"=w997) -> ()  [unwired: 2 in, 2 out]
            n530 = property on="Connecting Tab" class="TabCtl (strict)"("Visible"=TRUE) -> ()  [unwired: 2 in, 2 out]
          }
          frame #1 {
            n531 = call "Configure DAQ (by ref).vi"("System Ref"=w1003, "Cal Files Path"=w1013, "Config"=w1012, "Channel Filter"=w1011, "Sensor (scaling)"=w1010, "Mode"=enum16{"Init", "Acquire", "Clear"}."Init", "System Type"=w1004, "Total Channel Count"=w1009) -> ("Input Task OUT"=w1008:refnum<k21>, "Ctr Task OUT"=w1007:refnum<k21>, "DI Task OUT"=w1006:refnum<k21>, "error out"=w1005:errorcluster)  [unwired: 12 in, 4 out]
          }
          frame #2 {
            w1015 = 0
            n532 = property on="Decoration Tab" class="TabCtl (strict)"("DisabledEnum"=w1015) -> ()  [unwired: 2 in, 2 out]
            n533 = property on="Connecting Tab" class="TabCtl (strict)"("Visible"=FALSE) -> ()  [unwired: 2 in, 2 out]
            n534 = property on="Graph 2" class="WFGraph (strict)"("DisabledEnum"=w1015) -> ()  [unwired: 2 in, 2 out]
          }
        }
        n535 = Tick Count (ms)() -> (millisecond timer value=w977:u32)
        n536 = Bundle By Name(cluster=w995, "Connected Timer"=w977, "Acquiring Data"=FALSE, "AI Task"=w981, "DO Task"=w980, "DI Task"=w979) -> (w992:T28)
        n537 = case shown="No Error" w978 {
          tunnel: w992 -> [w1027 w1036]
          tunnel: [w1026 w1035] -> w991
          tunnel: w990 -> [w1022 _]
          tunnel: [w1021 string[] ["Clear Trigger", "Disarm Trigger"] ("Events to Insert")] -> w989
          tunnel: w988 -> [w1021 _]
          tunnel: w987 -> [w1020 _]
          frame No Error {
            n538 = local write "Play"(TRUE ("Play")) -> ()
            n539 = local write "Pause"(FALSE ("Play")) -> ()
            n540 = case shown="False" w1022 {
              tunnel: w1020 -> [w1031 _]
              frame False {
                w1029 = T30."Enabled" ("Disabled")
                n541 = case shown="\"Manual\", \"Timed\"" w1031 {
                  tunnel: [T30."Disabled and Grayed Out" ("Disabled") T30."Enabled" ("Disabled")] -> w1030
                  frame Default {
                  }
                  frame "Manual", "Timed" {
                  }
                }
                n542 = property on="Add Data Point" class="Bool"("Disabled"=w1029) -> ()  [unwired: 2 in, 2 out]
                n543 = property on="Disarm DAQ" class="Bool"("Disabled"=w1029) -> ()  [unwired: 2 in, 2 out]
                n544 = property on="Start Log" class="Bool"("Disabled"=w1030) -> ()  [unwired: 2 in, 2 out]
              }
              frame True {
              }
            }
            n545 = Bundle By Name(cluster=w1027, "Pause Graph"=FALSE) -> (w1026:T28)
            n546 = property on="Arm DAQ" class="Bool"("Disabled"=T30."Disabled and Grayed Out") -> ()  [unwired: 2 in, 2 out]
          }
          frame Error {
            (unwired) string[] ["Clear Trigger", "Disarm Trigger", "Exit Mode"] ("Events to Insert")
            n547 = disable-structure shown="Disabled" {
              frame Disabled {
                n548 = One Button Dialog(message="Unable to connect to cDAQ.\n\nIf the cDAQ was just plugged in, it could tak up to 1 minute for Windows to establish an ethernet connection.") -> ()  [unwired: 1 in, 1 out]
              }
              frame Enabled {
              }
            }
            n549 = Bundle By Name(cluster=w1036, "Trigger Armed"=FALSE) -> (w1035:T28)
          }
        }
      }
      frame "DAQ" {
        n550 = Unbundle By Name(w1062) -> ("O-Scope Mode"=w1049:bool, "Acquire Data"=w1045:bool, "Virtual Trigger"=w1042:bool, "Add Data Point"=w1041:bool, "Config"=w1055:T16, "Channel Filter"=w1054:bool[], "System Type"=w1043:T15, "Time Offset"=w1053:dbl, "Graph Ch Refs"=w1060:refnum<vi>[], "Connected Timer"=w1050:u32)
        n551 = Or(x=w1042, y=w1041) -> (x .or. y?=w1040:bool)
        n552 = call "Configure DAQ (by ref).vi"("Config"=w1055, "Channel Filter"=w1054, "Manual/Timed Trigger"=w1045, "Mode"=enum16{"Init", "Acquire", "Clear"}."Acquire", "System Type"=w1043, "Time Offset"=w1053) -> ("Pretrigger Size"=w1052:i32, "Acquiring Data"=w1048:bool, "Data"=w1039:sgl[][], "error out"=w1044:errorcluster)  [unwired: 14 in, 4 out]
        n553 = Compound Arithmetic op=OR(w1048, w1049) -> (w1056:bool)
        n554 = And(x=w1048, y=w1040) -> (x .and. y?=w1047:bool)
        n555 = property on="Acquiring Tab" class="TabCtl (strict)"("Visible"=w1047) -> ()  [unwired: 2 in, 2 out]
        n556 = case shown="No Error" w1044 {
          tunnel: w1060 -> [w1073 _]
          tunnel: w1056 -> [w1067 _]
          tunnel: [w1069 string[] ["Clear Trigger", "Disarm Trigger"] ("Events to Insert")] -> w1059
          tunnel: w1040 -> [w1066 _]
          tunnel: [w1064 FALSE] -> w1046
          frame No Error {
            n557 = call "Realtime Data (by ref).vi"("Enum"=enum16{"Init", "Read", "Write"}."Read") -> ("New Data"=w1068:dbl[][])  [unwired: 1 in]
            n558 = case shown="True" w1066 {
              tunnel: [string[] ["Update Graph"] ("Events to Insert") string[] ["Midnight Check", "Segmented File Check", "Save Data"] ("Events to Insert")] -> w1069
              tunnel: [TRUE FALSE] -> w1064
              frame False {
              }
              frame True {
              }
            }
            n559 = Array Size(array=w1068) -> (size(s)=w1071:i32[])
            n560 = Index Array(array=w1071) -> (element #2=w1070:i32)  [unwired: 2 in, 1 out]
            n561 = Greater Than 0?(x=w1070) -> (x > 0?=w1065:bool)
            n562 = case shown="True" w1065 {
              tunnel: w1068 -> [_ w1081]
              tunnel: w1073 -> [_ w1082]
              frame False {
              }
              frame True {
                n563 = for {
                  tunnel: w1082 -> [w1089] mode=indexing
                  tunnel: w1081 -> [w1088]
                  tunnel: [w1087] -> w1078 mode=indexing
                  n564 = property class="Ring"(reference=w1089) -> ("Value"=w1086:variant)  [unwired: 1 in, 2 out]
                  n565 = Variant To Data(type=u16 0, Variant=w1086) -> (data=w1084:u16)  [unwired: 1 in, 1 out]
                  n566 = Index Array(array=w1088, index (row)=w1084) -> (element=w1083:dbl[])  [unwired: 1 in]
                  n567 = call-poly <vilib>:"Mean.vi"("X"=w1083) -> ("mean"=w1087:dbl)  [unwired: 1 out]
                }
                n568 = Array To Cluster(array=w1078) -> (cluster=→"Graph Numerics":T40)
                n569 = Array To Cluster(array=w1078) -> (cluster=→"Graph Numerics (Big)":T41)
              }
            }
            n570 = And(x=w1067, y=w1065) -> ()  [unwired: 1 out]
          }
          frame Error {
            (unwired) string[] ["Clear Trigger", "Disarm Trigger", "Exit Mode"] ("Events to Insert")
            n571 = One Button Dialog(message="Communication with cDAQ was interrupted.") -> ()  [unwired: 1 in, 1 out]
          }
        }
        n572 = call "Insert Multiple Events.vi"("Events to Insert"=w1059, "Event queue in"=w1058) -> ("Event queue out"=w1057:string[])  [unwired: 5 in]
        n573 = Bundle By Name(cluster=w1062, "Pretrigger Size"=w1052, "Data"=w1039, "Acquiring Data"=w1047, "Trigger Index"=0, "Connected Timer"=w1050, "Force Update"=w1046) -> (w1063:T28)
      }
      frame "Start Log" {
        w1107 = T30."Disabled" ("Disabled")
        w1100 = T30."Enabled" ("Disabled")
        n574 = Unbundle By Name(w1106) -> ("Start Timestamp"=w1099:timestamp, "Manual Data Mode"=w1095:bool, "Virtual Trigger"=w1094:bool, "Config.All Type Info"=w1110:T24, "Config.Channels"=w1109:T20[])
        n575 = feedback-in #1(w1095) -> ()
        n576 = feedback #1() -> (w1098:bool)  [unwired: 1 in]
        n577 = call "Find Non Part Signal Indexes.vi"("All Type Info"=w1110, "Channels"=w1109) -> ("Non Part Indexes (data)"=w1108:i32[])  [unwired: 11 in, 2 out]
        n578 = Greater?(x=w1095, y=w1098) -> (0:w1097:bool)
        n579 = Compound Arithmetic op=OR(w1097, invert w1094) -> (w1096:bool)
        n580 = case shown="True" w1096 {
          tunnel: [w1111 w1112] -> w1101
          tunnel: w1099 -> [w1111 _]
          frame False {
          }
          frame True {
            n581 = Get Date/Time In Seconds() -> (seconds since 1Jan1904=w1112:timestamp)
            "Start of Test:" <- w1112
          }
        }
        n582 = property on="Header Table:" class="Tbl (strict)"("DisabledEnum"=w1107) -> ()  [unwired: 2 in, 2 out]
        n583 = property on="Data Base Path:" class="Path"("DisabledEnum"=w1107) -> ()  [unwired: 2 in, 2 out]
        n584 = property on="Start of Test:" class="AbsTime (strict)"("DisabledEnum"=w1100) -> ()  [unwired: 2 in, 2 out]
        n585 = property on="Elapsed Time:" class="DigNum (strict)"("DisabledEnum"=w1100) -> ()  [unwired: 2 in, 2 out]
        n586 = property on="Samples Recorded:" class="DigNum (strict)"("DisabledEnum"=w1100) -> ()  [unwired: 2 in, 2 out]
        n587 = Bundle By Name(cluster=w1106, "Start Timestamp"=w1101, "Samples Acquired"=u32 0, "Data Log Indicies"=w1108) -> (w1105:T28)
        n588 = call "Insert Multiple Events.vi"("Events to Insert"=string[] ["Trigger DAQ"], "Event queue in"=w1104) -> ("Event queue out"=w1103:string[])  [unwired: 5 in]
      }
      frame "Stop DAQ" {
        w1117 = T30."Enabled" ("Disabled")
        n589 = Unbundle By Name(w1115) -> ("Log Path Ref"=w1114:refnum<file>)
        n590 = Close File(refnum=w1114) -> (error out=w1113:errorcluster)  [unwired: 1 in, 1 out]
        n591 = call <vilib>:"Clear Errors.vi"("error in (no error)"=w1113) -> ()  [unwired: 5 in, 2 out]
        n592 = property on="Header Table:" class="Tbl (strict)"("DisabledEnum"=w1117) -> ()  [unwired: 2 in, 2 out]
        n593 = property on="Data Base Path:" class="Path"("DisabledEnum"=w1117) -> ()  [unwired: 2 in, 2 out]
        n594 = call "Insert Multiple Events.vi"("Events to Insert"=string[] ["Cfg - Enable Tab", "Clear Trigger", "Disarm Trigger"], "Event queue in"=w1119) -> ("Event queue out"=w1118:string[])  [unwired: 5 in]
      }
      frame "Update Graph" {
        n595 = Unbundle By Name(w1150) -> ("O-Scope Mode"=w1130:bool, "Force Update"=w1136:bool, "Acquiring Data"=w1145:bool, "Data"=w1131:sgl[][], "Graph Ch Refs"=w1147:refnum<vi>[], "Config.DAQ Settings.Sample Rate (S/s)"=w1120:dbl, "Pause Graph"=w1143:bool, "Start Timestamp"=w1122:timestamp, "Buffer Size"=w1132:u32, "UnPause Once"=w1133:bool, "Pretrigger Size"=w1125:i32)
        n596 = To Double Precision Float(number=w1122) -> (double precision float=w1141:dbl)
        n597 = Empty Array?(array=w1131) -> (empty?=w1146:bool)
        n598 = call "Prep Data for Graph.vi"("Data"=w1131, "Graph Ch Refs"=w1147, "Pretrigger Size"=w1125, "Buffer Size"=w1132) -> ("Elements Deleted"=w1127:dbl, "Current Size"=w1126:dbl, "Data Out"=w1142:sgl[][])  [unwired: 9 in]
        n599 = Compound Arithmetic op=AND(invert w1146, w1145) -> (w1137:bool)
        n600 = Format Into String("Graph Range") -> (resulting string=w1139:string)  [unwired: 3 in, 1 out]
        n601 = Add(x=w1127, y=w1126) -> (x+y=w1128:dbl)
        n602 = Fract/Exp String To Number(string=w1139) -> (number=w1138:dbl)  [unwired: 3 in, 1 out]
        n603 = Compound Arithmetic op=OR(w1130, w1136, w1137) -> (w1124:bool)
        n604 = Reciprocal(x=w1120) -> (1/x=w1129:dbl)
        n605 = Compound Arithmetic op=AND(w1143, invert w1133) -> (w1134:bool)
        n606 = Divide(x=w1128, y=w1120) -> (x/y=w1121:dbl)
        n607 = Multiply(x=w1120, y=w1138) -> (x*y=w1144:dbl)
        n608 = case shown="True" w1124 {
          tunnel: w1142 -> [_ w1165]
          tunnel: w1144 -> [_ w1171]
          tunnel: w1134 -> [_ w1164]
          tunnel: w1120 -> [_ w1172]
          tunnel: w1141 -> [_ _]
          tunnel: w1138 -> [_ w1167]
          tunnel: w1127 -> [_ w1170]
          tunnel: w1126 -> [_ w1169]
          tunnel: w1129 -> [_ w1168]
          frame False {
          }
          frame True {
            n609 = Increment(x=w1171) -> (x+1=w1161:dbl)
            n610 = Divide(x=w1170, y=w1172) -> (x/y=w1163:dbl)
            n611 = Subtract(x=w1169, y=w1161) -> (x-y=w1162:dbl)
            n612 = Transpose 2D Array(2D array=w1165) -> (transposed array=w1155:sgl[][])
            n613 = Delete From Array(array=w1165, length=w1161, index (row)=w1162) -> (deleted portion=w1156:sgl[][])  [unwired: 1 in, 1 out]
            n614 = Transpose 2D Array(2D array=w1156) -> (transposed array=w1154:sgl[][])
            n615 = Add(x=0.0, y=w1163) -> (x+y=w1157:dbl)
            n616 = property on="Graph 2" class="WFGraph (strict)"("Value"=w1155, "XScale.Multiplier"=w1168, "XScale.Offset"=w1157, "XScale.Minimum"=w1157, "XScale.ScaleFit"=u8 1 ("X Scale.Scale Fit")) -> ("XScale.Maximum"=w1151:dbl)  [unwired: 2 in, 2 out]
            n617 = Subtract(x=w1151, y=w1157) -> (x-y=w1166:dbl)
            n618 = Max & Min(x=w1167, y=w1166) -> (min(x,y)=w1158:dbl)  [unwired: 1 out]
            n619 = Subtract(x=w1151, y=w1158) -> (x-y=w1159:dbl)
            n620 = case shown="False" w1164 {
              tunnel: w1154 -> [w1175 _]
              tunnel: w1159 -> [w1176 _]
              tunnel: [T30."Enabled" ("Disabled") T30."Disabled" ("Disabled")] -> w1160
              tunnel: w1168 -> [w1173 _]
              frame False {
                n621 = property on="Graph 1" class="WFGraph (strict)"("Value"=w1175, "XScale.Multiplier"=w1173, "XScale.Offset"=w1176, "XScale.Minimum"=w1176) -> ()  [unwired: 2 in, 2 out]
              }
              frame True {
              }
            }
            n622 = property on="Graph Range" class="Enum (strict)"("DisabledEnum"=w1160) -> ()  [unwired: 2 in, 2 out]
          }
        }
        n623 = Bundle By Name(cluster=w1150, "Time Offset"=w1121, "Data"=sgl[][] [], "Force Update"=w1133, "UnPause Once"=FALSE ("Force Update")) -> (w1149:T28)
      }
      frame "Update Graph Toggles" {
        n624 = property on="Graph Toggles" class="Clust (strict)"() -> ("Controls[]"=w1178:refnum<vi>[])  [unwired: 2 in, 2 out]
        n625 = for {
          tunnel: w1178 -> [w1185] mode=indexing
          i -> [w1182]
          n626 = To More Specific Class(target class=refnum<vi> refnum ("Boolean"), reference=w1185) -> (specific class reference=w1183:refnum<vi>)  [unwired: 1 in, 1 out]
          n627 = property class="Bool (strict)"(reference=w1183) -> ("Value"=w1181:bool)  [unwired: 1 in, 2 out]
          n628 = property on="Graph 1" class="WFGraph (strict)"("Active Plot"=w1182, "Plot.Visible?"=w1181) -> ()  [unwired: 2 in, 2 out]
          n629 = property on="Graph 2" class="WFGraph (strict)"("Active Plot"=w1182, "Plot.Visible?"=w1181) -> ()  [unwired: 2 in, 2 out]
        }
      }
      frame "Update Axis Toggles" {
        n630 = property on="Axis Toggles" class="Clust (strict)"() -> ("Controls[]"=w1186:refnum<vi>[])  [unwired: 2 in, 2 out]
        n631 = for {
          tunnel: w1186 -> [w1198] mode=indexing
          i -> [w1195]
          n632 = To More Specific Class(target class=refnum<vi> refnum ("Boolean"), reference=w1198) -> (specific class reference=w1196:refnum<vi>)  [unwired: 1 in, 1 out]
          n633 = property class="Bool (strict)"(reference=w1196) -> (reference out=w1193:refnum<vi>, "Value"=w1192:bool)  [unwired: 1 in, 1 out]
          n634 = Boolean To (0,1)(Boolean=w1192) -> (0, 1=w1194:i16)
          n635 = Select(t=u32 16711680, s=w1192, f=u32 16777226) -> (s? t:f=w1189:u32)
          n636 = property class="Bool (strict)"(reference=w1193, "BoolText.TextColor"=w1189) -> ()  [unwired: 1 in, 2 out]
          n637 = property on="Graph 1" class="WFGraph (strict)"("Active Plot"=w1195, "Plot.YScaleIdx"=w1194) -> ()  [unwired: 2 in, 2 out]
          n638 = property on="Graph 2" class="WFGraph (strict)"("Active Plot"=w1195, "Plot.YScaleIdx"=w1194) -> ()  [unwired: 2 in, 2 out]
        }
      }
      frame "Update Graph Settings" {
        n639 = Unbundle By Name(w1221) -> ("Config.Graph Settings"=w1217:T22)
        n640 = Unbundle(w1217) -> ("Graph Labels"=w1216:string[], w1215:u8[], w1214:i16[], w1213:u32[], w1212:u8[], w1211:u8[], w1210:u8[], w1209:u32[], w1208:u8[], w1207:u8[], w1206:u8[], w1205:dbl[], w1204:dbl[], "Graph Toggles"=w1202:bool[], "Axis Toggles"=w1201:bool[], "Graph Range"=w1200:T7)
        n641 = property on="Graph Channels" class="Clust (strict)"() -> ("Controls[]"=w1220:refnum<vi>[])  [unwired: 2 in, 2 out]
        n642 = Array To Cluster(array=w1202) -> (cluster=w1219:T42)
        n643 = Array To Cluster(array=w1201) -> (cluster=w1218:T43)
        n644 = for {
          N: 2 -> [_]
          tunnel: w1206 -> [w1224] mode=indexing
          tunnel: w1205 -> [w1227] mode=indexing
          tunnel: w1204 -> [w1226] mode=indexing
          i -> [w1225]
          n645 = property on="Graph 1" class="WFGraph (strict)"("ActYScl"=w1225, "YScale.ScaleFit"=w1224, "YScale.Maximum"=w1227, "YScale.Minimum"=w1226) -> ()  [unwired: 2 in, 2 out]
          n646 = property on="Graph 2" class="WFGraph (strict)"("ActYScl"=w1225, "YScale.ScaleFit"=w1224, "YScale.Maximum"=w1227, "YScale.Minimum"=w1226) -> ()  [unwired: 2 in, 2 out]
        }
        n647 = local write "Graph Toggles"(w1219) -> ()
        n648 = local write "Graph Range"(w1200) -> ()
        n649 = for {
          tunnel: w1220 -> [w1246] mode=indexing
          tunnel: w1216 -> [w1230] mode=indexing
          tunnel: w1215 -> [w1243] mode=indexing
          tunnel: w1214 -> [w1242] mode=indexing
          tunnel: w1213 -> [w1241] mode=indexing
          tunnel: w1212 -> [w1240] mode=indexing
          tunnel: w1211 -> [w1239] mode=indexing
          tunnel: w1210 -> [w1238] mode=indexing
          tunnel: w1209 -> [w1237] mode=indexing
          tunnel: w1208 -> [w1236] mode=indexing
          tunnel: w1207 -> [w1235] mode=indexing
          i -> [w1234]
          n650 = To More Specific Class(target class=refnum<vi> refnum ("Ring"), reference=w1246) -> (specific class reference=w1245:refnum<vi>)  [unwired: 1 in, 1 out]
          n651 = property on="Graph 1" class="WFGraph (strict)"("Active Plot"=w1234, "Plot.Bar Plot Style"=w1243, "Plot.Fill To"=w1242, "Plot.Fill/Pt. Color"=w1241, "Plot.Label Style"=w1240, "Plot.Line Style"=w1239, "Plot.Line Width"=w1238, "Plot.Plot Color"=w1237, "Plot.Plot Interpolation"=w1236, "Plot.Point Style"=w1235) -> ()  [unwired: 2 in, 2 out]
          n652 = property class="Ring"(reference=w1245) -> (reference out=w1244:refnum<vi>, "Strings []"=w1229:string[])  [unwired: 1 in, 1 out]
          n653 = property on="Graph 2" class="WFGraph (strict)"("Active Plot"=w1234, "Plot.Bar Plot Style"=w1243, "Plot.Fill To"=w1242, "Plot.Fill/Pt. Color"=w1241, "Plot.Label Style"=w1240, "Plot.Line Style"=w1239, "Plot.Line Width"=w1238, "Plot.Plot Color"=w1237, "Plot.Plot Interpolation"=w1236, "Plot.Point Style"=w1235) -> ()  [unwired: 2 in, 2 out]
          n654 = Search 1D Array(1D array=w1229, element=w1230) -> (index of element=w1228:i32)  [unwired: 1 in]
          n655 = Less Than 0?(x=w1228) -> (x < 0?=w1233:bool)
          n656 = Select(t=0, s=w1233, f=w1228) -> (s? t:f=w1231:i32)
          n657 = property class="Ring"(reference=w1244, "Value"=w1231) -> ()  [unwired: 1 in, 2 out]
        }
        n658 = local write "Axis Toggles"(w1218) -> ()
        n659 = call "Insert Multiple Events.vi"("Events to Insert"=string[] ["Update Graph Toggles", "Update Axis Toggles"], "Event queue in"=w1203) -> ("Event queue out"=w1222:string[])  [unwired: 5 in]
      }
      frame "Midnight Check" {
        n660 = Unbundle By Name(w1253) -> ("Config.DAQ Settings.Save Mode"=w1248:T8, "Midnight Check"=w1251:timestamp, "File Created?"=w1249:bool)
        n661 = case shown="\"New File at Midnight\"" w1248 {
          tunnel: w1253 -> [w1254 w1265]
          tunnel: [w1254 w1264] -> w1252
          tunnel: w1251 -> [_ w1259]
          tunnel: w1249 -> [_ w1256]
          frame Default {
          }
          frame "New File at Midnight" {
            n662 = Get Date/Time In Seconds() -> (seconds since 1Jan1904=w1258:timestamp)
            n663 = Seconds To Date/Time(time stamp (now)=w1258) -> (date time rec=w1263:T44)  [unwired: 1 in]
            n664 = Seconds To Date/Time(time stamp (now)=w1259) -> (date time rec=w1262:T44)  [unwired: 1 in]
            n665 = Unbundle By Name(w1263) -> ("hour"=w1261:i32)
            n666 = Unbundle By Name(w1262) -> ("hour"=w1260:i32)
            n667 = Less?(x=w1261, y=w1260) -> (x < y?=w1255:bool)
            n668 = case shown="True" w1255 {
              tunnel: [w1266 FALSE] -> w1257
              tunnel: w1256 -> [w1266 _]
              frame False {
              }
              frame True {
              }
            }
            n669 = Bundle By Name(cluster=w1265, "Midnight Check"=w1258, "File Created?"=w1257, "Midnight Rollover"=w1255) -> (w1264:T28)
          }
        }
      }
      frame "Segmented File Check" {
        n670 = Unbundle By Name(w1274) -> ("Config.DAQ Settings.Save Mode"=w1269:T8, "Saving Path"=w1272:path, "Config.DAQ Settings.File Size Limit"=w1268:dbl, "File Created?"=w1270:bool)
        n671 = case shown="\"Segmented Files\"" w1269 {
          tunnel: w1274 -> [w1275 w1287]
          tunnel: [w1275 w1286] -> w1273
          tunnel: w1272 -> [_ w1282]
          tunnel: w1270 -> [_ w1284]
          tunnel: w1268 -> [_ w1279]
          frame Default {
          }
          frame "Segmented Files" {
            n672 = Get File Size(file=w1282) -> (size (in bytes)=w1278:i64)  [unwired: 1 in, 2 out]
            n673 = Divide(x=w1278, y=i64 1000000) -> (x/y=w1277:dbl)
            n674 = Greater Or Equal?(x=w1277, y=w1279) -> (x >= y?=w1283:bool)
            n675 = case shown="True" w1283 {
              tunnel: [w1290 FALSE] -> w1285
              tunnel: w1284 -> [w1290 _]
              tunnel: w1282 -> [w1288 w1298]
              tunnel: [FALSE TRUE] -> w1281
              tunnel: [w1288 w1292] -> w1280
              frame False {
              }
              frame True {
                n676 = Strip Path(path=w1298) -> (stripped path=w1293:path, name=w1295:string)
                n677 = Match Pattern(string=w1295, regular expression="(") -> (before substring=w1291:string, after substring=w1294:string, offset past match=w1296:i32)  [unwired: 1 in, 1 out]
                n678 = case shown="-1" w1296 {
                  tunnel: w1295 -> [_ w1316]
                  tunnel: w1294 -> [w1302 _]
                  tunnel: w1293 -> [w1306 w1313]
                  tunnel: [w1305 w1311] -> w1292
                  tunnel: w1291 -> [w1308 _]
                  frame 0, Default {
                    n679 = Match Pattern(string=w1302, regular expression=")") -> (before substring=w1301:string)  [unwired: 1 in, 3 out]
                    n680 = Decimal String To Number(string=w1301) -> (number=w1310:i32)  [unwired: 2 in, 1 out]
                    n681 = Increment(x=w1310) -> (x+1=w1307:i32)
                    n682 = Format Into String(format string="(%d).csv", initial string=w1308, w1307) -> (resulting string=w1304:string)  [unwired: 1 in, 1 out]
                    n683 = Build Path(base path=w1306, name or relative path=w1304) -> (appended path=w1305:path)
                  }
                  frame -1 {
                    n684 = Search and Replace String(input string=w1316, search string=".csv", replace string=" (2).csv" ("search string")) -> (result string=w1312:string)  [unwired: 5 in, 3 out]
                    n685 = Build Path(base path=w1313, name or relative path=w1312) -> (appended path=w1311:path)
                  }
                }
              }
            }
            n686 = Bundle By Name(cluster=w1287, "File Created?"=w1285, "Saving Path"=w1280, "Segment File"=w1281) -> (w1286:T28)
          }
        }
      }
      frame "Save Data" {
        # "Do Not Insert if CPU Saver is True"
        n687 = Unbundle By Name(w1360) -> ("Add Data Point"=w1325:bool, "Manual Data Mode"=w1320:bool, "Title Bar"=w1338:refnum<vi>, "Segment File"=w1345:bool, "Config"=w1358:T16, "Saving Path"=w1354:path, "Data"=w1355:sgl[][], "Acquiring Data"=w1352:bool, "Start Timestamp"=w1332:timestamp, "File Created?"=w1353:bool, "O-Scope Mode"=w1350:bool, "Samples Acquired"=w1349:u32, "Data Log Indicies"=w1330:i32[], "Pretrigger Size"=w1348:i32, "Midnight Check"=w1343:timestamp, "Midnight Rollover"=w1344:bool, "Config.Data Base Path"=w1336:path, "Samples Recorded"=w1334:u32, "Log Path Ref"=w1317:refnum<file>, "Virtual Trigger"=w1341:bool)
        n688 = Get Date/Time In Seconds() -> (seconds since 1Jan1904=w1335:timestamp)
        n689 = property on="Save Data As" class="Bool"("DisabledEnum"=T30."Enabled" ("Disabled")) -> ()  [unwired: 2 in, 2 out]
        n690 = Subtract(x=w1335, y=w1332) -> (x-y=w1323:dbl)
        n691 = case shown="False" w1350 {
          tunnel: w1358 -> [w1390 _]
          tunnel: [w1389 w1525] -> w1357
          tunnel: [w1388 w1524] -> w1356
          tunnel: w1355 -> [w1387 _]
          tunnel: w1332 -> [w1386 _]
          tunnel: w1354 -> [w1385 w1525]
          tunnel: w1353 -> [w1384 w1524]
          tunnel: w1352 -> [w1383 _]
          tunnel: w1349 -> [w1382 w1521]
          tunnel: w1348 -> [w1381 _]
          tunnel: [w1380 string[] [] ("event queue out")] -> w1346
          tunnel: w1345 -> [w1379 _]
          tunnel: w1344 -> [w1378 _]
          tunnel: w1343 -> [w1377 _]
          tunnel: w1338 -> [w1376 _]
          tunnel: w1336 -> [w1375 _]
          tunnel: w1334 -> [w1374 w1522]
          tunnel: [w1373 w1522] -> w1333
          tunnel: [w1372 w1521] -> w1331
          tunnel: w1330 -> [w1371 _]
          tunnel: [w1370 FALSE ("Stop DAQ")] -> w1326
          tunnel: w1325 -> [w1369 _]
          tunnel: [w1368 FALSE ("Add Data Point")] -> w1324
          tunnel: w1320 -> [w1367 _]
          tunnel: w1323 -> [_ _]
          tunnel: [w1366 FALSE ("empty?")] -> w1322
          tunnel: [w1365 w1517] -> w1318
          tunnel: w1317 -> [w1364 w1517]
          frame False {
            # "NOT O-Scope Mode"
            n692 = case shown="True" w1384 {
              selector: w1384 -> [_ w1440]
              tunnel: w1390 -> [w1412 w1433]
              tunnel: [w1410 w1438] -> w1389
              tunnel: [TRUE ("append to file? (new file:F)") w1437] -> w1388
              tunnel: w1387 -> [w1409 w1442]
              tunnel: w1386 -> [w1402 w1441]
              tunnel: w1385 -> [w1406 w1443]
              tunnel: w1383 -> [_ w1439]
              tunnel: w1382 -> [w1399 w1436]
              tunnel: w1381 -> [_ w1435]
              tunnel: [w1407 string[] [] ("event queue out")] -> w1380
              tunnel: w1379 -> [w1405 _]
              tunnel: w1378 -> [w1404 _]
              tunnel: w1377 -> [w1403 _]
              tunnel: w1376 -> [_ _]
              tunnel: w1375 -> [w1395 _]
              tunnel: w1374 -> [w1400 w1432]
              tunnel: [w1400 w1431] -> w1373
              tunnel: [w1399 w1430] -> w1372
              tunnel: w1371 -> [_ w1429]
              tunnel: [FALSE ("Stop DAQ") w1428] -> w1370
              tunnel: w1369 -> [w1397 w1427]
              tunnel: [w1397 w1426] -> w1368
              tunnel: w1367 -> [_ w1425]
              tunnel: [FALSE ("empty?") w1424] -> w1366
              tunnel: [w1394 w1422] -> w1365
              tunnel: w1364 -> [w1393 w1423]
              frame False {
                # "File Not Created"
                n693 = Close File(refnum=w1393) -> (error out=w1392:errorcluster)  [unwired: 1 in, 1 out]
                n694 = Empty Array?(array=w1409) -> (empty?=w1408:bool)
                n695 = call <vilib>:"Clear Errors.vi"("error in (no error)"=w1392) -> ("error out"=w1391:errorcluster)  [unwired: 5 in, 1 out]
                n696 = Select(t=w1403, s=w1404, f=w1402) -> (s? t:f=w1401:timestamp)
                n697 = case shown="True" w1408 {
                  tunnel: [string[] ["Save Data"] ("event queue out") string[] [] ("event queue out")] -> w1407
                  frame False {
                  }
                  frame True {
                  }
                }
                n698 = flat-sequence {
                  tunnel: w1412 -> [w1419]
                  tunnel: [w1418] -> w1410
                  tunnel: w1406 -> [w1417]
                  tunnel: w1405 -> [w1416]
                  tunnel: w1401 -> [w1415]
                  tunnel: w1395 -> [w1414]
                  tunnel: [w1413] -> w1394
                  tunnel: w1391 -> [_]
                  frame #0 {
                    n699 = call "Generate New Data File.vi"("Config"=w1419, "Segment File"=w1416, "Saving Path"=w1417, "Start Time"=w1415, "Base Path"=w1414) -> ("new file path (Not A Path if cancelled)"=w1418:path, "Log Path Ref"=w1413:refnum<file>)  [unwired: 9 in]
                  }
                }
              }
              frame True {
                # "File Created"
                n700 = case shown="True" w1439 {
                  tunnel: [w1451 w1468] -> w1438
                  tunnel: [w1450 w1466] -> w1437
                  tunnel: w1442 -> [_ w1465]
                  tunnel: w1441 -> [_ w1467]
                  tunnel: w1443 -> [w1451 w1468]
                  tunnel: w1440 -> [w1450 w1466]
                  tunnel: w1436 -> [w1448 w1464]
                  tunnel: w1435 -> [_ w1463]
                  tunnel: w1433 -> [_ w1462]
                  tunnel: w1432 -> [w1449 w1461]
                  tunnel: [w1449 w1460] -> w1431
                  tunnel: [w1448 w1459] -> w1430
                  tunnel: w1429 -> [_ w1458]
                  tunnel: [FALSE ("Stop DAQ") w1457] -> w1428
                  tunnel: w1427 -> [_ w1456]
                  tunnel: [FALSE w1455] -> w1426
                  tunnel: w1425 -> [_ w1454]
                  tunnel: [FALSE ("empty?") w1453] -> w1424
                  tunnel: w1423 -> [w1444 w1452]
                  tunnel: [w1444 w1452] -> w1422
                  frame False {
                    # "NOT Acquiring Data"
                  }
                  frame True {
                    # "Acquiring Data"
                    n701 = Empty Array?(array=w1465) -> (empty?=w1453:bool)
                    n702 = case shown="False" w1453 {
                      tunnel: w1465 -> [w1479 _]
                      tunnel: w1468 -> [_ _]
                      tunnel: w1467 -> [w1486 _]
                      tunnel: w1464 -> [w1482 w1515]
                      tunnel: w1463 -> [w1485 _]
                      tunnel: w1462 -> [w1484 _]
                      tunnel: w1461 -> [w1483 w1516]
                      tunnel: [w1477 w1516] -> w1460
                      tunnel: [w1476 w1515] -> w1459
                      tunnel: w1458 -> [w1478 _]
                      tunnel: [w1475 FALSE ("Stop DAQ")] -> w1457
                      tunnel: w1456 -> [w1473 w1513]
                      tunnel: [FALSE ("Add Data Point") w1513] -> w1455
                      tunnel: w1454 -> [w1470 _]
                      tunnel: w1452 -> [w1469 _]
                      frame False {
                        # "Data NOT Empty"
                        n703 = case shown="False" w1470 {
                          tunnel: w1486 -> [w1497 _]
                          tunnel: w1485 -> [w1496 _]
                          tunnel: w1484 -> [w1495 _]
                          tunnel: w1483 -> [w1494 w1500]
                          tunnel: w1482 -> [w1493 w1498]
                          tunnel: [w1492 w1500] -> w1480
                          tunnel: w1479 -> [w1491 _]
                          tunnel: w1478 -> [w1490 _]
                          tunnel: [w1489 w1498] -> w1474
                          tunnel: [w1488 FALSE ("Stop DAQ")] -> w1472
                          tunnel: w1469 -> [w1487 _]
                          frame False {
                            n704 = call "Auto Save Trigger Data.vi"("Samples Recorded"=w1494, "Data Log Indicies"=w1490, "Log Path Ref"=w1487, "Config"=w1495, "Data"=w1491, "Start Time"=w1497, "Samples Acquired"=w1493, "Pretrigger Size"=w1496) -> ("Samples Recorded OUT"=w1492:u32, "Stop DAQ"=w1488:bool, "Samples Acquired OUT"=w1489:u32)  [unwired: 9 in]
                          }
                          frame True {
                          }
                        }
                        n705 = Compound Arithmetic op=AND(w1473, invert w1472) -> (w1471:bool)
                        n706 = case shown="True" w1471 {
                          tunnel: w1480 -> [w1503 w1512]
                          tunnel: w1479 -> [_ w1511]
                          tunnel: w1478 -> [_ w1510]
                          tunnel: w1469 -> [_ w1504]
                          tunnel: [w1503 w1509] -> w1477
                          tunnel: [w1502 w1508] -> w1476
                          tunnel: [w1501 w1507] -> w1475
                          tunnel: w1474 -> [w1502 w1506]
                          tunnel: w1472 -> [w1501 _]
                          frame False {
                          }
                          frame True {
                            n707 = call "Auto Save Trigger Data.vi"("Samples Recorded"=w1512, "Data Log Indicies"=w1510, "Log Path Ref"=w1504, "Data"=w1511, "Add Data Point"=TRUE, "Samples Acquired"=w1506) -> ("Samples Recorded OUT"=w1509:u32, "Stop DAQ"=w1507:bool, "Samples Acquired OUT"=w1508:u32)  [unwired: 11 in]
                          }
                        }
                      }
                      frame True {
                        # "Data Empty"
                      }
                    }
                  }
                }
              }
            }
          }
          frame True {
            # "O-Scope Mode"
          }
        }
        n708 = Not(x=w1341) -> (.not. x?=w1340:bool)
        n709 = Build Array(w1340) -> (w1342:bool[])
        n710 = call "Insert Multiple Events.vi"("Insert all? (T)"=TRUE, "Insert Selected?"=w1342, "Events to Insert"=string[] ["Update Graph"] ("event queue out"), "Event queue in"=w1337) -> ("Event queue out"=w1347:string[])  [unwired: 3 in]
        n711 = call "Insert Multiple Events.vi"("Events to Insert"=w1346, "Event queue in"=w1347) -> ("Event queue out"=w1329:string[])  [unwired: 5 in]
        n712 = Not(x=w1322) -> (.not. x?=w1321:bool)
        n713 = Compound Arithmetic op=OR(w1321, invert w1320) -> (w1319:bool)
        n714 = case shown="True" w1319 {
          tunnel: w1333 -> [_ w1363]
          tunnel: w1323 -> [_ w1362]
          frame False {
          }
          frame True {
            "Samples Recorded:" <- w1363
            "Elapsed Time:" <- w1362
          }
        }
        n715 = Bundle By Name(cluster=w1360, "Samples Recorded"=w1333, "Samples Acquired"=w1331, "Saving Path"=w1357, "Log Path Ref"=w1318, "File Created?"=w1356, "Add Data Point"=w1324) -> (w1359:T28)
        n716 = call "Insert Multiple Events.vi"("Insert all? (T)"=w1326, "Events to Insert"=string[] ["Stop DAQ"] ("event queue out"), "Event queue in"=w1329) -> ("Event queue out"=w1328:string[])  [unwired: 4 in]
      }
      frame "Save Graph Settings" {
        n717 = property on="Graph Channels" class="Clust (strict)"() -> ("Controls[]"=w1552:refnum<vi>[])  [unwired: 2 in, 2 out]
        n718 = for {
          tunnel: w1552 -> [w1568] mode=indexing
          tunnel: [w1567] -> w1549 mode=indexing
          tunnel: [w1565] -> w1548 mode=indexing
          tunnel: [w1564] -> w1547 mode=indexing
          tunnel: [w1563] -> w1546 mode=indexing
          tunnel: [w1562] -> w1545 mode=indexing
          tunnel: [w1561] -> w1544 mode=indexing
          tunnel: [w1560] -> w1543 mode=indexing
          tunnel: [w1559] -> w1542 mode=indexing
          tunnel: [w1558] -> w1541 mode=indexing
          tunnel: [w1557] -> w1540 mode=indexing
          i -> [w1566]
          n719 = To More Specific Class(target class=refnum<vi> refnum ("Ring"), reference=w1568) -> (specific class reference=w1570:refnum<vi>)  [unwired: 1 in, 1 out]
          n720 = property on="Graph 1" class="WFGraph (strict)"("Active Plot"=w1566) -> ("Plot.Bar Plot Style"=w1565:u8, "Plot.Fill To"=w1564:i16, "Plot.Fill/Pt. Color"=w1563:u32, "Plot.Label Style"=w1562:u8, "Plot.Line Style"=w1561:u8, "Plot.Line Width"=w1560:u8, "Plot.Plot Color"=w1559:u32, "Plot.Plot Interpolation"=w1558:u8, "Plot.Point Style"=w1557:u8)  [unwired: 2 in, 2 out]
          n721 = property class="Ring"(reference=w1570) -> ("RingText.Text"=w1567:string)  [unwired: 1 in, 2 out]
        }
        n722 = for {
          N: 2 -> [_]
          tunnel: [w1555] -> w1538 mode=indexing
          tunnel: [w1554] -> w1537 mode=indexing
          tunnel: [w1553] -> w1536 mode=indexing
          i -> [w1556]
          n723 = property on="Graph 1" class="WFGraph (strict)"("ActYScl"=w1556) -> ("YScale.ScaleFit"=w1555:u8, "YScale.Maximum"=w1554:dbl, "YScale.Minimum"=w1553:dbl)  [unwired: 2 in, 2 out]
        }
        n724 = local read "Graph Toggles"() -> (w1551:T4)
        n725 = local read "Graph Range"() -> (w1533:T7)
        n726 = local read "Axis Toggles"() -> (w1550:T4)
        n727 = Cluster To Array(cluster=w1551) -> (array=w1535:bool[])
        n728 = Cluster To Array(cluster=w1550) -> (array=w1534:bool[])
        n729 = Bundle(cluster=T22 {"Graph Labels"=[], [], [], [], [], [], [], [], [], [], [], [], [], "Graph Toggles"=[], "Axis Toggles"=[], "Graph Range"=enum."1"} ("output cluster"), "Graph Labels"=w1549, w1548, w1547, w1546, w1545, w1544, w1543, w1542, w1541, w1540, w1538, w1537, w1536, "Graph Toggles"=w1535, "Axis Toggles"=w1534, "Graph Range"=w1533) -> (w1529:T22)
        n730 = Bundle By Name(cluster=w1531, "Config.Graph Settings"=w1529) -> (w1530:T28)
        n731 = call "Insert Multiple Events.vi"("Events to Insert"=string[] ["Cfg - Save"], "Event queue in"=w1526) -> ("Event queue out"=w1527:string[])  [unwired: 5 in]
      }
      frame "Arm Trigger" {
        n732 = Unbundle By Name(w1573) -> ("O-Scope Mode"=w1572:bool)
        n733 = Not(x=w1572) -> (.not. x?=w1571:bool)
        n734 = call "Trim Data (by ref).vi"("Boolean"=TRUE) -> ()  [unwired: 12 in, 3 out]
        n735 = Bundle By Name(cluster=w1573, "Trigger Armed"=w1571, "Buffer Size"=u32 100000, "File Created?"=FALSE, "Time Offset"=0.0) -> (w1578:T28)
      }
      frame "Disarm Trigger" {
        w1580 = T30."Disabled and Grayed Out" ("Disabled")
        w1581 = FALSE ("Trigger Armed")
        n736 = property on="Open File" class="Bool"("DisabledEnum"=T30."Enabled" ("Disabled")) -> ()  [unwired: 2 in, 2 out]
        n737 = property on="O-Scope Mode" class="Bool"("DisabledEnum"=T30."Enabled" ("Disabled")) -> ()  [unwired: 2 in, 2 out]
        n738 = property on="Arm DAQ" class="Bool"("Disabled"=T30."Enabled") -> ()  [unwired: 2 in, 2 out]
        n739 = property on="Start Log" class="Bool"("Disabled"=w1580) -> ()  [unwired: 2 in, 2 out]
        n740 = property on="Disarm DAQ" class="Bool"("Disabled"=w1580) -> ()  [unwired: 2 in, 2 out]
        n741 = property on="Add Data Point" class="Bool"("Disabled"=w1580) -> ()  [unwired: 2 in, 2 out]
        n742 = call "Configure DAQ (by ref).vi"("Mode"=enum16{"Init", "Acquire", "Clear"}."Clear") -> ()  [unwired: 19 in, 8 out]
        n743 = Bundle By Name(cluster=w1583, "Trigger Armed"=w1581, "Acquire Data"=w1581, "Acquiring Data"=w1581) -> (w1587:T28)
      }
      frame "Start DAQ" {
        n744 = Unbundle By Name(w1589) -> ("AI Task"=w1593:refnum<k21>)
        n745 = call <vilib>:"DAQmx Start Task.vi"("task/channels in"=w1593) -> ("task out"=w1592:refnum<k21>)  [unwired: 13 in, 1 out]
        n746 = disable-structure shown="Disabled" {
          frame Disabled {
            n747 = while {
              stop <- w1595 stop-if-true
              n748 = call "AI RT FIFO (by ref).vi"("Mode"=RT_FIFO_Mode."Read") -> ("Empty?"=w1595:bool)  [unwired: 11 in, 3 out]
            }
          }
          frame Enabled {
          }
        }
        n749 = property class="DAQmx Read"(reference=w1592) -> (reference out=w1591:refnum<k21>, "AvailSampPerChan"=w1590:u32)  [unwired: 1 in, 1 out]
        n750 = call-poly <vilib>:"DAQmx Read.vi"("task/channels in"=w1591, "number of samples per channel"=w1590) -> ()  [unwired: 11 in, 3 out]
      }
      frame "Trigger DAQ" {
        n751 = Unbundle By Name(w1608) -> ("Manual Data Mode"=w1597:bool, "Trigger Armed"=w1599:bool, "Config.DAQ Settings.Sample Rate (S/s)"=w1602:dbl, "Config.DAQ Settings.Trigger Type"=w1601:T10, "Start Timestamp"=w1600:timestamp)
        n752 = Or(x=w1597, y=w1599) -> (x .or. y?=w1598:bool)
        n753 = case shown="True" w1598 {
          tunnel: [FALSE w1610] -> w1606
          tunnel: w1602 -> [_ w1617]
          tunnel: w1601 -> [_ w1614]
          tunnel: w1600 -> [_ w1613]
          tunnel: w1597 -> [_ w1611]
          frame False {
          }
          frame True {
            w1616 = T30."Enabled" ("Disabled")
            n754 = case shown="\"Manual\", \"Timed\"" w1614 {
              tunnel: [T30."Disabled and Grayed Out" ("Disabled") T30."Enabled" ("Disabled")] -> w1615
              tunnel: [T30."Enabled" ("Disabled") T30."Disabled and Grayed Out" ("Disabled")] -> w1612
              frame Default {
              }
              frame "Manual", "Timed" {
              }
            }
            n755 = disable-structure shown="Disabled" {
              disable-tunnel: w1617 -> [w1626 _]
              disable-tunnel: w1613 -> [w1623 _]
              frame Disabled {
                n756 = Reciprocal(x=w1626) -> (1/x=w1624:dbl)
                n757 = To Double Precision Float(number=w1623) -> (double precision float=w1625:dbl)
                n758 = property on="Graph 1" class="WFGraph (strict)"("X Scale.Offset and Multiplier:Multiplier"=w1624) -> ()  [unwired: 2 in, 2 out]
                n759 = property on="Graph 2" class="WFGraph (strict)"("X Scale.Offset and Multiplier:Multiplier"=w1624) -> ()  [unwired: 2 in, 2 out]
                n760 = property on="Graph 1" class="WFGraph (strict)"("XScale.Offset"=w1625) -> ()  [unwired: 2 in, 2 out]
                n761 = property on="Graph 2" class="WFGraph (strict)"("XScale.Offset"=w1625) -> ()  [unwired: 2 in, 2 out]
              }
              frame Enabled {
              }
            }
            n762 = Not(x=w1611) -> (.not. x?=w1610:bool)
            n763 = property on="Start Log" class="Bool"("Disabled"=T30."Disabled and Grayed Out") -> ()  [unwired: 2 in, 2 out]
            n764 = property on="Play" class="Bool (strict)"("DisabledEnum"=w1616) -> ()  [unwired: 2 in, 2 out]
            n765 = property on="Pause" class="Bool (strict)"("DisabledEnum"=w1616) -> ()  [unwired: 2 in, 2 out]
            n766 = property on="Disarm DAQ" class="Bool"("Disabled"=w1612) -> ()  [unwired: 2 in, 2 out]
            n767 = property on="Stop DAQ" class="Bool"("Disabled"=w1615) -> ()  [unwired: 2 in, 2 out]
          }
        }
        n768 = call "Insert Multiple Events.vi"("Insert all? (T)"=w1597, "Events to Insert"=string[] ["Save Data"], "Event queue in"=w1604) -> ("Event queue out"=w1605:string[])  [unwired: 4 in]
        n769 = Bundle By Name(cluster=w1608, "Virtual Trigger"=w1606) -> (w1607:T28)
      }
      frame "Clear Trigger" {
        w1628 = T30."Enabled" ("Disabled")
        w1627 = FALSE ("Acquiring Data")
        n770 = property on="Disarm DAQ" class="Bool"("Disabled"=w1628) -> ()  [unwired: 2 in, 2 out]
        n771 = property on="Start Log" class="Bool"("Disabled"=w1628) -> ()  [unwired: 2 in, 2 out]
        n772 = property on="Add Data Point" class="Bool"("Disabled"=w1628) -> ()  [unwired: 2 in, 2 out]
        n773 = property on="Stop DAQ" class="Bool"("Disabled"=T30."Disabled and Grayed Out") -> ()  [unwired: 2 in, 2 out]
        n774 = Bundle By Name(cluster=w1631, "Virtual Trigger"=w1627, "Manual Data Mode"=w1627) -> (w1630:T28)
      }
      frame "Clear Data" {
        n775 = Bundle By Name(cluster=w1636, "Data"=sgl[][] [], "Trigger Index"=0) -> (w1637:T28)
      }
      frame "Error" {
      }
      frame "File Open Error" {
        n776 = One Button Dialog(message="Unable to Log Data. File already open.\nPLEASE CLOSE THE FILE.") -> ()  [unwired: 1 in, 1 out]
        n777 = call "Insert Multiple Events.vi"("Events to Insert"=string[] ["Clear Trigger", "Disarm Trigger", "DAQ"], "Event queue in"=w1642) -> ("Event queue out"=w1640:string[])  [unwired: 5 in]
      }
      frame "Exit" {
        # "Only Close App if It is an Executable"
        n778 = disable-structure shown="Disabled" {
          disable-tunnel: w1645 -> [w1649 _]
          frame Disabled {
            n779 = Unbundle By Name(w1649) -> ("Calibration Path"=w1648:path, "Sensors"=w1650:T26[])
            n780 = Flatten To String(anything=w1650) -> (data string=w1651:string)  [unwired: 3 in, 2 out]
            n781 = call "Write Characters To File with Advisory Dialog Option and Error Out.vi"("file path (dialog if empty)"=w1648, "character string"=w1651, "advisory dialog? (display:T)"=FALSE) -> ()  [unwired: 11 in, 2 out]
          }
          frame Enabled {
          }
        }
        n782 = property class="App"() -> ("App.Kind"=w1646:T38)  [unwired: 2 in, 2 out]
        n783 = case shown="\"Run Time System\"" w1646 {
          frame Default {
          }
          frame "Run Time System" {
            n784 = control-ref of="This VI"() -> (w1653:refnum<vi>)
            n785 = invoke class="VI" method="FP.Close"(reference=w1653) -> ()  [unwired: 2 in, 3 out]
          }
        }
      }
      frame "Cfg - Init" {
        (unwired) "Direct T-Type Thermocouple" ("Sensor")
        n786 = Unbundle By Name(w1667) -> ("Config"=w1668:T16, "System Type"=w1655:T15)
        n787 = disable-structure shown="Disabled" {
          frame Disabled {
            n788 = Current VI's Path() -> (path=w1732:path)
            n789 = call "Set Window Title using Path.vi"("VI path"=w1732, "File Path"=path "" ("Sensor Config Path"), "Title"="Sensor Configuration") -> ()  [unwired: 12 in, 1 out]
          }
          frame Enabled {
          }
        }
        n790 = case shown="\"Standard 8TC\"" w1655 {
          tunnel: [w1674 w1696 w1718] -> w1665
          tunnel: [w1672 w1694 w1716] -> w1663
          tunnel: ["test.std" ("Config Name") "test.8TC" ("Config Name") "test.def" ("Config Name")] -> w1654
          frame "Standard", Default {
            n791 = for {
              tunnel: T20 {"Channel"="", "Type"="", "Acquire"=FALSE, "Name"="", "Sensor"="", "Data Index"=0} ("Channel") -> [w1681]
              tunnel: string[] ["9221_AI-00", "9221_AI-01", "9221_AI-02", "9221_AI-03", "9221_AI-04", "9221_AI-05", "9221_AI-06", "9221_AI-07", "9205_AI-00", "9205_AI-01", "9205_AI-02", "9205_AI-03", "9205_AI-04", "9205_AI-05", "9205_AI-06", "9205_AI-07", "9208_AI-00", "9208_AI-01", "9208_AI-02", "9208_AI-03", "9208_AI-04", "9208_AI-05", "9208_AI-06", "9208_AI-07", "9211_TC-00", "9211_TC-01", "9211_TC-02", "9211_TC-03", "9411_CTR-0"] ("Strings []") -> [w1678] mode=indexing
              tunnel: [w1680] -> w1674 mode=indexing
              tunnel: [T23 {"Channel Acquired?"=FALSE, "RMS?"=FALSE, "Pk-Pk"=FALSE, "Frequency"=FALSE, "EU High Limit 1"=0.0, "EU Low Limit 1"=0.0, "EU High Limit 2"=0.0, "EU Low Limit 2"=0.0, "RMS High Limit"=0.0, "RMS Low Limit"=0.0, "Pk-Pk High Limit "=0.0, "Pk-Pk Low Limit"=0.0, "Frequency High Limit"=0.0, "Frequency Low Limit"=0.0} ("Test Limit")] -> w1672 mode=indexing
              i -> [w1675]
              n792 = case shown="24..27" w1675 {
                tunnel: ["Direct Connection" ("Sensor") "Direct Connection" ("Sensor") "Direct Connection" ("Sensor") "Direct Connection" ("Sensor") "Direct Connection" ("Sensor")] -> w1677
                tunnel: ["0-60 VDC" ("Sensor") "0-10 VDC" ("Sensor") "0-20 mA" ("Sensor") "T-Type" ("Sensor") "Counter" ("Sensor")] -> w1676
                frame 0..7, Default {
                }
                frame 8..15 {
                }
                frame 16..23 {
                }
                frame 24..27 {
                }
                frame 28 {
                }
              }
              n793 = Bundle By Name(cluster=w1681, "Channel"=w1678, "Type"=w1676, "Sensor"=w1677, "Data Index"=w1675) -> (w1680:T20)
            }
          }
          frame "Standard 8TC" {
            n794 = for {
              tunnel: T20 {"Channel"="", "Type"="", "Acquire"=FALSE, "Name"="", "Sensor"="", "Data Index"=0} ("Channel") -> [w1703]
              tunnel: string[] ["9221_AI-00", "9221_AI-01", "9221_AI-02", "9221_AI-03", "9221_AI-04", "9221_AI-05", "9221_AI-06", "9221_AI-07", "9205_AI-00", "9205_AI-01", "9205_AI-02", "9205_AI-03", "9205_AI-04", "9205_AI-05", "9205_AI-06", "9205_AI-07", "9205_AI-22A", "9205_AI-23A", "9208_AI-00", "9208_AI-01", "9208_AI-02", "9208_AI-03", "9208_AI-04", "9208_AI-05", "9208_AI-06", "9208_AI-07", "9211-1_TC-00", "9211-1_TC-01", "9211-1_TC-02", "9211-1_TC-03", "9211-2_TC-00", "9211-2_TC-01", "9211-2_TC-02", "9211-2_TC-03", "9411_CTR-0"] ("Strings []") -> [w1700] mode=indexing
              tunnel: [w1702] -> w1696 mode=indexing
              tunnel: [T23 {"Channel Acquired?"=FALSE, "RMS?"=FALSE, "Pk-Pk"=FALSE, "Frequency"=FALSE, "EU High Limit 1"=0.0, "EU Low Limit 1"=0.0, "EU High Limit 2"=0.0, "EU Low Limit 2"=0.0, "RMS High Limit"=0.0, "RMS Low Limit"=0.0, "Pk-Pk High Limit "=0.0, "Pk-Pk Low Limit"=0.0, "Frequency High Limit"=0.0, "Frequency Low Limit"=0.0} ("Test Limit")] -> w1694 mode=indexing
              i -> [w1697]
              n795 = case shown="34" w1697 {
                tunnel: ["Direct Connection" ("Sensor") "Direct Connection" ("Sensor") "Direct Connection" ("Sensor") "Direct Connection" ("Sensor") "Direct Connection" ("Sensor")] -> w1699
                tunnel: ["0-60 VDC" ("Sensor") "0-10 VDC" ("Sensor") "0-20 mA" ("Sensor") "T-Type" ("Sensor") "Counter" ("Sensor")] -> w1698
                frame 0..7, Default {
                }
                frame 8..17 {
                }
                frame 18..25 {
                }
                frame 26..33 {
                }
                frame 34 {
                }
              }
              n796 = Bundle By Name(cluster=w1703, "Channel"=w1700, "Type"=w1698, "Sensor"=w1699, "Data Index"=w1697) -> (w1702:T20)
            }
          }
          frame "Deformation" {
            n797 = for {
              tunnel: T20 {"Channel"="", "Type"="", "Acquire"=FALSE, "Name"="", "Sensor"="", "Data Index"=0} ("Channel") -> [w1725]
              tunnel: string[] ["9205/0_AI-00", "9205/0_AI-01", "9205/0_AI-02", "9205/0_AI-03", "9205/0_AI-04", "9205/0_AI-05", "9205/0_AI-06", "9205/0_AI-07", "9205/0_AI-08", "9205/0_AI-09", "9205/0_AI-10", "9205/0_AI-11", "9205/0_AI-12", "9205/0_AI-13", "9205/0_AI-14", "9205/0_AI-15", "9205/0_AI-16", "9205/0_AI-17", "9205/0_AI-18", "9205/0_AI-19", "9205/0_AI-20", "9205/0_AI-21", "9205/0_AI-22", "9205/0_AI-23", "9205/0_AI-24", "9205/0_AI-25", "9205/0_AI-26", "9205/0_AI-27", "9205/0_AI-28", "9205/0_AI-29", "9205/0_AI-30", "9205/0_AI-31", "9205/1_AI-00", "9205/1_AI-01", "9205/1_AI-02", "9205/1_AI-03", "9205/1_AI-04", "9205/1_AI-05", "9205/1_AI-06", "9205/1_AI-07", "9205/1_AI-08", "9205/1_AI-09", "9205/1_AI-10", "9205/1_AI-11", "9205/1_AI-12", "9205/1_AI-13", "9205/1_AI-14", "9205/1_AI-15", "9205/1_AI-16", "9205/1_AI-17", "9205/1_AI-18", "9205/1_AI-19", "9205/1_AI-20", "9205/1_AI-21", "9205/1_AI-22", "9205/1_AI-23", "9205/1_AI-24", "9205/1_AI-25", "9205/1_AI-26", "9205/1_AI-27", "9205/1_AI-28", "9205/1_AI-29", "9205/1_AI-30", "9205/1_AI-31", "9205/2_AI-00", "9205/2_AI-01", "9205/2_AI-02", "9205/2_AI-03", "9205/2_AI-04", "9205/2_AI-05", "9205/2_AI-06", "9205/2_AI-07", "9205/2_AI-08", "9205/2_AI-09", "9205/2_AI-10", "9205/2_AI-11", "9205/2_AI-12", "9205/2_AI-13", "9205/2_AI-14", "9205/2_AI-15", "9205/2_AI-16", "9205/2_AI-17", "9205/2_AI-18", "9205/2_AI-19", "9205/2_AI-20", "9205/2_AI-21", "9205/2_AI-22", "9205/2_AI-23", "9205/2_AI-24", "9205/2_AI-25", "9205/2_AI-26", "9205/2_AI-27", "9205/2_AI-28", "9205/2_AI-29", "9205/2_AI-30", "9205/2_AI-31", "9220_AI-00", "9220_AI-01", "9220_AI-02", "9220_AI-03", "9220_AI-04", "9220_AI-05", "9220_AI-06", "9220_AI-07", "9220_AI-08", "9220_AI-09", "9220_AI-10", "9220_AI-11", "9220_AI-12", "9220_AI-13", "9220_AI-14", "9220_AI-15", "9208_AI-00", "9208_AI-01", "9208_AI-02", "9208_AI-03", "9208_AI-04", "9208_AI-05", "9208_AI-06", "9208_AI-07", "9211_TC-00", "9211_TC-01", "9211_TC-02", "9211_TC-03"] ("appended array") -> [w1722] mode=indexing
              tunnel: [w1724] -> w1718 mode=indexing
              tunnel: [T23 {"Channel Acquired?"=FALSE, "RMS?"=FALSE, "Pk-Pk"=FALSE, "Frequency"=FALSE, "EU High Limit 1"=0.0, "EU Low Limit 1"=0.0, "EU High Limit 2"=0.0, "EU Low Limit 2"=0.0, "RMS High Limit"=0.0, "RMS Low Limit"=0.0, "Pk-Pk High Limit "=0.0, "Pk-Pk Low Limit"=0.0, "Frequency High Limit"=0.0, "Frequency Low Limit"=0.0} ("Test Limit")] -> w1716 mode=indexing
              i -> [w1719]
              n798 = case shown="120..123" w1719 {
                tunnel: ["Direct Connection" ("Sensor") "Direct Connection" ("Sensor") "Direct Connection" ("Sensor")] -> w1721
                tunnel: ["0-10 VDC" ("Sensor") "0-20 mA" ("Sensor") "T-Type" ("Sensor")] -> w1720
                frame 0..111, Default {
                }
                frame 112..119 {
                }
                frame 120..123 {
                }
              }
              n799 = Bundle By Name(cluster=w1725, "Channel"=w1722, "Type"=w1720, "Sensor"=w1721, "Data Index"=w1719) -> (w1724:T20)
            }
          }
        }
        n800 = local write "Config Name:"(w1654) -> ()
        n801 = Bundle By Name(cluster=w1668, "Channels"=w1665, "DAQ Settings.Auto Save"=TRUE, "Test Limits"=w1663, "DAQ Settings.Log File Type"=Log_File_Type."Basic", "Data Base Path"=path "c:/Data", "DAQ Settings.Trigger Type"=T10."Manual", "DAQ Settings.Sample Rate"=10.0, "DAQ Settings.Log Rate"=1.0 ("DAQ Settings.Sample Rate"), "DAQ Settings.Save Mode"=T8."Single File") -> (w1669:T16)
        n802 = Bundle By Name(cluster=w1667, "Config"=w1669, "Config Saved"=w1669) -> (w1666:T28)
      }
      frame "Cfg - Load Sensors" {
        n803 = Unbundle By Name(w1742) -> ("Calibration Path"=w1735:path)
        n804 = call "Open Sensor Library.vi"("Sensor Library Path"=w1735) -> ("Sensors Info"=w1740:T26[], "Error?"=w1736:bool)  [unwired: 4 in, 1 out]
        n805 = case shown="True" w1736 {
          tunnel: [string[] ["Cfg - Sort Sensors", "Cfg - Add Default Sensors"] string[] ["Exit"]] -> w1739
          frame False {
          }
          frame True {
            n806 = One Button Dialog(message="Could not find sensor file.", button name ("OK")="Close Program") -> ()  [unwired: 1 out]
          }
        }
        n807 = call "Insert Multiple Events.vi"("Events to Insert"=w1739, "Event queue in"=w1738) -> ("Event queue out"=w1737:string[])  [unwired: 5 in]
        n808 = Bundle By Name(cluster=w1742, "Sensors"=w1740) -> (w1741:T28)
      }
      frame "Cfg - Sort Sensors" {
        # "Order sensor list.  Sort text, then numbers, then put together."
        n809 = Unbundle By Name(w1760) -> ("Sensors"=w1747:T26[])
        n810 = for {
          tunnel: w1747 -> [w1771] mode=indexing
          tunnel: [w1771] -> w1750 mode=indexing if=w1773
          tunnel: [w1771] -> w1751 mode=indexing if=w1772
          n811 = Unbundle By Name(w1771) -> ("Sensor Name"=w1774:string)
          n812 = call "Check if Number"("String IN"=w1774) -> ("Is a Number?"=w1773:bool)  [unwired: 10 in]
          n813 = Not(x=w1773) -> (.not. x?=w1772:bool)
        }
        n814 = for {
          tunnel: w1751 -> [w1767] mode=indexing
          tunnel: [w1766] -> w1757 mode=indexing
          n815 = Unbundle By Name(w1767) -> ("Sensor Name"=w1766:string)
        }
        n816 = for {
          tunnel: w1750 -> [w1765] mode=indexing
          tunnel: [w1764] -> w1749 mode=indexing
          n817 = Unbundle By Name(w1765) -> ("Sensor Name"=w1764:string)
        }
        n818 = Decimal String To Number(string=w1749) -> (number=w1748:i32[])  [unwired: 2 in, 1 out]
        n819 = call-poly <userlib>:"Sort Array__ogtk.vi"("Array in"=w1757) -> ("Sorted Pointers"=w1756:i32[])  [unwired: 9 in, 1 out]
        n820 = call-poly <userlib>:"Sort Array__ogtk.vi"("Array in"=w1748) -> ("Sorted Pointers"=w1755:i32[])  [unwired: 9 in, 1 out]
        n821 = for {
          tunnel: w1756 -> [w1769] mode=indexing
          tunnel: w1751 -> [w1770]
          tunnel: [w1768] -> w1754 mode=indexing
          n822 = Index Array(array=w1770, index=w1769) -> (element=w1768:T26)
        }
        n823 = for {
          tunnel: w1755 -> [w1762] mode=indexing
          tunnel: w1750 -> [w1763]
          tunnel: [w1761] -> w1753 mode=indexing
          n824 = Index Array(array=w1763, index=w1762) -> (element=w1761:T26)
        }
        n825 = Build Array (concatenate)(w1754, w1753) -> (w1752:T26[])
        n826 = Bundle By Name(cluster=w1760, "Sensors"=w1752) -> (w1759:T28)
      }
      frame "Cfg - Add Default Sensors" {
        w1775 = "Direct Connection"
        n827 = Unbundle By Name(w1784) -> ("Sensors"=w1778:T26[])
        n828 = for {
          tunnel: w1778 -> [w1799] mode=indexing
          tunnel: [w1798] -> w1777 mode=indexing
          n829 = Unbundle By Name(w1799) -> ("Sensor Name"=w1798:string)
        }
        n830 = Search 1D Array(1D array=w1777, element=w1775) -> (index of element=w1776:i32)  [unwired: 1 in]
        n831 = case shown="-1" w1776 {
          selector: w1776 -> [w1785 _]
          tunnel: w1778 -> [w1789 w1797]
          tunnel: [w1790 w1793] -> w1779
          tunnel: w1775 -> [_ w1792]
          frame Default {
            # "Default sensor exists, but not might not be at the top, so move it there."
            n832 = Delete From Array(array=w1789, length=0, index=w1785) -> (deleted portion=w1787:T26[], array with subset deleted=w1788:T26[])
            n833 = Insert Into Array(array=w1788, index=0, new element=w1787) -> (w1790:T26[])
          }
          frame -1 {
            # "Default sensor dosn't exist, so add them to the top of the list."
            n834 = Bundle By Name(cluster=T26 {"Sensor Name"="", "Sensor Info"={"Manufacturer"="", "Model"="", "Serial Number"=""}, "Last Cal Info"={"Last Calibration Date"=0.0, "Calibrator"="", "Cal Duration"=0}, "Voltage Range"={"High Limit"=0.0, "Low Limit"=0.0}, "EGU Range"={"High Limit"=0.0, "Low Limit"=0.0}, "Units"="", "Calibration Type"=enum."Calibrate Analog", "EGU List"=[], "Voltage List"=[], "Coefficients"=[], "Order"=0, "Algorithm"=enum."SVD", "Max Error % of Full Scale"=0.0, "Max Mean Squared Error"=0.0, "Use Error %"=FALSE, "Use MSE"=FALSE, "Allow Manual Entry"=FALSE, "Max Stability Error"=0.0, "Max Error % of Reading"=0.0, "Use Error % of Reading"=FALSE} ("Sensor Description"), "Sensor Name"=w1792) -> (w1795:T26)
            n835 = Insert Into Array(array=w1797, index=0, new element=w1795) -> (w1793:T26[])
          }
        }
        n836 = call "Insert Multiple Events.vi"("Events to Insert"=string[] [], "Event queue in"=w1782) -> ("Event queue out"=w1781:string[])  [unwired: 5 in]
        n837 = Bundle By Name(cluster=w1784, "Sensors"=w1779) -> (w1783:T28)
      }
      frame "Cfg - Store Channel Group" {
        n838 = Unbundle By Name(w1802) -> ("Config"=w1803:T16, "Channel Display"=w1804:T11)
        n839 = call "Store Channel Display.vi"("Channels in"=w1803, "Channel Display"=w1804) -> ("Channels out"=w1805:T16)  [unwired: 13 in]
        n840 = Bundle By Name(cluster=w1802, "Config"=w1805) -> (w1801:T28)
      }
      frame "Cfg - Update Channel Group" {
        n841 = Unbundle By Name(w1808) -> ("Sensors"=w1809:T26[], "Config.Channels"=w1810:T20[], "Config.Graph Settings"=w1813:T22)
        n842 = call "Update Channel Display.vi"("Sensors"=w1809, "Channels"=w1810, "Config.Graph Settings"=w1813) -> ("Graph Settings"=w1812:T22, "Sensors 2"=w1811:T11)  [unwired: 11 in]
        n843 = local write "Sensors"(w1811) -> ()
        n844 = Bundle By Name(cluster=w1808, "Channel Display"=w1811, "Config.Graph Settings"=w1812) -> (w1807:T28)
      }
      frame "Cfg - Check for Sensor Select" {
        n845 = Unbundle By Name(w1820) -> ("Channel Display"=w1823:T11)
        n846 = for {
          tunnel: w1823 -> [w1838] mode=indexing
          tunnel: [w1837] -> w1816
          tunnel: [w1836] -> w1815
          tunnel: [w1835] -> w1814
          i -> [w1835]
          stop <- w1837 stop-if-true
          n847 = Unbundle By Name(w1838) -> ("Sensor"=w1836:string, "Chg Sensor"=w1837:bool)
        }
        n848 = case shown="True" w1816 {
          tunnel: [-1 ("index of element") w1829] -> w1821
          tunnel: [string[] [] ("Events to Insert") w1828] -> w1822
          tunnel: w1815 -> [_ w1827]
          tunnel: w1814 -> [_ w1826]
          frame False {
          }
          frame True {
            n849 = case shown="\"Direct T-Type Thermocouple\"" w1827 {
              tunnel: [w1830 -1 ("index of element")] -> w1829
              tunnel: [string[] ["Cfg - Change Sensor", "Cfg - Clear Change Sensor Buttons", "Cfg - Store Channel Group", "Cfg - Update Channel Group", "Cfg - Save"] ("Events to Insert") string[] ["Cfg - Clear Change Sensor Buttons"] ("Events to Insert")] -> w1828
              tunnel: w1826 -> [w1830 _]
              frame Default {
              }
              frame "Direct T-Type Thermocouple" {
                n850 = One Button Dialog(message="Thermocouple Channels cannot\nhave sensors assigned to them.") -> ()  [unwired: 1 in, 1 out]
              }
            }
          }
        }
        n851 = Bundle By Name(cluster=w1820, "Channel Select"=w1821) -> (w1819:T28)
        n852 = call "Insert Multiple Events.vi"("Events to Insert"=w1822, "Event queue in"=w1817) -> ("Event queue out"=w1818:string[])  [unwired: 5 in]
      }
      frame "Cfg - Check for Calibrate" {
        n853 = Unbundle By Name(w1845) -> ("Channel Display"=w1848:T11)
        n854 = for {
          tunnel: w1848 -> [w1866] mode=indexing
          tunnel: [w1865] -> w1841
          tunnel: [w1864] -> w1840
          tunnel: [w1863] -> w1839
          i -> [w1863]
          stop <- w1865 stop-if-true
          n855 = Unbundle By Name(w1866) -> ("Sensor"=w1864:string, "Cal"=w1865:bool)
        }
        n856 = case shown="True" w1841 {
          tunnel: [-1 ("index of element") w1854] -> w1846
          tunnel: [string[] [] ("Events to Insert") w1853] -> w1847
          tunnel: w1839 -> [_ w1852]
          tunnel: w1840 -> [_ w1851]
          frame False {
          }
          frame True {
            n857 = case shown="Default" w1851 {
              tunnel: [string[] ["Cfg - Store Channel Group", "Cfg - Calibrate Sensor", "Cfg - Clear Calibrate Buttons", "Cfg - Update Channel Group"] ("Events to Insert") string[] ["Cfg - Clear Calibrate Buttons"] ("Events to Insert") string[] ["Cfg - Clear Calibrate Buttons"] ("Events to Insert")] -> w1853
              tunnel: [w1855 -1 ("index of element") -1 ("index of element")] -> w1854
              tunnel: w1852 -> [w1855 _ _]
              frame Default {
              }
              frame "Direct Connection" {
                n858 = One Button Dialog(message="This sensor type is fixed and\ncannot be calibrated.") -> ()  [unwired: 1 in, 1 out]
              }
              frame "Direct T-Type Thermocouple" {
                n859 = One Button Dialog(message="Thermocouple Channels cannot\nbe calibrated.") -> ()  [unwired: 1 in, 1 out]
              }
            }
          }
        }
        n860 = Bundle By Name(cluster=w1845, "Channel Select"=w1846) -> (w1844:T28)
        n861 = call "Insert Multiple Events.vi"("Events to Insert"=w1847, "Event queue in"=w1842) -> ("Event queue out"=w1843:string[])  [unwired: 5 in]
      }
      frame "Cfg - Change Sensor" {
        n862 = Unbundle By Name(w1869) -> ("Channel Display"=w1871:T11, "Channel Select"=w1870:i32, "Sensors"=w1880:T26[])
        n863 = Index Array(array=w1871, index=w1870) -> (element=w1872:T12)
        n864 = Unbundle By Name(w1872) -> ("Channel"=w1876:string, "Sensor"=w1878:string)
        n865 = call "Select Sensor.vi"("Channel"=w1876, "Sensor Name in"=w1878, "Sensors"=w1880) -> ("Sensor Name out"=w1877:string)  [unwired: 12 in]
        n866 = Bundle By Name(cluster=w1872, "Sensor"=w1877) -> (w1873:T12)
        n867 = Replace Array Subset(array=w1871, new element=w1873, index=w1870) -> (w1874:T11)
        n868 = for {
          tunnel: w1874 -> [w1883] mode=indexing
          tunnel: [w1882] -> w1875 mode=indexing
          tunnel: FALSE ("Chg Sensor") -> [w1881]
          n869 = Bundle By Name(cluster=w1883, "Chg Sensor"=w1881) -> (w1882:T12)
        }
        n870 = local write "Sensors"(w1875) -> ()
        n871 = Bundle By Name(cluster=w1869, "Channel Display"=w1875) -> (w1868:T28)
      }
      frame "Cfg - Calibrate Sensor" {
        n872 = Unbundle By Name(w1889) -> ("System Ref"=w1884:tag, "Sensors"=w1894:T26[], "Channel Display"=w1890:T11, "Channel Select"=w1898:i32, "Calibration Path"=w1899:path, "System Type"=w1885:T15)
        n873 = for {
          tunnel: w1894 -> [w1904] mode=indexing
          tunnel: [w1903] -> w1895 mode=indexing
          n874 = Unbundle By Name(w1904) -> ("Sensor Name"=w1903:string)
        }
        n875 = Index Array(array=w1890, index=w1898) -> (element=w1891:T12)
        n876 = Unbundle By Name(w1891) -> ("Sensor"=w1896:string)
        n877 = Search 1D Array(1D array=w1895, element=w1896) -> (index of element=w1897:i32)  [unwired: 1 in]
        n878 = Index Array(array=w1894, index=w1897) -> (element=w1892:T26)
        n879 = call "Calibrate Sensor.vi"("Sensor"=w1892, "System Ref"=w1884, "Channel Info"=w1891, "Cal Base Path"=w1899, "System Type"=w1885, "Channel index"=w1898) -> ("Sensor out"=w1902:T45, "OK Out"=w1901:bool)  [unwired: 8 in]
        n880 = Replace Array Subset(array=w1894, new element=w1902, index=w1897) -> (w1893:T26[])
        n881 = call "Insert Multiple Events.vi"("Insert all? (T)"=w1901, "Events to Insert"=string[] ["Cfg - Save Scaling Sensors"], "Event queue in"=w1886) -> ("Event queue out"=w1887:string[])  [unwired: 4 in]
        n882 = Bundle By Name(cluster=w1889, "Sensors"=w1893) -> (w1888:T28)
      }
      frame "Cfg - Add Sensor" {
        n883 = Unbundle By Name(w1909) -> ("Sensors"=w1910:T26[])
        n884 = call "Add Sensor.vi"("Sensors in"=w1910) -> ("Sensors out"=w1911:T26[])  [unwired: 13 in, 1 out]
        n885 = Bundle By Name(cluster=w1909, "Sensors"=w1911) -> (w1908:T28)
        n886 = call "Insert Multiple Events.vi"("Events to Insert"=string[] ["Cfg - Sort Sensors", "Cfg - Save Scaling Sensors"], "Event queue in"=w1905) -> ("Event queue out"=w1906:string[])  [unwired: 5 in]
      }
      frame "Cfg - Delete Sensor" {
        # "delete sensor from list"
        n887 = Unbundle By Name(w1916) -> ("Sensors"=w1917:T26[])
        n888 = call "Delete Sensor.vi"("Sensors"=w1917) -> ("Sensors out"=w1918:T27)  [unwired: 14 in]
        n889 = call "Insert Multiple Events.vi"("Events to Insert"=string[] ["Cfg - Sort Sensors", "Cfg - Save Scaling Sensors", "Cfg - Update Channel Group"], "Event queue in"=w1912) -> ("Event queue out"=w1913:string[])  [unwired: 5 in]
        n890 = Bundle By Name(cluster=w1916, "Sensors"=w1918) -> (w1915:T28)
      }
      frame "Cfg - Clear Change Sensor Buttons" {
        n891 = Unbundle By Name(w1921) -> ("Channel Display"=w1923:T11)
        n892 = for {
          tunnel: w1923 -> [w1926] mode=indexing
          tunnel: [w1925] -> w1922 mode=indexing
          n893 = Bundle By Name(cluster=w1926, "Chg Sensor"=FALSE) -> (w1925:T12)
        }
        n894 = local write "Sensors"(w1922) -> ()
        n895 = Bundle By Name(cluster=w1921, "Channel Display"=w1922) -> (w1920:T28)
      }
      frame "Cfg - Clear Calibrate Buttons" {
        n896 = Unbundle By Name(w1929) -> ("Channel Display"=w1930:T11)
        n897 = for {
          tunnel: w1930 -> [w1934] mode=indexing
          tunnel: [w1933] -> w1931 mode=indexing
          n898 = Bundle By Name(cluster=w1934, "Cal"=FALSE ("Chg Sensor")) -> (w1933:T12)
        }
        n899 = local write "Sensors"(w1931) -> ()
        n900 = Bundle By Name(cluster=w1929, "Channel Display"=w1931) -> (w1928:T28)
      }
      frame "Cfg - Check for Changes" {
        n901 = Unbundle By Name(w1937) -> ("Config"=w1938:T16, "Config Saved"=w1939:T16)
        n902 = Not Equal?(x=w1938, y=w1939) -> (x != y?=w1940:bool)
        n903 = case shown="True" w1940 {
          tunnel: [string[] ["Exit"] ("Events to Insert") w1945] -> w1941
          frame False {
          }
          frame True {
            n904 = Two Button Dialog(message="Sensor Configuration has changed.\nDo you want to save changes?", 1:"No" ("F button name (\"Cancel\")"), 2:"Yes" ("T button name (\"OK\")")) -> (T button?=w1948:bool)
            n905 = Select(t=string[] ["Save", "Exit"] ("Events to Insert"), s=w1948, f=string[] ["Exit"] ("Events to Insert")) -> (s? t:f=w1945:string[])
          }
        }
        n906 = call "Insert Multiple Events.vi"("Events to Insert"=w1941, "Event queue in"=w1935) -> ("Event queue out"=w1936:string[])  [unwired: 5 in]
      }
      frame "Cfg - Save Scaling Sensors" {
        # "save scaling sensor values"
        n907 = Unbundle By Name(w1955) -> ("Calibration Path"=w1951:path, "Sensors"=w1956:T26[])
        n908 = Flatten To String(anything=w1956) -> (data string=w1957:string)  [unwired: 3 in, 2 out]
        n909 = call "Write Characters To File with Advisory Dialog Option and Error Out.vi"("file path (dialog if empty)"=w1951, "character string"=w1957, "advisory dialog? (display:T)"=FALSE) -> ()  [unwired: 11 in, 2 out]
        n910 = call "Insert Multiple Events.vi"("Events to Insert"=string[] [], "Event queue in"=w1953) -> ("Event queue out"=w1954:string[])  [unwired: 5 in]
      }
      frame "Cfg - Load Last Config" {
        n911 = Unbundle By Name(w1966) -> ("Config Dir"=w1961:path, "Config Name"=w1960:string, "Config Extension"=w1958:string)
        n912 = Build Path(base path=w1961, name or relative path=w1960) -> (appended path=w1959:path)
        n913 = call <vilib>:"Check if File or Folder Exists.vi"("path"=w1959) -> ("file or folder exists?"=w1962:bool)  [unwired: 8 in, 2 out]
        n914 = case shown="True" w1962 {
          tunnel: [string[] ["Cfg - Load", "Save App Config"] string[] ["Cfg - Save", "Save App Config"]] -> w1967
          tunnel: w1966 -> [w1968 w1976]
          tunnel: [w1968 w1975] -> w1965
          tunnel: w1958 -> [_ w1973]
          frame True {
          }
          frame False {
            # "Config doesn't exist, so create new one."
            n915 = Match Pattern(string=w1973, regular expression="*") -> (after substring=w1972:string)  [unwired: 1 in, 3 out]
            n916 = Concatenate Strings("temporary" ("string"), w1972) -> (w1970:string)
            n917 = Bundle By Name(cluster=w1976, "Config Name"=w1970) -> (w1975:T28)
          }
        }
        n918 = call "Insert Multiple Events.vi"("Events to Insert"=w1967, "Event queue in"=w1963) -> ("Event queue out"=w1964:string[])  [unwired: 5 in]
      }
      frame "Cfg - Load" {
        n919 = Unbundle By Name(w1987) -> ("Config"=w1981:T16, "Config Dir"=w1983:path, "Config Name"=w1978:string)
        n920 = Build Path(base path=w1983, name or relative path=w1978) -> (appended path=w1982:path)
        n921 = Read from Binary File(5:w1981, 11:w1982) -> (0:w1980:errorcluster, 2:w1979:T16)  [unwired: 4 in, 2 out]
        n922 = case shown="No Error" w1980 {
          tunnel: w1987 -> [w2001 w2002]
          tunnel: [w2000 w2002] -> w1986
          tunnel: [string[] ["Cfg - Update Channel Group", "Cfg - Update DAQ Table", "Save App Config"] ("event queue out") string[] [] ("event queue out")] -> w1989
          tunnel: w1979 -> [w1991 _]
          tunnel: w1978 -> [w1990 _]
          frame No Error {
            w1994 = T30."Disabled and Grayed Out" ("Disabled")
            n923 = Unbundle By Name(w1991) -> ("Header"=w1996:T21, "Data Base Path"=w1992:path)
            n924 = local write "Changes Latch"(TRUE ("Changes Latch")) -> ()
            n925 = Cluster To Array(cluster=w1996) -> (array=w1999:string[])
            n926 = property on="Revert" class="Bool"("DisabledEnum"=w1994) -> ()  [unwired: 2 in, 2 out]
            n927 = property on="Save" class="Bool"("DisabledEnum"=w1994) -> ()  [unwired: 2 in, 2 out]
            n928 = Build Array(w1999) -> (w1998:string[][])
            n929 = Transpose 2D Array(2D array=w1998) -> (transposed array=w1997:string[][])
            n930 = local write "Header Table:"(w1997) -> ()
            n931 = local write "Data Base Path:"(w1992) -> ()
            n932 = Bundle By Name(cluster=w2001, "Config"=w1991) -> (w2000:T28)
            "Config Name:" <- w1990
          }
          frame Error {
          }
        }
        n933 = call "Insert Multiple Events.vi"("Insert all? (T)"=TRUE ("Insert?"), "Events to Insert"=w1989, "Event queue in"=w1984) -> ("Event queue out"=w1985:string[])  [unwired: 4 in]
      }
      frame "Cfg - Save" {
        n934 = Unbundle By Name(w2013) -> ("Config Saved"=w2017:T16, "Config Dir"=w2007:path, "Config Name"=w2004:string, "Config"=w2014:T16, "Channel Display"=w2015:T11, "Changes?"=w2019:bool)  [unwired: 1 out]
        n935 = call "Store Channel Display.vi"("Channels in"=w2014, "Channel Display"=w2015) -> ("Channels out"=w2008:T16)  [unwired: 13 in]
        n936 = Build Path(base path=w2007, name or relative path=w2004) -> (appended path=w2006:path)
        n937 = Write to Binary File(file (use dialog)=w2006, data=w2008) -> (error out=w2005:errorcluster)  [unwired: 4 in, 2 out]
        n938 = case shown="No Error" w2005 {
          tunnel: [w2025 w2027] -> w2016
          tunnel: w2008 -> [w2025 _]
          tunnel: w2017 -> [_ w2027]
          tunnel: [FALSE ("Changes?") w2026] -> w2018
          tunnel: w2019 -> [w2022 w2026]
          tunnel: [w2022 w2026] -> w2009
          tunnel: w2004 -> [w2021 _]
          frame No Error {
            w2023 = T30."Disabled and Grayed Out" ("Disabled")
            n939 = local write "Config Name:"(w2021) -> ()
            n940 = property on="Save" class="Bool"("DisabledEnum"=w2023) -> ()  [unwired: 2 in, 2 out]
            n941 = property on="Revert" class="Bool"("DisabledEnum"=w2023) -> ()  [unwired: 2 in, 2 out]
          }
          frame Error {
          }
        }
        "Changes Latch" <- w2009
        n942 = Bundle By Name(cluster=w2013, "Config Saved"=w2016, "Changes?"=w2018) -> (w2012:T28)
        n943 = call "Insert Multiple Events.vi"("Events to Insert"=string[] ["Save App Config"], "Event queue in"=w2010) -> ("Event queue out"=w2011:string[])  [unwired: 5 in]
      }
      frame "Cfg - Clear" {
        w2028 = T30."Disabled and Grayed Out" ("Disabled")
        w2035 = string[][] [] ("Header Table")
        n944 = local write "Config Name:"("" ("Config Name")) -> ()
        n945 = local write "Header Table:"(w2035) -> ()
        n946 = local write "DAQ Table"(w2035) -> ()
        n947 = property on="Save" class="Bool"("DisabledEnum"=w2028) -> ()  [unwired: 2 in, 2 out]
        n948 = property on="Revert" class="Bool"("DisabledEnum"=w2028) -> ()  [unwired: 2 in, 2 out]
        n949 = call "Insert Single Event.vi"("Insert?"=TRUE, "Event to insert"="Cfg - Init", "Event queue in"=w2029) -> ("Event queue out"=w2030:string[])  [unwired: 4 in]
        n950 = Bundle By Name(cluster=w2032, "Config"=T16 {"DAQ Settings"={"Trigger Type"=enum."Manual", "Trigger Samples"=0, "Pretrigger Samples"=0, "Trigger Interval"=0.0, "Time Units"=FALSE, "Auto Save"=FALSE, "Sample Rate"=0.0, "Select Analog"=FALSE, "Trigger Value"=0.0, "Trigger Stop Method"=enum."Use Samples Value to Stop Trigger", "Rate Sec/Min"=FALSE, "Save Mode"=enum."Single File", "File Size Limit"=0.0, "Log File Type"=enum."Basic", "Trigger Data Index"=0, "Log Rate"=7.0, "Rate Sec/Min (Log)"=FALSE, "Sample Rate (S/s)"=0.0, "Log Rate (S/s)"=0.0}, "Channels"=[], "Header"={"CA Number"="", "Test Name"="", "Serial Number"="", "Technician"=""}, "Graph Settings"={"Graph Labels"=[], [], [], [], [], [], [], [], [], [], [], [], [], "Graph Toggles"=[], "Axis Toggles"=[], "Graph Range"=enum."1"}, "Test Limits"=[], "All Type Info"=[], "Save Mode"=enum."New File at Midnight", "Data Base Path"=path ""}) -> (w2031:T28)
      }
      frame "Cfg - Update DAQ Table" {
        w2064 = i16 3 ("precision (6)")
        w2062 = ""
        n951 = Unbundle By Name(w2044) -> ("Config.DAQ Settings.Trigger Type"=w2048:T10, "Config.DAQ Settings.Time Units"=w2051:bool, "Config.DAQ Settings.Rate Sec/Min"=w2066:bool, "Config.DAQ Settings.Rate Sec/Min (Log)"=w2040:bool, "Config.DAQ Settings.Auto Save"=w2052:bool, "Config.DAQ Settings.Trigger Stop Method"=w2049:T18, "Config.DAQ Settings.Save Mode"=w2069:T8, "Config.DAQ Settings.File Size Limit"=w2070:dbl, "Config.DAQ Settings.Trigger Value"=w2053:dbl, "Config.DAQ Settings.Trigger Samples"=w2055:i32, "Config.DAQ Settings.Pretrigger Samples"=w2057:i32, "Config.DAQ Settings.Trigger Interval"=w2059:dbl, "Config.DAQ Settings.Sample Rate"=w2061:dbl, "Config.DAQ Settings.Log Rate"=w2039:dbl, "Config.Channels"=w2071:T20[], "Config.DAQ Settings.Trigger Data Index"=w2072:u32)
        n952 = Index Array(array=w2071, index=w2072) -> (element=w2073:T20)
        n953 = Unbundle By Name(w2073) -> ("Channel"=w2075:string, "Name"=w2076:string)
        n954 = Empty String/Path?(string/path=w2076) -> (empty?=w2074:bool)
        n955 = Select(t=w2075, s=w2074, f=w2076) -> (s? t:f=w2077:string)
        n956 = Number To Fractional String(number=w2053, precision (6)=w2064) -> (F-format string=w2054:string)  [unwired: 2 in]
        n957 = Number To Decimal String(number=w2055) -> (decimal integer string=w2056:string)  [unwired: 1 in]
        n958 = Number To Decimal String(number=w2057) -> (decimal integer string=w2058:string)  [unwired: 1 in]
        n959 = Number To Fractional String(number=w2059, precision (6)=w2064) -> (F-format string=w2060:string)  [unwired: 2 in]
        n960 = Number To Decimal String(number=w2061) -> (decimal integer string=w2063:string)  [unwired: 1 in]
        n961 = Number To Decimal String(number=w2039) -> (decimal integer string=w2038:string)  [unwired: 1 in]
        n962 = Not(x=w2066) -> (.not. x?=w2065:bool)
        n963 = Not(x=w2040) -> (.not. x?=w2041:bool)
        n964 = Not(x=w2051) -> (.not. x?=w2050:bool)
        n965 = local write "Trigger Stop Method"(w2049) -> ()
        n966 = Build Array(w2062, w2077, w2054, w2056, w2058, w2060, w2062, w2063, w2038) -> (w2045:string[])
        n967 = local write "Minutes"(w2050) -> ()
        n968 = local write "Sample Min"(w2066) -> ()
        n969 = local write "Log Min"(w2040) -> ()
        n970 = local write "Trigger Type"(w2048) -> ()
        n971 = local write "Hours"(w2051) -> ()
        n972 = local write "Save Mode"(w2069) -> ()
        n973 = local write "Limit:"(w2070) -> ()
        n974 = local write "Sample Sec"(w2065) -> ()
        n975 = local write "Auto Save"(w2052) -> ()
        n976 = local write "Log Sec"(w2041) -> ()
        n977 = Build Array(w2045) -> (w2046:string[][])
        n978 = Transpose 2D Array(2D array=w2046) -> (transposed array=w2047:string[][])
        n979 = local write "DAQ Table"(w2047) -> ()
        n980 = call "Insert Single Event.vi"("Insert?"=TRUE, "Event to insert"="Cfg - Update Fields", "Event queue in"=w2042) -> ("Event queue out"=w2043:string[])  [unwired: 4 in]
      }
      frame "Cfg - Update Fields" {
        n981 = Unbundle By Name(w2079) -> ("Config.DAQ Settings.Trigger Type"=w2080:T10, "Config.DAQ Settings.Save Mode"=w2087:T8)
        n982 = case shown="\"Single File\", \"New File at Midnight\", Default" w2087 {
          tunnel: [FALSE TRUE] -> w2088
          frame "Single File", "New File at Midnight", Default {
          }
          frame "Segmented Files" {
          }
        }
        n983 = case shown="\"Timed\"" w2080 {
          tunnel: [w2091 w2093 w2095] -> w2081
          tunnel: [w2091 w2093 w2095] -> w2082
          tunnel: [w2091 w2092 w2095] -> w2083
          tunnel: [w2091 w2093 w2095] -> w2084
          tunnel: [w2091 w2092 TRUE] -> w2085
          tunnel: [w2091 w2093 w2095] -> w2086
          frame "Manual", Default {
            w2091 = TRUE
          }
          frame "Timed" {
            w2092 = FALSE
            w2093 = TRUE
          }
          frame "Analog Rising", "Analog Falling" {
            w2095 = FALSE
          }
        }
        n984 = property on="Hide Trig Ch" class="Bool"("Visible"=w2081) -> ()  [unwired: 2 in, 2 out]
        n985 = property on="Hide Trig Val" class="Bool"("Visible"=w2082) -> ()  [unwired: 2 in, 2 out]
        n986 = property on="Hide Trig Samples" class="Bool"("Visible"=w2083) -> ()  [unwired: 2 in, 2 out]
        n987 = property on="Hide Pretrig Smpls" class="Bool"("Visible"=w2084) -> ()  [unwired: 2 in, 2 out]
        n988 = property on="Hide Trig Int" class="Bool"("Visible"=w2085) -> ()  [unwired: 2 in, 2 out]
        n989 = property on="Hide Trig Stop" class="Bool"("Visible"=w2086) -> ()  [unwired: 2 in, 2 out]
        n990 = property on="Limit:" class="DigNum (strict)"("Visible"=w2088) -> ()  [unwired: 2 in, 2 out]
      }
      frame "Cfg - Import from CSV" {
        n991 = Unbundle By Name(w2103) -> ("Sensors"=w2098:T26[])
        n992 = call "File Dialog3"("pattern label"="*.csv") -> ("selected path"=w2096:path, "cancelled"=w2097:bool)  [unwired: 11 in, 2 out]
        n993 = case shown="False" w2097 {
          tunnel: [string[] ["Cfg - Sort Sensors", "Cfg - Save Scaling Sensors", "Cfg - Update Channel Group"] ("Events to Insert") string[] [] ("Events to Insert")] -> w2104
          tunnel: w2103 -> [w2111 w2113]
          tunnel: [w2110 w2113] -> w2102
          tunnel: w2098 -> [w2109 _]
          tunnel: w2096 -> [w2107 _]
          frame False {
            n994 = call "Import Sensors from CSV.vi"("CSV Path"=w2107, "Sensors"=w2109) -> ("Sensors OUT"=w2108:T26[])  [unwired: 9 in]
            n995 = One Button Dialog(message="Import complete!") -> ()  [unwired: 1 in, 1 out]
            n996 = Bundle By Name(cluster=w2111, "Sensors"=w2108) -> (w2110:T28)
          }
          frame True {
          }
        }
        n997 = call "Insert Multiple Events.vi"("Events to Insert"=w2104, "Event queue in"=w2100) -> ("Event queue out"=w2101:string[])  [unwired: 5 in]
      }
      frame "Cfg - Enable Tab" {
        n998 = property on="Main Tab" class="TabCtl (strict)"() -> ("Pages"=w2116:refnum<vi>[])  [unwired: 2 in, 2 out]
        n999 = Index Array(array=w2116, index=1) -> (element=w2117:refnum<vi>)
        n1000 = property class="Page"(reference=w2117, "PageEnb"=T31."Page Enabled" ("Page Enabled State")) -> ()  [unwired: 1 in, 2 out]
      }
      frame "Cfg - Disable Tab" {
        n1001 = property on="Main Tab" class="TabCtl (strict)"() -> ("Pages"=w2122:refnum<vi>[])  [unwired: 2 in, 2 out]
        n1002 = Index Array(array=w2122, index=1) -> (element=w2123:refnum<vi>)
        n1003 = property class="Page"(reference=w2123, "PageEnb"=T31."Page Disabled & Grayed" ("Page Enabled State")) -> ()  [unwired: 1 in, 2 out]
      }
    }
  }
